vi "ControlProgram5.8.vi"() -> ()   [LabVIEW 2016]
uses:
  <vilib>/Utility/miscctls.llb/LVPoint32TypeDef.ctl
  <vilib>/Platform/TimedLoop/XDataNode/timing_clust.ctl
  <vilib>/Platform/TimedLoop/XDataNode/nitl_modes.ctl
  <vilib>/Platform/TimedLoop/XDataNode/wakeup.ctl
  <vilib>/vision/Avi1.llb/AviRefnum.ctl
  <vilib>/Utility/error.llb/DialogType.ctl
  <vilib>/DAQmx/write.llb/DAQmx Write (Analog 1D DBL NChan 1Samp).vi
  <vilib>/DAQmx/read.llb/DAQmx Read (Analog 2D DBL NChan NSamp).vi
  <vilib>/Analysis/baseanly.llb/Mean (DBL).vi
  <vilib>/DAQmx/write.llb/DAQmx Write (Digital Bool 1Line 1Point).vi
  <vilib>/DAQmx/create/channels.llb/DAQmx Create Channel (DO-Digital Output).vi
  <vilib>/Instr/_visa.llb/VISA Configure Serial Port (Instr).vi
  <vilib>/DAQmx/create/channels.llb/DAQmx Create Channel (AI-Voltage-Basic).vi
  <vilib>/DAQmx/create/channels.llb/DAQmx Create Channel (AO-Voltage-Basic).vi
  <vilib>/DAQmx/configure/timing.llb/DAQmx Timing (Sample Clock).vi
  <vilib>/DAQmx/miscellaneous.llb/DAQmx Fill In Error Info.vi
  <vilib>/Utility/inputDevices.llb/mouseAcquire.vi
  <vilib>/Utility/inputDevices.llb/closeMouse.vi
  <vilib>/platform/TimedLoop/XDataNode/XDataNode.xnode
  <vilib>/Platform/TimedLoop/XDataNode/XDNodeRunTimeDep.lvlib
  <resource>/objmgr/daqmx.rc
  <vilib>/Analysis/NI_AALBase.lvlib
panel:
  out "Primary Video Display":T1(plugin-control)
  in  "Save file index":i32
  out "Flush Sample Start Time":u32=2111292881
  out "Sample flush time (s)":dbl=48.0
  in  "Inject Sample":bool
  out "Chart Freq (Hz)":dbl=500.0
  out "Cal values":T2={"AX alpha"=612.9626061060078, "BX alpha"=549.6584469744151, "AX kappa"=0.3485731373010688, "BX kappa"=0.3853424216291352, "AX offset"=-0.03900484438240665, "BX offset"=-0.11295550662085417, "AY alpha"=582.7562541114835, "BY alpha"=571.1587543790358, "AY kappa"=0.37498408087930674, "BY kappa"=0.36252029651198364, "AY offset"=-0.21125584642206058, "BY offset"=-0.12469077200400738}
  in  "Inject Pump 1":bool
  in  "Inject Pump 2":bool
  in  "Tab Control 2":T3(tab)
  in  "Force FB script":bool
  in  "Got ADig bead":bool
  in  "Move Cap. 2 (ADig Top)":bool
  in  "Dump beads":bool
  in  "Got DNA bead":bool
  in  "Flow on\ncap 2?":bool=TRUE
  in  "Flow on\ncap 1?":bool=TRUE
  in  "Flow on\ndump?":bool=TRUE
  in  "Raster set":i32=1
  in  "Fish After TA?":bool=TRUE
  in  "Delta after tether":dbl=1700.0
  in  "TA Cancel Save?":bool=TRUE
  in  "Min fish\ndelta (nm)":dbl=1425.0 min=0.0 max=5000.0 step=50.0
  in  "Max fish\ndelta (nm)":dbl=1900.0 min=0.0 max=5000.0 step=25.0
  in  "Fish Speed (ms)":i32=5000
  in  "Wait (ms)":i32=1500
  in  "# attempts":dbl=10.0
  in  "Cutoff force (pN)":dbl=4.5
  in  "Raster after\n tether?":bool=TRUE
  out "Tether":bool
  out "Attempt #":i32
  in  "Flow on\nwhile fish?":bool=TRUE
  in  "Flow on\nafter raster?":bool=TRUE
  in  "Offset raster set":i32
  in  "Offset @ Delta (nm)":dbl=1700.0
  in  "Cal @ Delta (nm)":dbl=2500.0
  in  "Cal stage position":i32=3
  out "Cal Final Sampling Rate":dbl=125000.0
  in  "Cal Averaging":i32=1
  in  "Wait before dip (s)":dbl=3.0
  in  "Start dipping after?":bool
  in  "Start trap delta (nm)":dbl=1700.0
  in  "Cancel dwell":bool=TRUE
  in  "Pause dwell":bool
  in  "Return position":dbl=3.0
  in  "Dip duration":dbl=15.0
  in  "Dip position":dbl=4.0
  in  "Dip":bool
  out "Dip time":i32
  in  "Stop":bool=TRUE
  in  "?":T4(tab)
  in  "Cal time (s)":dbl=5.0
  in  "Save N sets":bool
  in  "N sets":i32=200
  out "Cal sets to save":i32=500
  in  "Reset data stream":bool
  out "Buffer Overflow":bool
  out "Stage moving":bool
  in  "Comment":string
  in  "Raster scan":bool
  out "Saving":bool
  in  "Save cal":bool
  in  "Save Data":bool
  in  "Stop saving":bool
  out "Calibrating":bool
  out "Progress":dbl(slide) scale=0.0..100.0
  in  "Read Cal":bool
  in  "Fish":bool
  in  "Averaging Number":i32=1250
  out "Final Sampling Rate":dbl=100.0
  in  "Trap position (V)":cluster{"X":dbl, "Y":dbl}={"X"=3.9042624789680316, "Y"=0.2}
  in  "Trap delta (nm)":dbl=2500.0 min=0.0 max=5000.0 step=50.0
  in  "Fixed X":dbl=1.3
  in  "Fixed Y":dbl=1.8
  in  "Shutter 1 (B)":bool
  in  "Shutter 2 (A)":bool
  in  "Pulling direction":bool
  out "Raster scanning...":bool
  out "Current file name":path=path "D:/data/160111/160111_006.dat"
  in  "AX alpha":dbl=612.9626061060078 format="%#_3p"
  in  "BX alpha":dbl=549.6584469744151 format="%#_3g"
  in  "AX kappa":dbl=0.3485731373010688 format="%#_3g"
  in  "BX kappa":dbl=0.3853424216291352 format="%#_3g"
  in  "AX offset":dbl=-0.03900484438240665 format="%#_3g"
  in  "BX offset":dbl=-0.11295550662085417 format="%#_3g"
  in  "AY alpha":dbl=582.7562541114835 format="%#_3g"
  in  "BY alpha":dbl=571.1587543790358 format="%#_3g"
  in  "AY kappa":dbl=0.37498408087930674 format="%#_3g"
  in  "BY kappa":dbl=0.36252029651198364 format="%#_3g"
  in  "AY offset":dbl=-0.21125584642206058 format="%#_3g"
  in  "BY offset":dbl=-0.12469077200400738 format="%#_3g"
  out "Buffer status":u8(slide) scale=0.0..100.0
  in  "Target":bool
  in  "Set Current\nPos to (0,0,0)":bool
  in  "dump spot":string="Dump beads spot"
  in  "up flow spot":string="Upper flow spot"
  in  "low flow spot":string="Lower flow spot"
  in  "up cap":string="Upper capillary (ADig beads)"
  in  "bottom cap":string="Lower capillary (DNA beads)"
  in  "Move to Position 5":bool
  in  "Set Position 5":bool
  in  "Saved stage positions":dbl[][](array[numeric])=[[1.0, 0.0, 0.0, 0.0], [2.0, -0.13716, -3.21132, 0.01436], [3.0, 0.45, -0.73974, 0.005], [4.0, 0.45, -2.1978, 0.005], [5.0, 0.45, -2.63158, -0.02256]]
  in  "Set Position 2":bool
  in  "Move to Position 2":bool
  in  "Set Position 1":bool
  in  "Move to Position 1":bool
  in  "Set Position 4":bool
  in  "Move to Position 4":bool
  in  "Set Position 3":bool
  in  "Move to Position 3":bool
  out "Stage error":errorcluster
  in  "Clear Volume":bool
  out "Sample Flush Meter":u8(slide) scale=0.0..100.0
  out "Flushing Sample":bool
  in  "Flush Sample":bool
  in  "Normal \nRate (ul/hr)  3":dbl=100.0
  in  "Normal \nVolume (ul) 3":dbl=250.0
  in  "Normal \nVolume (ul) 2":dbl
  in  "Normal \nRate (ul/hr)":dbl
  in  "Normal \nVolume (ul)":dbl
  in  "Flush\nRate (ul/min)":dbl
  in  "Flush\nVolume (ul)":dbl
  in  "Flush \nRate (ul/min)  2":dbl
  in  "Flush Pump 2":bool
  in  "Flush\nVolume (ul)  2":dbl
  in  "Flush Pump 1":bool
  in  "Normal \nRate (ul/hr)  2":dbl
  in  "Write Wait":i32=1000
  in  "Flush \nRate (ul/min)  3":dbl=100.0
  in  "Flush\nVolume (ul)  3":dbl=80.0
  out "error out":errorcluster
  in  "Use Mouse to Move Trap?":bool
  in  "Pause Mouse/Mirror Connection":bool
  out "Reference Voltage":cluster{dbl, dbl}={0.0, -0.0}
  out "Saved voltage":cluster{dbl, dbl}={5.766666666666665, 1.45}
  out "Real Coordinates":cluster{"Horizontal":i32, "Vertical":i32}={"Horizontal"=897, "Vertical"=-1271}
  out "CoordinatesMousePressed":T5
  out "Sum error":dbl(knob) scale=-0.2..0.2
  out "Trap sep":waveform(dbl)[](graph)=[{"t0"=timestamp(4.489999999999949 s since 1904-01-01), "dt"=0.002, "Y"=[-1157.7639781743756, -1157.678951177374, -1157.7582331070425, -1157.7490409992681, -1157.8995617642552], "attributes"=variant("NI_ChannelName"=variant(string "T2 X"))}, {"t0"=timestamp(4.489999999999949 s since 1904-01-01), "dt"=0.002, "Y"=[-909.0775466981794, -909.1316439023619, -909.1322956759037, -909.1570630705896, -909.1264297140281], "attributes"=variant("NI_ChannelName"=variant(string "T2 Y"))}]
  in  "Set reading to\nsetpoint":bool
  in  "Offset Y (nm)":dbl format="%0.2f"
  in  "Offset X (nm)":dbl format="%0.2f"
  in  "Remove offsets":bool
  in  "Force Feedback":bool
  out "Feedback Output Voltage 2":cluster{dbl, dbl} {"?" format="%#_4g"; "?" format="%#_4g"}
  in  "Offset":cluster{"Off Y":dbl, "Off X":dbl}={"Off Y"=1.5, "Off X"=0.17}
  in  "Setpoint voltage":cluster{"SP Y":dbl, "SP X":dbl}={"SP Y"=0.6, "SP X"=0.0}
  in  "Feedback const":T6={"Ki_B_Y"=0.5, "Ki_B_X"=0.0, "Kp Y"=1.0, "Kp X"=0.0}
  out "Mean Trap Pos X 2 (nm)":dbl=-1157.769953044463 format="%0.2f"
  out "Mean Trp Pos Y 2 (nm)":dbl=-909.1249958122125 format="%0.2f"
  out "T2 X RMS (A)":dbl=0.7168002469275427 format="%0.2f"
  out "T2 Y RMS (A)":dbl=0.25997187037503383 format="%0.2f"
  in  "Scan range (nm)":dbl=425.0
  in  "Scan speed (nm/s)":dbl=100.0 min=0.0 max=100.0
  in  "Step size (nm)":dbl=1.0
  in  "Save scans":bool=TRUE
  in  "# scans":i32=1
  in  "Load param":bool
  in  "Scan Parameters":T7(array[cluster])=[{"Label"="Offset", "Scan range 1"=600.0, "Step size 1"=1.0, "Scan speed 1"=100, "# scans 2"=1}, {"Label"="Hairpin", "Scan range 1"=450.0, "Step size 1"=1.0, "Scan speed 1"=100, "# scans 2"=1}]
  in  "Trap delta\nafter (nm)":dbl=1550.0
  in  "Stop raster":bool
  out "Scan range (V)":dbl=0.47672462142456534
  out "Scan steps (mirror)":u64=425
  out "Scan increment (V)":dbl=0.0011217049915872126
  out "Time per step (ms)":dbl=10.0
  out "Total raster time (s)":dbl=8.5
  out "N sets to be saved":dbl=850.0
  in  "Zoom Factor":sgl=7.0
  in  "Center Point":cluster{"X":i32, "Y":i32}={"X"=335, "Y"=271}
  in  "Intensity Upper":dbl=88.0
  in  "Intensity Lower":dbl=66.0
  out "Window Size":cluster{"Height":i32, "Width":i32}
  in  "Image Index":dbl=1.0 min=1.0
  in  "Save Image":bool
  in  "Averaging":bool
  in  "Reset Averaging":bool
  in  "Save Video":bool
  in  "New Video File":bool
  in  "Video Index":dbl=1.0 min=1.0 step=1.0
  in  "Video Capture Rate (Hz)":dbl=30.0
  in  "Initial Window Size":cluster{"Width":i32, "Height":i32}={"Width"=884, "Height"=619}
  in  "Initial Window Position":cluster{"X Position":i32, "Y Position":i32}={"X Position"=796, "Y Position"=4}
  out "Window Position":cluster{"X Position":i32, "Y Position":i32}={"X Position"=40, "Y Position"=40}
  out "Path Out":path
  in  "Target coordinates":cluster{"X1":dbl, "Y1":dbl, "X2":dbl, "Y2":dbl}={"X1"=328.0, "Y1"=274.0, "X2"=368.0, "Y2"=314.0}
  in  "# Samples/channel (in)":i32=40000 format="%.2f"
  out "Buffer size\n(Samples/channel)":u32=511
  out "DAQ rate\n(Samples/s)":dbl=125000.0 format="%#_6p"
  out "# Samples/channel":i32=1250
  out "# Samples/channel/s":dbl=100.0
  out "AvailSampPerChan":u32=9
  out "Data update period (s/set)":dbl=0.01 format="%#_6p"
  out "AvailSampPerChan 2":u32=110
  in  "PC samp per channel":i32=1000
  in  "Sampling Rate":dbl=125000.0 format="%0.0p"
  in  "DAQ Rate2":dbl=1000000.0 format="%#_6p"
  out "Data period (s)":dbl=8e-06 format="%#_6p"
  in  "Save user params":bool
  in  "User":string(combo)
  in  "Load user params":bool
  in  "Tether break\nforce (pN)":dbl=1.0
  in  "Path":path=path "E:/Data"
  out "Mirror task":refnum<k21>
  in  "Conv X (nm/V)":dbl=891.5
  in  "Conv Y (nm/V)":dbl=505.7
  in  "Min value Y":dbl format="%.1g"
  in  "Max value Y":dbl=10.0 format="%.1f"
  in  "Min value X":dbl format="%0.1f"
  in  "Max value X":dbl=10.0 format="%.1f"
  in  "HWP1":string="Half waveplate 1: differential trap power"
  in  "HWP0":string="Half waveplate 0: total trap power"
  in  "Move 1":bool
  in  "\"Degrees\" 1":dbl
  in  "Move 0":bool
  in  "\"Degrees\" 0":dbl
  out "Deflection":T5
  in  "Sampling Rate":dbl=125000.0 format="%0.2f"
  in  "Averaging Number":i32=12500
  in  "DAQ Rate":dbl=1000000.0
  out "Final Sampling Rate":dbl
  in  "Tab Control":T8(tab)
  in  "Downsamp\nfact":dbl=250.0
  out "Bead sep":waveform(dbl)[](graph)=[{"t0"=timestamp(4.489999999999949 s since 1904-01-01), "dt"=0.002, "Y"=[8093.963535945606, 8103.1617772716045, 8385.72390184118, 8245.733099167523, 8154.925676756515], "attributes"=variant("NI_ChannelName"=variant(string "T2"))}, {"t0"=timestamp(4.489999999999949 s since 1904-01-01), "dt"=0.002, "Y"=[1717.924930434114, 1628.723007842151, 1787.6888378897193, 1598.475730715916, 1776.2517588078954], "attributes"=variant("NI_ChannelName"=variant(string "T1"))}]
  out "Force (pN)":waveform(dbl)[](graph)=[{"t0"=timestamp(4.489999999999949 s since 1904-01-01), "dt"=0.002, "Y"=[2821.5994183803123, 2824.8226375853515, 2923.3663028678166, 2874.5254578927593, 2842.869034836209], "attributes"=variant("NI_ChannelName"=variant(string "T2"))}, {"t0"=timestamp(4.489999999999949 s since 1904-01-01), "dt"=0.002, "Y"=[623.5850847499229, 591.0680427774053, 648.761979867749, 579.944408346982, 644.7436619059413], "attributes"=variant("NI_ChannelName"=variant(string "T1"))}]
  out "Mean force (pN)":dbl=1737.5286029210451 format="%0.2f"
  out "Force noise (pN)":dbl=26.83032703631318 format="%0.2f"
  out "Mean Bead Sep\n(nm)":dbl=4949.257225667222 format="%0.2f"
  out "Bead Sep Noise\n(A)":dbl=757.8078481959694 format="%0.2f"
  out "PSD 2":cluster{dbl[], dbl[]}(graph)
  out "PSD 1":cluster{dbl[], dbl[]}(graph)
  out "PSD 1 Sum":dbl(slide) scale=0.0..10.0
  out "PSD 2 Sum":dbl(slide) scale=0.0..10.0
  in  "Start":bool
  out "All signals":waveform(dbl)[](graph)=[{"t0"=timestamp(4.489999999999949 s since 1904-01-01), "dt"=0.002, "Y"=[0.0010396217068286443, 0.0010666908927528754, 0.001103298744846499, 0.0010651440823993424, 0.0010656596859401936], "attributes"=variant("NI_ChannelName"=variant(string "A y"))}, {"t0"=timestamp(4.489999999999949 s since 1904-01-01), "dt"=0.002, "Y"=[0.02000680227246931, 0.020097032918054827, 0.02003412926844257, 0.020136734401221615, 0.020087494249822452], "attributes"=variant("NI_ChannelName"=variant(string "A x"))}, {"t0"=timestamp(4.489999999999949 s since 1904-01-01), "dt"=0.002, "Y"=[-0.0014958587831537804, -0.0015046240440107857, -0.0014930229638311983, -0.001533240041751485, -0.0015262793936602433], "attributes"=variant("NI_ChannelName"=variant(string "B y"))}, {"t0"=timestamp(4.489999999999949 s since 1904-01-01), "dt"=0.002, "Y"=[0.0002901198559372817, 0.0002731049385577592, 0.00026511308349727467, 0.0002517073909711183, 0.0002916666665966012], "attributes"=variant("NI_ChannelName"=variant(string "B x"))}, {"t0"=timestamp(4.489999999999949 s since 1904-01-01), "dt"=0.002, "Y"=[-0.001511556786147372, -0.0015167122027053212, -0.0014612914746018214, -0.0014935128282145193, -0.0015064013696263116], "attributes"=variant("NI_ChannelName"=variant(string "A sum"))}, {"t0"=timestamp(4.489999999999949 s since 1904-01-01), "dt"=0.002, "Y"=[-0.0005242945138364382, -0.0005565158674093218, -0.000501095139248956, -0.0005771375336978897, -0.0005165613890095197], "attributes"=variant("NI_ChannelName"=variant(string "B sum"))}, {"t0"=timestamp(4.489999999999949 s since 1904-01-01), "dt"=0.002, "Y"=[0.0013303666019343777, 0.0014257418088905328, 0.0013368108726387405, 0.0013471217058124534, 0.0011782818123890176], "attributes"=variant("NI_ChannelName"=variant(string "Trap x"))}, {"t0"=timestamp(4.489999999999949 s since 1904-01-01), "dt"=0.002, "Y"=[0.0023382505474007294, 0.002231275652833831, 0.002229986798687363, 0.0021810103409340116, 0.002241586486003531], "attributes"=variant("NI_ChannelName"=variant(string "Trap y"))}]
  # "Bead Calibration"
  # "Y"
  # "X"
  # "Pump #1 Controls"
  # "Pump #2 Controls"
  # "Sample Pump Controls"
  # "Retract the pumps manually. Change it back to INFUSE when you're done. Suck it up, don't whine."
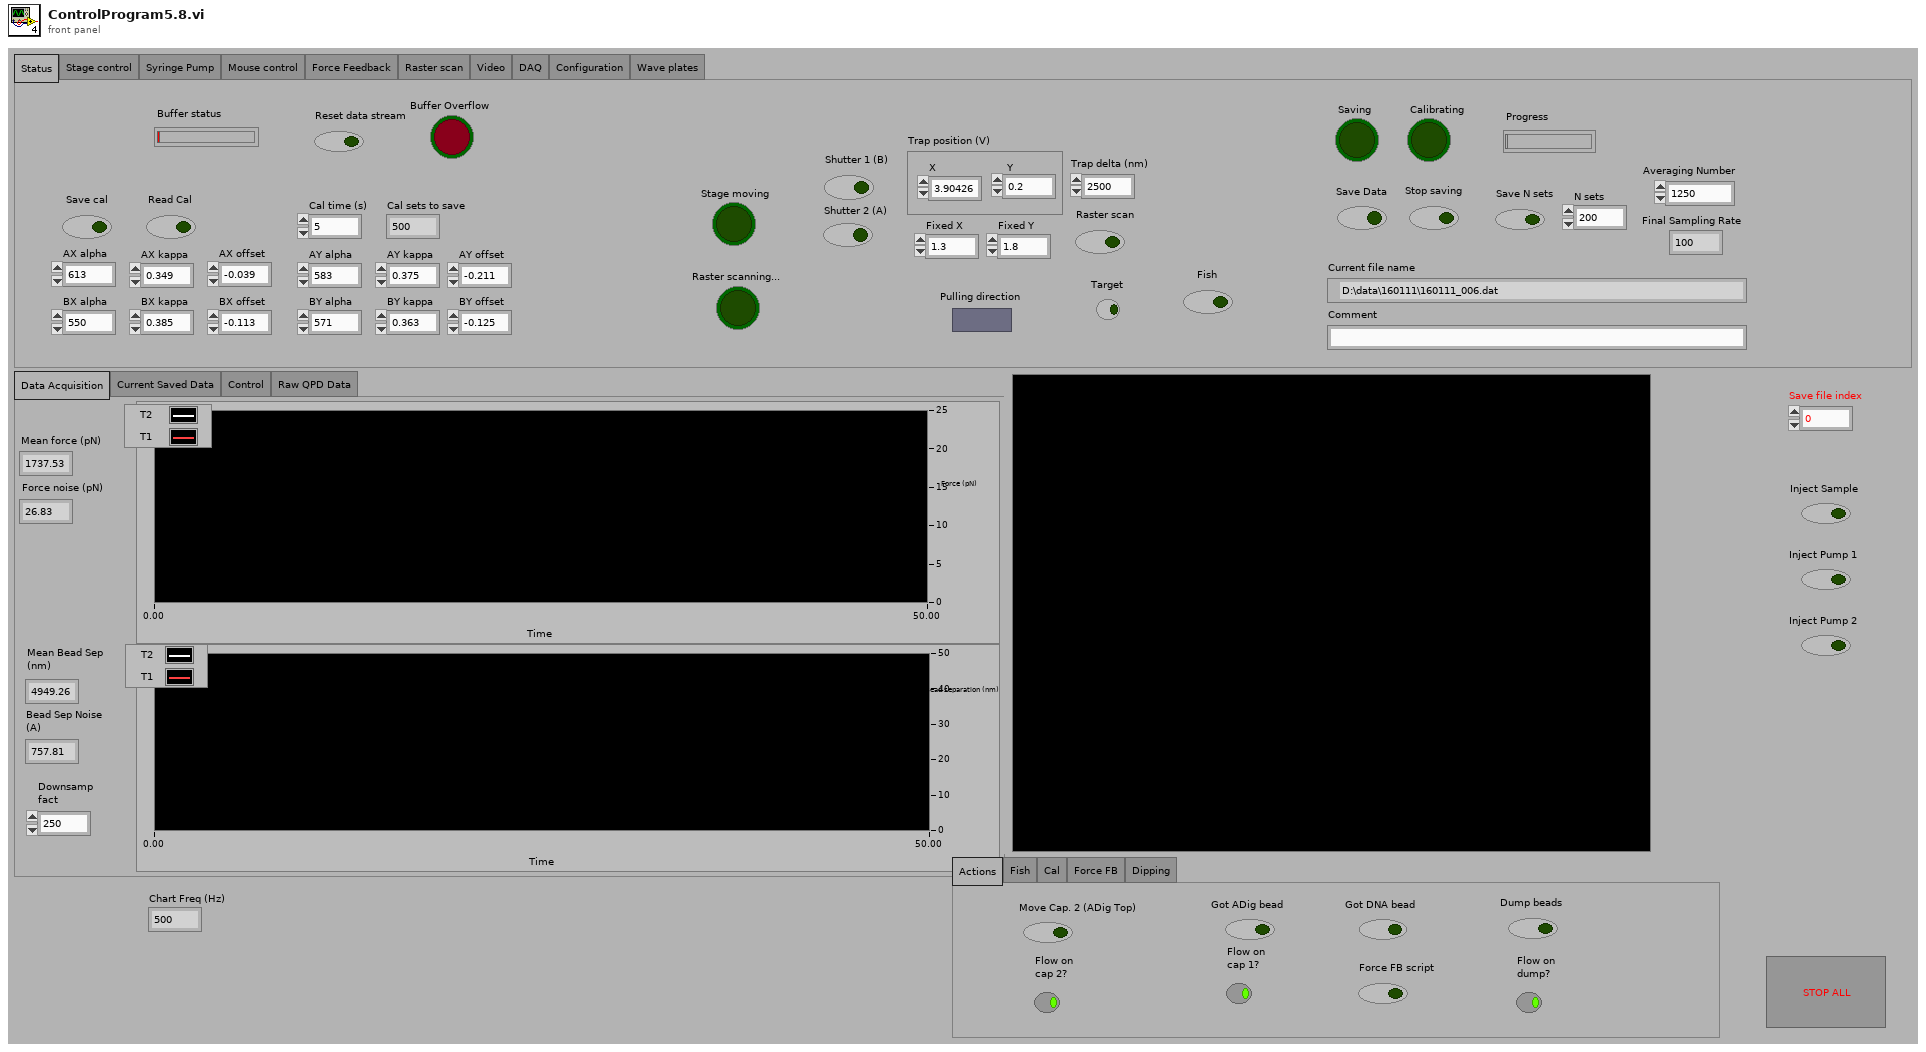
[diagram p1: front panel]
types:
  T1 = typedef "IMAQ Image.ctl" = refnum<image>
  T2 = cluster{"AX alpha":dbl, "BX alpha":dbl, "AX kappa":dbl, "BX kappa":dbl, "AX offset":dbl, "BX offset":dbl, "AY alpha":dbl, "BY alpha":dbl, "AY kappa":dbl, "BY kappa":dbl, "AY offset":dbl, "BY offset":dbl}
  T3 = enum32{"Actions", "Fish", "Cal", "Force FB", "Dipping"}
  T4 = enum32{"Status", "Stage control", "Syringe Pump", "Mouse control", "Force Feedback", "Raster scan", "Video", "DAQ", "Configuration", "Wave plates"}
  T5 = typedef "LVPoint32TypeDef.ctl" = cluster{"Horizontal":i32, "Vertical":i32}
  T6 = cluster{"Ki_B_Y":dbl, "Ki_B_X":dbl, "Kp Y":dbl, "Kp X":dbl}
  T7 = cluster{"Label":string, "Scan range 1":dbl, "Step size 1":dbl, "Scan speed 1":i32, "# scans 2":i32}[]
  T8 = enum32{"Data Acquisition", "Current Saved Data", "Control", "Raw QPD Data"}
  T9 = enum32{"setting", "request", "request control", "info", "statistics", "system settings", "I/O sub system", "HRT control", "camera descriptions", "device specific data", "event sub system settings", "event sub system results", "image memory manager"}
  T10 = typedef "AviRefnum.ctl" = refnum<k1>
  T11 = typedef "XDNodeRunTimeDep.lvlib/timing_clust.ctl" = cluster{"Expected End [f-1]":u64, "Actual End [f-1]":u64, "Finished Late? [f-1]":bool, "Expected End [i-1]":u64, "Actual End [i-1]":u64, "Finished Late? [i-1]":bool, "Expected Start [i]":u64, "Actual Start [i]":u64, "Expected Start [f]":u64, "Actual Start [f]":u64, "Source Name":string, "Structure Name":string, "Period":i64, "Deadline":i64, "Offset":i64, "Start":i64, "Priority":i32, "Timeout":i32, "Mode":T12, "Wakeup Reason":T13, "Error":errorcluster, "Source Type":string, "Secondary Source Type":string, "Global End Time":u64, "Global Start Time":u64, "Frame Duration":u64, "Iteration Duration":u64, "Assigned CPU":i32, "I/O Scan Engine Mode":u32}
  T12 = typedef "XDNodeRunTimeDep.lvlib/nitl_modes.ctl" = enum32{"No Change", "Process missed periods, maintain original phase", "Discard missed periods, maintain original phase", "Process missed periods, ignore original phase", "Discard missed periods, ignore original phase"}
  T13 = typedef "XDNodeRunTimeDep.lvlib/wakeup.ctl" = enum32{"Normal", "Aborted", "Asynchronous wakeup", "Timing source error", "Timed loop error", "Timeout"}
  T14 = typedef "Image Type" = u32
  T15 = typedef "imagedata.ctl" = cluster{"image type":i32, "image depth":i32, "image":u8[], "mask":u8[], "colors":u32[], "Rectangle":cluster{"left":i16, "top":i16, "right":i16, "bottom":i16}}
  T16 = enum16{"open", "replace", "create", "open or create", "replace or create", "replace or create with confirmation"}
  T17 = enum16{"big-endian, network order", "native, host order", "little-endian"}
  T18 = cluster{string, string, string, string, string, string, string, string}
  T19 = typedef "DialogType.ctl" = u16
  T20 = cluster{"button 1":bool, "button 2":bool, "button 3":bool, "button 4":bool}
  T21 = cluster{"[0]":dbl, "[1]":dbl, "[2]":dbl, "[3]":dbl, "[4]":dbl, "[5]":dbl, "[6]":dbl, "[7]":dbl, "[8]":dbl, "[9]":dbl, "[10]":dbl, "[11]":dbl}
  T22 = cluster{"Label":string, "Scan range 1":dbl, "Step size 1":dbl, "Scan speed 1":i32, "# scans 2":i32}
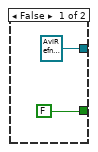
[diagram p2: hidden frame]
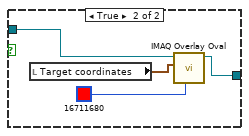
[diagram p5: hidden frame]
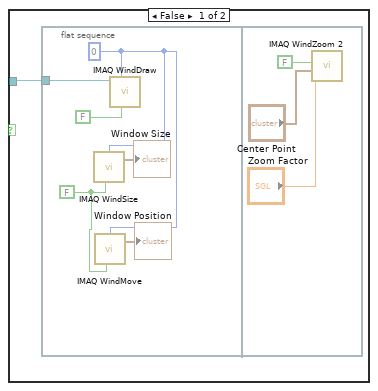
[diagram p6: hidden frame]
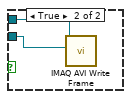
[diagram p8: hidden frame]
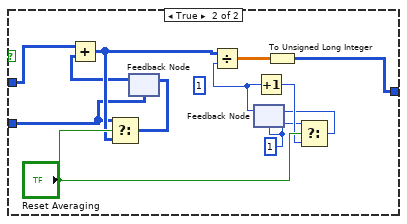
[diagram p9: hidden frame]
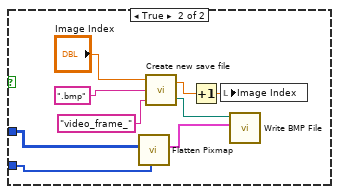
[diagram p10: hidden frame]
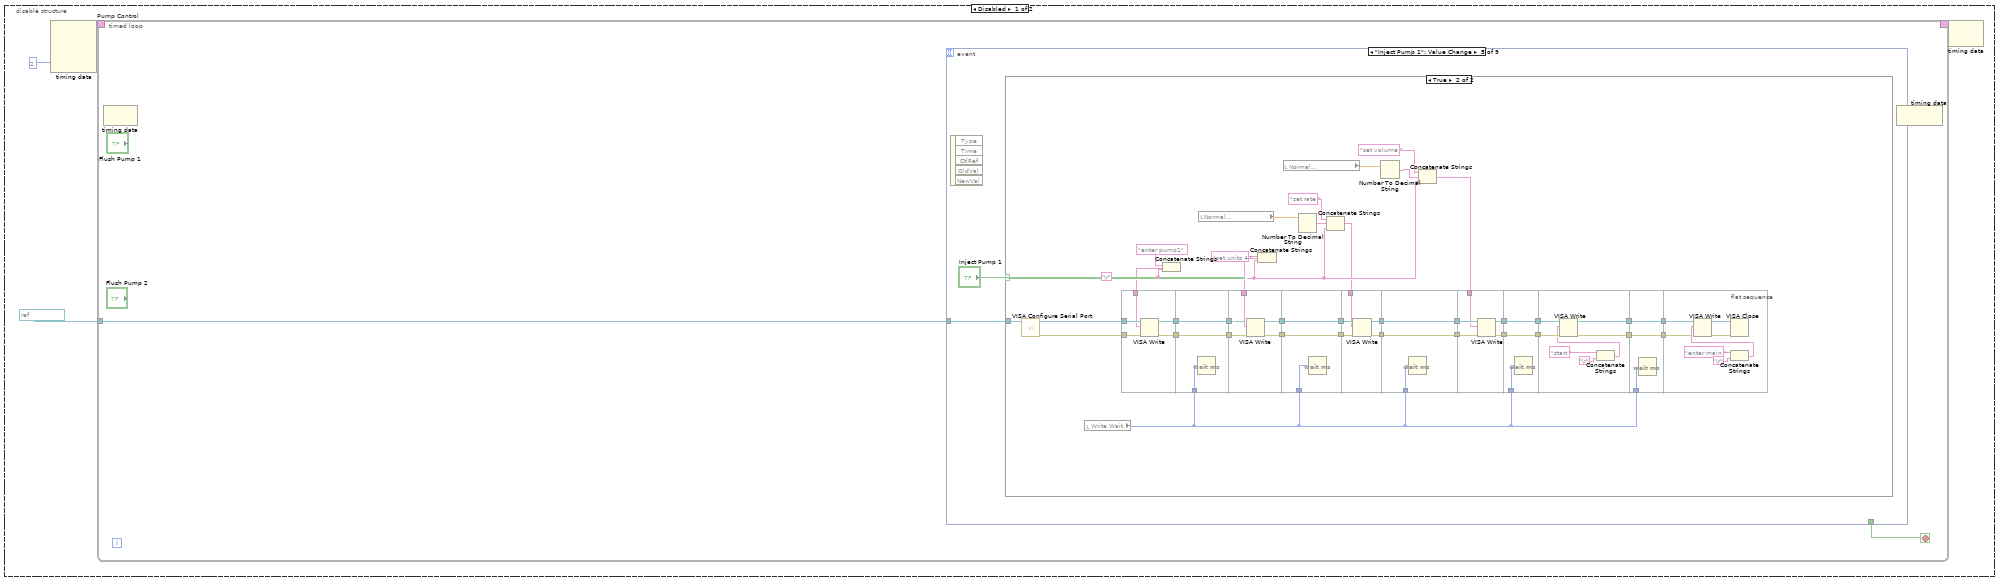
[diagram p11: hidden frame]
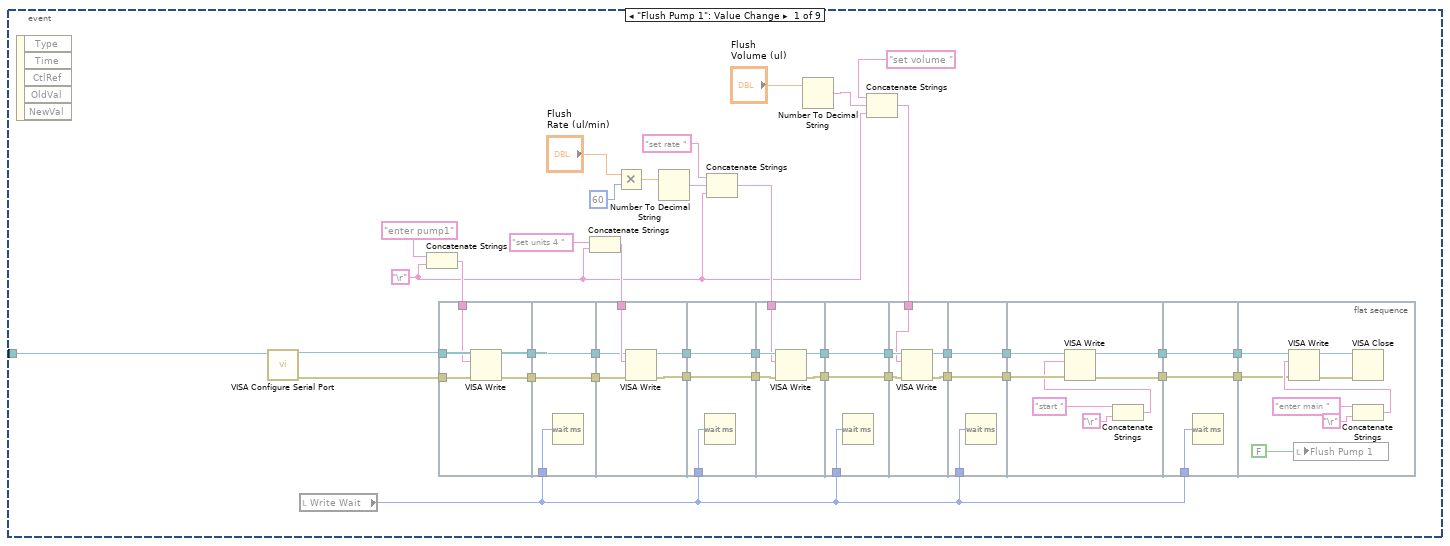
[diagram p12: hidden frame]
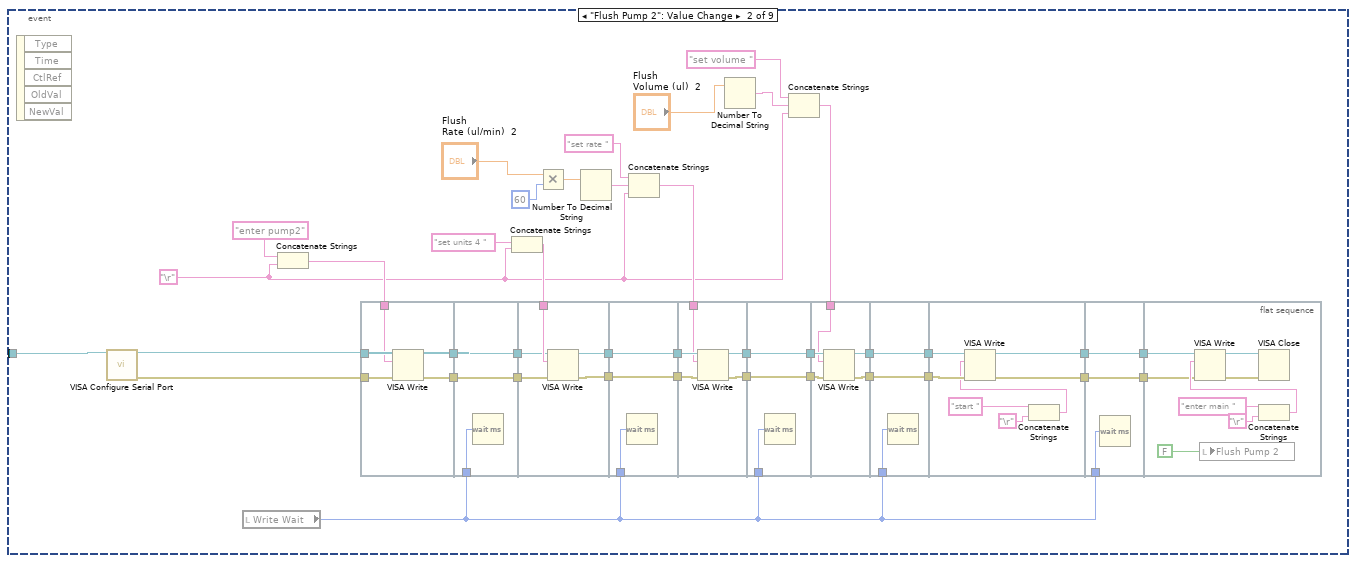
[diagram p13: hidden frame]
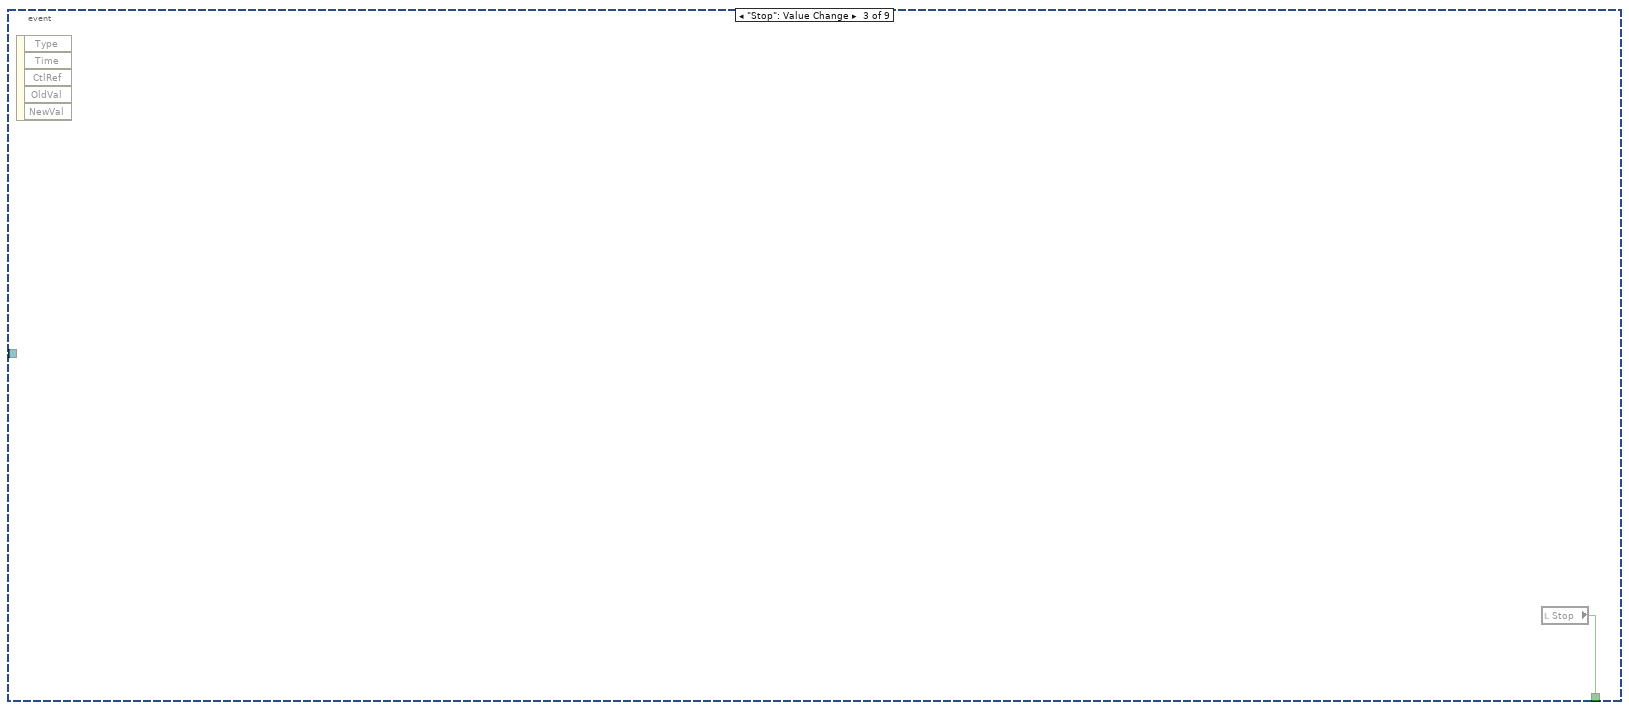
[diagram p14: hidden frame]
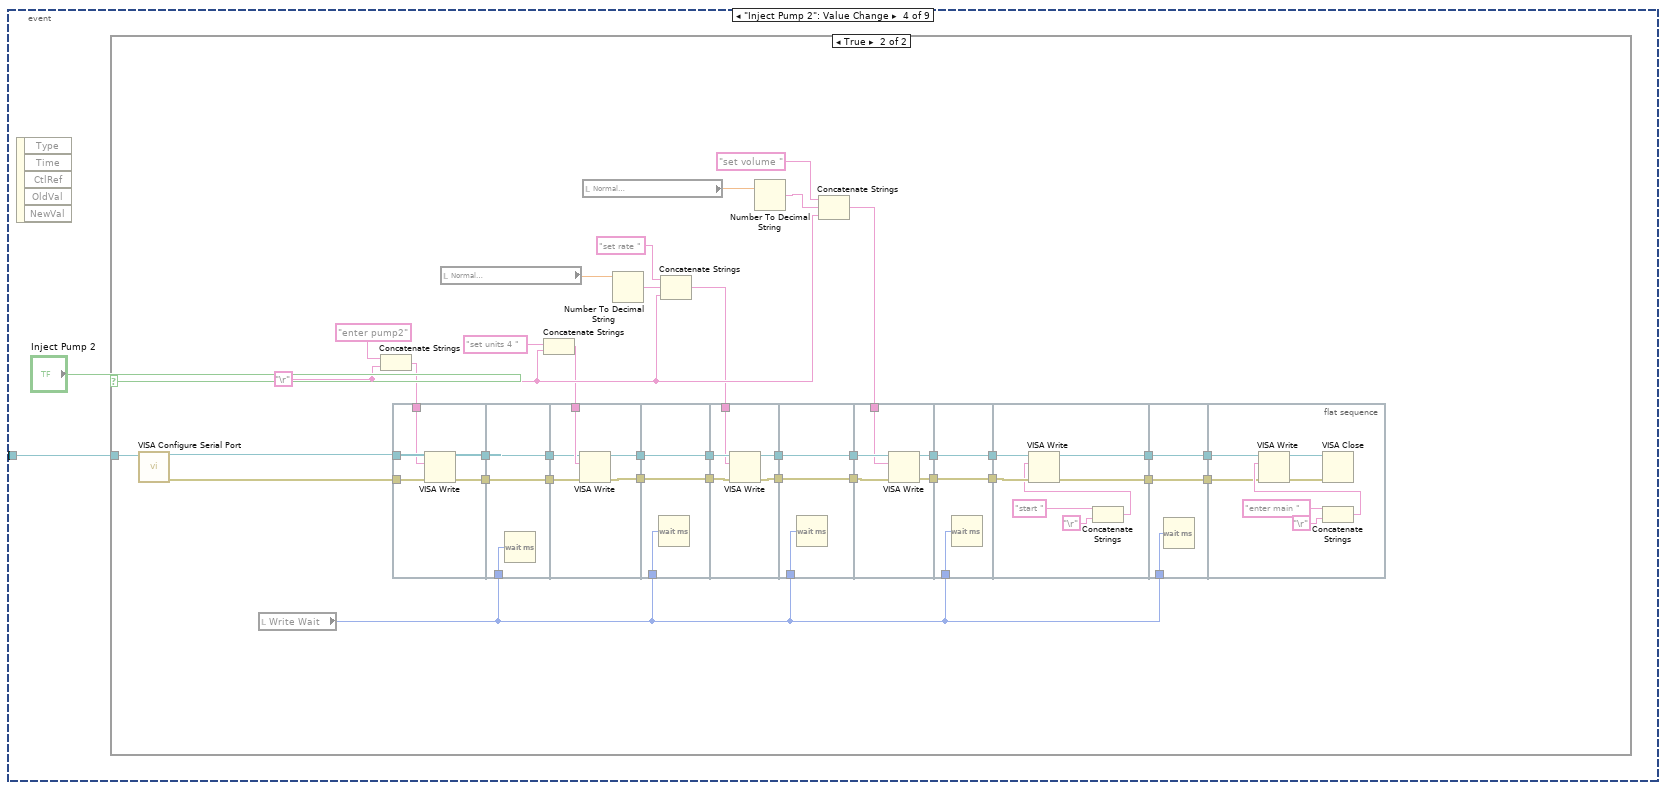
[diagram p15: hidden frame]
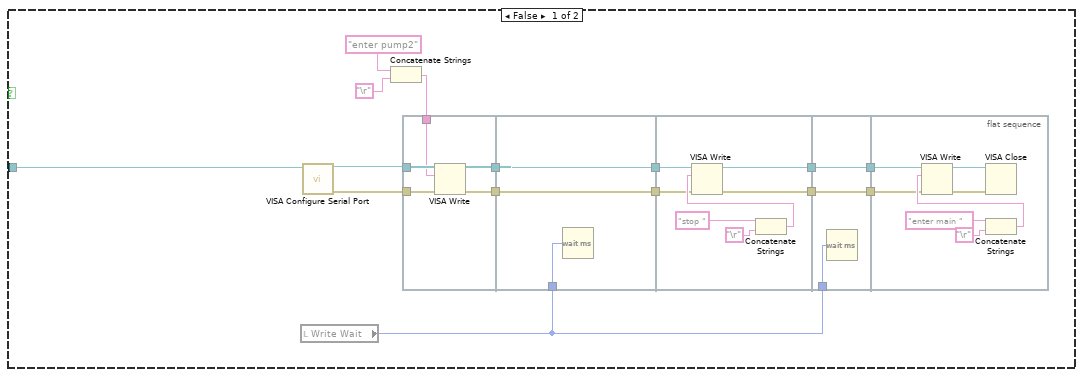
[diagram p16: hidden frame]
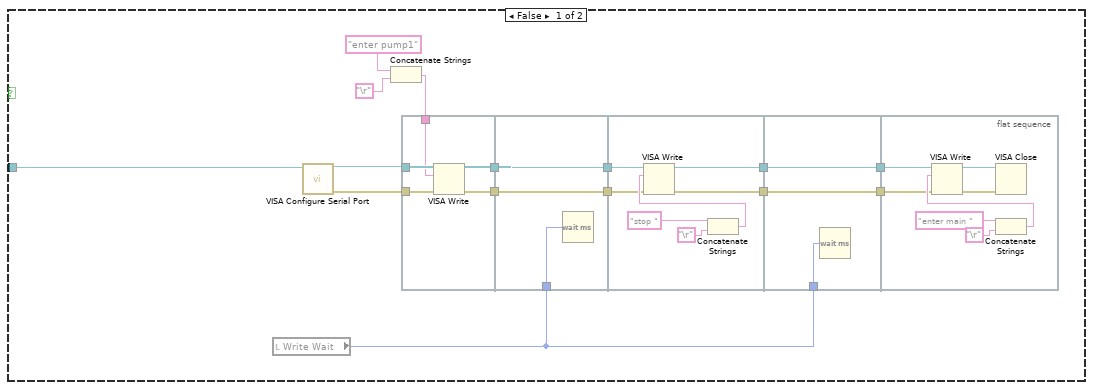
[diagram p17: hidden frame]
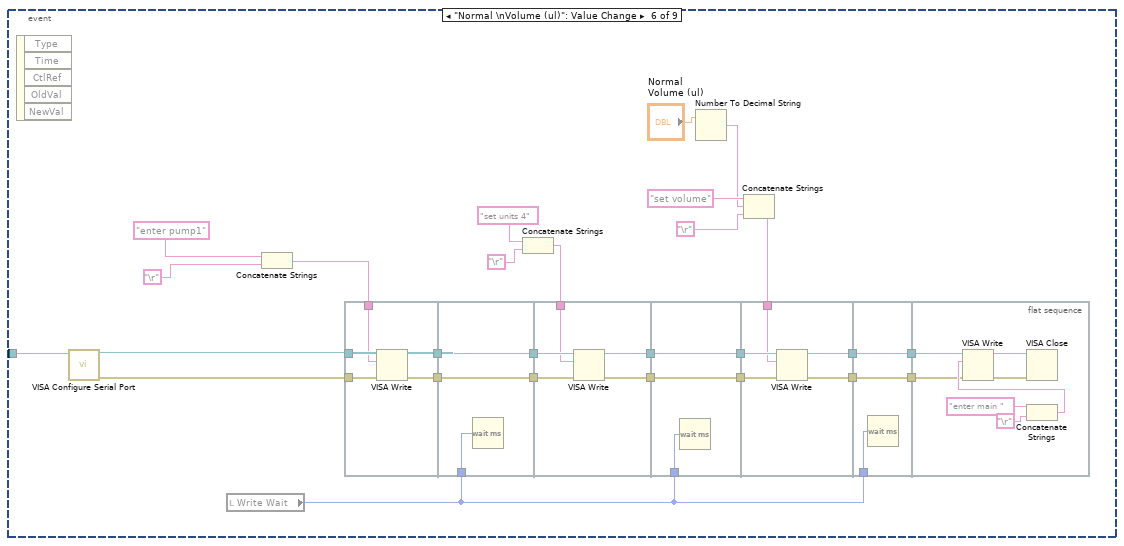
[diagram p18: hidden frame]
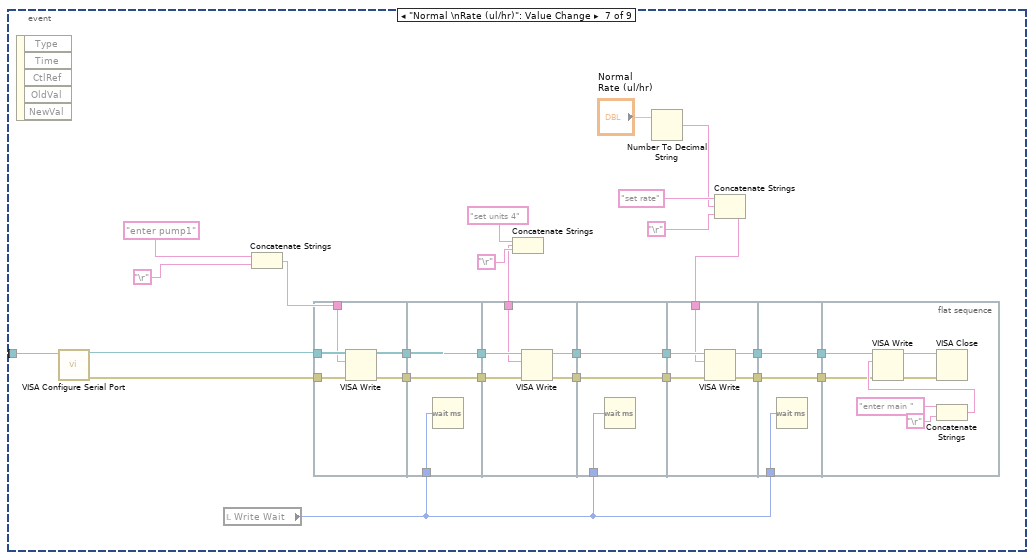
[diagram p19: hidden frame]
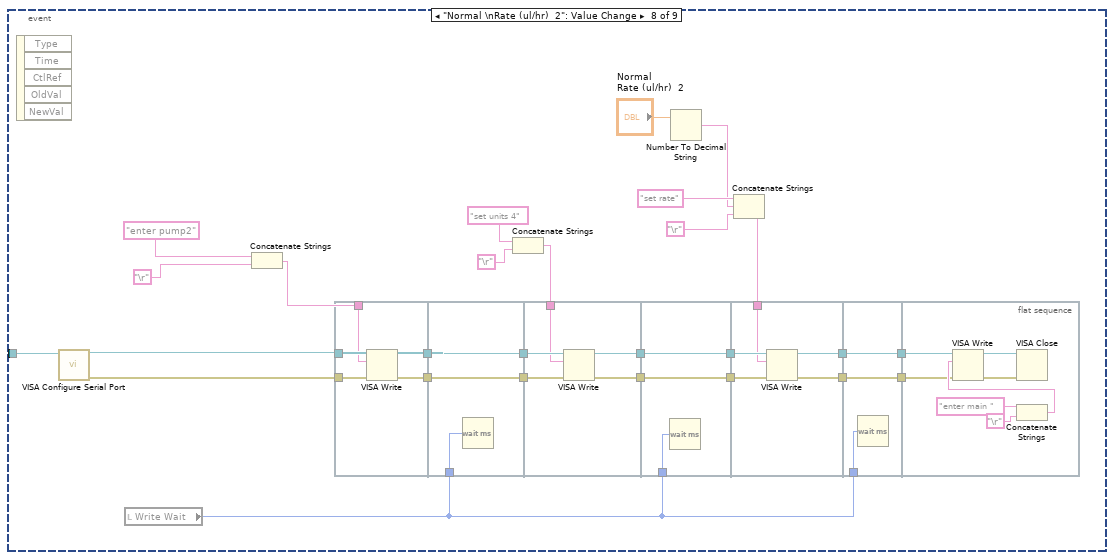
[diagram p20: hidden frame]
diagram:
  w38 = 10.0 ("Minimum Value")
  w39 = -10.0 ("Minimum Value")
  w41 = -2.0 ("Minimum Value")
  w42 = 2.0 ("Maximum Value")
  w67 = 10123 items=["Finite Samples"=10178, "Continuous Samples"=10123] ("sample mode")
  w88 = tag "Dev1/port2/line1"  # Shutter 2
  w91 = tag "Dev1/port1/line4"  # Shutter 1
  # "Create channels for movable mirror"
  # "Create channels for detectors"
  n1 = call-poly <vilib>:"DAQmx Create Virtual Channel.vi"("maximum value"=w42, "minimum value"=w41, "physical channels"=tag "Dev1/ai0" ("Physical Channel")) -> ("task out"=w43:refnum<k21>, "error out"=w66:errorcluster)  [unwired: 11 in]
  n2 = call-poly <vilib>:"DAQmx Create Virtual Channel.vi"("task in"=w43, "maximum value"=w42, "minimum value"=w41, "physical channels"=tag "Dev1/ai1", "error in"=w66) -> ("task out"=w64:refnum<k21>, "error out"=w63:errorcluster)  [unwired: 9 in]
  n3 = call-poly <vilib>:"DAQmx Create Virtual Channel.vi"("task in"=w64, "maximum value"=w42, "minimum value"=w41, "physical channels"=tag "Dev1/ai2", "error in"=w63) -> ("task out"=w55:refnum<k21>, "error out"=w54:errorcluster)  [unwired: 9 in]
  n4 = call-poly <vilib>:"DAQmx Create Virtual Channel.vi"("task in"=w55, "maximum value"=w42, "minimum value"=w41, "physical channels"=tag "Dev1/ai3" ("Physical Channel"), "error in"=w54) -> ("task out"=w40:refnum<k21>, "error out"=w60:errorcluster)  [unwired: 9 in]
  n5 = call-poly <vilib>:"DAQmx Create Virtual Channel.vi"("task in"=w40, "maximum value"=w38, "minimum value"=w39, "physical channels"=tag "Dev1/ai4", "error in"=w60) -> ("task out"=w58:refnum<k21>, "error out"=w57:errorcluster)  [unwired: 9 in]
  n6 = call-poly <vilib>:"DAQmx Create Virtual Channel.vi"("task in"=w58, "maximum value"=w38, "minimum value"=w39, "physical channels"=tag "Dev1/ai5", "error in"=w57) -> ("task out"=w53:refnum<k21>, "error out"=w52:errorcluster)  [unwired: 9 in]
  n7 = call-poly <vilib>:"DAQmx Create Virtual Channel.vi"("task in"=w53, "maximum value"=w38, "minimum value"=w39, "physical channels"=tag "Dev1/ai6", "error in"=w52) -> ("task out"=w47:refnum<k21>, "error out"=w45:errorcluster)  [unwired: 9 in]
  n8 = call-poly <vilib>:"DAQmx Create Virtual Channel.vi"("task in"=w47, "maximum value"=w38, "minimum value"=w39, "physical channels"=tag "Dev1/ai7", "error in"=w45) -> ("task out"=w46:refnum<k21>, "error out"=w44:errorcluster)  [unwired: 9 in]
  n9 = call-poly <vilib>:"DAQmx Timing.vi"("task/channels in"=w46, "sample mode"=w67, "samples per channel"="PC samp per channel", "rate"="Sampling Rate", "error in"=w44) -> ("task out"=w50:refnum<k21>, "error out"=w49:errorcluster)  [unwired: 9 in]
  n10 = call-poly <vilib>:"DAQmx Create Virtual Channel.vi"("maximum value"="Max value Y", "minimum value"="Min value Y", "physical channels"=tag "Dev1/ao1" ("Trap X Axis")) -> ("task out"=w35:refnum<k21>, "error out"=w37:errorcluster)  [unwired: 11 in]
  n11 = property class="DAQmx Timing"(reference=w50, error in=w49, "More:AI Convert:Rate"="DAQ Rate2") -> (reference out=w7:refnum<k21>, error out=w6:errorcluster, "SampClk.Rate"=→"DAQ rate\n(Samples/s)":dbl)
  n12 = call-poly <vilib>:"DAQmx Create Virtual Channel.vi"("task in"=w35, "maximum value"="Max value X", "minimum value"="Min value X", "physical channels"=tag "Dev1/ao0" ("Trap Y Axis"), "error in"=w37) -> ("task out"=w26:refnum<k21>, "error out"=w25:errorcluster)  [unwired: 9 in]
  "Mirror task" <- w26
  n13 = property class="DAQmx Buffer"(reference=w7, error in=w6) -> (reference out=w4:refnum<k21>, error out=w3:errorcluster, "Input.OnbrdBufSize"=→"Buffer size\n(Samples/channel)":u32)
  n14 = call <vilib>:"DAQmx Start Task.vi"("task/channels in"=w4, "error in"=w3) -> ("task out"=w27:refnum<k21>)  [unwired: 12 in, 1 out]
  n15 = flat-sequence "Video" {
    tunnel: [w104] -> w1
    tunnel: w1 -> [w145]
    frame #0 {
      n16 = while {
        stop <- w97 continue-if-true
        n17 = call "Close Video Capture.vi"() -> ("error code OUT"=w99:i32)
        n18 = Equal?(x=w99, y=0) -> (x = y?=w97:bool)
      }
      n19 = local write "Stop"(FALSE ("Stop All")) -> ()
    }
    frame #1 {
      n20 = call "DMR_Init.vi"() -> ()  [unwired: 3 out]
    }
    frame #2 {
      # "Setting the destination format to Mono8 makes sure that the image can be displayed in the intensity plot."
      n21 = call "DMR_GetDevice.vi"("search string IN"="DE514724602") -> ("device handle OUT"=w122:i32)  [unwired: 4 in, 2 out]
      n22 = call "DMR_OpenDevice.vi"("device handle IN"=w122) -> ("driver handle OUT"=w105:i32)  [unwired: 4 out]
      n23 = call "DMR_FindList.vi"("flags IN"=u32 0 ("flags"), "list name IN"="" ("String"), "list type IN"=T9."camera descriptions", "driver handle IN"=w105) -> ("list handle OUT"=w108:i32)  [unwired: 2 out]
      n24 = call "DMR_FindList.vi"("flags IN"=u32 0 ("flags"), "list name IN"="Base", "list type IN"=T9."setting", "driver handle IN"=w105) -> ("list handle OUT"=w106:i32)  [unwired: 2 out]
      n25 = call "OBJ_GetHandle.vi"("object name IN"="VideoStandard", "list handle IN"=w108) -> ("object handle OUT"=w102:i32)  [unwired: 3 out]
      n26 = call "OBJ_GetHandle.vi"("object name IN"="PixelFormat", "list handle IN"=w106) -> ("object handle OUT"=w116:i32)  [unwired: 3 out]
      n27 = call "OBJ_SetS.vi"("value index IN"=0, "value IN"="NTSC M", "object handle IN"=w102) -> ()  [unwired: 2 out]
      n28 = call "OBJ_SetS.vi"("value index IN"=0, "value IN"="Mono8" ("value"), "object handle IN"=w116) -> ()  [unwired: 2 out]
      n29 = call "OBJ_GetHandle.vi"("object name IN"="VideoChannel", "list handle IN"=w106) -> ("object handle OUT"=w112:i32)  [unwired: 3 out]
      n30 = while {
        tunnel: [w127] -> w104
        tunnel: w105 -> [w124]
        stop <- w125 continue-if-true
        n31 = call "DMR_ImageRequestSingle.vi"("request control IN"=0, "driver handle IN"=w124) -> ("error code OUT"=w126:i32, "driver handle OUT"=w127:i32)  [unwired: 2 out]
        n32 = Equal To 0?(x=w126) -> (x = 0?=w125:bool)
      }
      n33 = call "OBJ_SetI.vi"("value index IN"=0, "value IN"=0 ("Video channel"), "object handle IN"=w112) -> ()  [unwired: 2 out]
    }
    frame #3 {
      w133 = T14 0 items=["Grayscale (U8)", "Grayscale (I16)", "Grayscale (SGL)", "Complex (CSG)", "RGB (U32)", "HSL (U32)", "RGB (U64)"] ("Image Type")
      w141 = T14 0 items=["Grayscale (U8)", "Grayscale (I16)", "Grayscale (SGL)", "Complex (CSG)", "RGB (U32)", "HSL (U32)", "RGB (U64)"] ("Image Type")
      n34 = for "Create Greyscale map" {
        N: 256 -> [_]
        tunnel: [w147] -> w130 mode=indexing
        workers-P: _ -> [_]
        i -> [w150]
        n35 = To Unsigned Byte Integer(number=w150) -> (unsigned 8bit integer=w146:u8)
        n36 = Join Numbers(hi=w146, lo=w146) -> ((hi.lo)=w149:u16)
        n37 = Join Numbers(hi=w146, lo=w146) -> ((hi.lo)=w148:u16)
        n38 = Join Numbers(hi=w149, lo=w148) -> ((hi.lo)=w147:u32)
      }
      n39 = call "IMAQ Create"("Image Name"="Scaled video", "Image Type"=w133) -> ("New Image"=w132:T1)  [unwired: 2 in, 2 out]
      n40 = call "IMAQ Create"("Image Name"="Main video", "Image Type"=w141) -> ("New Image"=w142:T1)  [unwired: 2 in, 2 out]
      n41 = node-c288(0 ("Processor")) -> (w140:T11)  [unwired: 3 out]
      n42 = Initialize Array(u32 0 ("Window Number (0...15)"), 480 ("dimension size"), 640 ("dimension size")) -> (w135:u32[][])
      n43 = timed-loop {
        tunnel: w145 -> [w167]
        tunnel: [w166] -> w144
        tunnel: w142 -> [w165]
        timing: w140 -> [_]
        timing-out: [_] -> w139
        tunnel: w135 -> [w154]
        tunnel: w132 -> [w152]
        tunnel: w130 -> [w151]
        stop <- w153 stop-if-true
        # "This block performs the \nactual image capture."
        n44 = node-c288() -> ()  [unwired: 2 out]
        n45 = local read "Stop"() -> (w153:bool)
        n46 = Reciprocal(x="Video Capture Rate (Hz)") -> (1/x=w157:dbl)
        n47 = Multiply(x=w157, y=1000.0) -> (x*y=w155:dbl)
        n48 = call "DMR_ImageRequestWaitFor.vi"("queue number IN"=0, "timeout(ms) IN"=500, "driver handle IN"=w167) -> ("error code OUT"=w171:i32, "request number OUT"=w168:i32, "driver handle OUT"=w169:i32)
        n49 = feedback #1(T10 refnum ("Avi Refnum")) -> (w159:T10)
        n50 = case shown="True" "New Video File" {
          tunnel: [T10 refnum ("Avi Refnum") w188] -> w161
          tunnel: [FALSE TRUE] -> w162
          tunnel: w159 -> [_ w184]
          frame False {
          }
          frame True {
            n51 = call "Create new save file.vi"("Ext"=".avi" ("string"), "Index In"="Video Index") -> ("Path Out"=w180:path, "Index Out"=w181:dbl)  [unwired: 1 in]
            "Path Out" <- w180
            n52 = Not Equal?(x=w184, y=T10 refnum ("Avi Refnum")) -> (x != y?=w185:bool)
            n53 = Increment(x=w181) -> (x+1=w190:dbl)
            n54 = case shown="True" w185 {
              tunnel: w184 -> [_ w191]
              frame False {
              }
              frame True {
                n55 = call "IMAQ AVI Close"("Avi Refnum"=w191) -> ()  [unwired: 1 in, 10 out]
              }
            }
            n56 = local write "Video Index"(w190) -> ()
            n57 = call "IMAQ AVI Create"("Frames Per Second"=u32 30, "AVI Path"=w180) -> ("Avi Refnum"=w188:T10)  [unwired: 5 in, 4 out]
          }
        }
        n58 = Equal To 0?(x=w171) -> (x = 0?=w170:bool)
        n59 = Select(t=w161, s=w162, f=w159) -> (s? t:f=w160:T10)
        n60 = feedback-in #1(w160) -> ()
        n61 = case shown="True" w170 {
          tunnel: w169 -> [w192 w219]
          tunnel: w168 -> [_ w218]
          tunnel: [w192 w215] -> w166
          tunnel: w165 -> [_ w196]
          tunnel: w154 -> [_ w203]
          tunnel: w160 -> [_ w201]
          tunnel: w152 -> [_ w197]
          tunnel: w151 -> [_ w198]
          frame False {
          }
          frame True {
            w209 = u32 0 ("X-offset IN")
            n62 = call "DMR_GetImageRequestBufferData.vi"("driver handle IN"=w219, "request number IN"=w218) -> ("width OUT"=w208:i32, "height OUT"=w207:i32, "driver handle OUT"=w214:i32, "request number OUT"=w213:i32, "bytes per pixel OUT"=w210:i32)  [unwired: 13 out]
            n63 = call "DMR_GetImageRequestBufferImageData.vi"("driver handle IN"=w214, "request number IN"=w213, "bytes per pixel IN"=w210, "X-offset IN"=w209, "Y-offset IN"=w209, "height IN"=w207, "width IN"=w208) -> ("driver handle OUT"=w212:u32, "request number OUT"=w211:u32, "image OUT"=w204:u32[][])  [unwired: 10 out]
            n64 = call "DMR_ImageRequestUnlock.vi"("request number IN"=w211, "driver handle IN"=w212) -> ("driver handle OUT"=w217:i32)  [unwired: 1 in, 2 out]
            n65 = case shown="False" "Averaging" {
              tunnel: w204 -> [w260 w265]
              tunnel: [w260 w264] -> w200
              tunnel: w203 -> [_ w262]
              frame False {
              }
              frame True {
                (unwired) 1
                w270 = 1
                n66 = feedback #2(w262) -> (w261:u32[][])
                n67 = Add(x=w265, y=w261) -> (x+y=w266:u32[][])
                n68 = Select(t=w262, s="Reset Averaging", f=w266) -> (s? t:f=w268:u32[][])
                n69 = feedback-in #2(w268) -> ()
                n70 = feedback #3(w270) -> (w263:i32)
                n71 = Divide(x=w266, y=w263) -> (x/y=w267:dbl[][])
                n72 = Increment(x=w263) -> (x+1=w271:i32)
                n73 = To Unsigned Long Integer(number=w267) -> (unsigned 32bit integer=w264:u32[][])
                n74 = Select(t=w270, s="Reset Averaging", f=w271) -> (s? t:f=w269:i32)
                n75 = feedback-in #3(w269) -> ()
              }
            }
            n76 = call "DMR_ImageRequestSingle.vi"("request control IN"=0, "driver handle IN"=w217) -> ("driver handle OUT"=w215:i32)  [unwired: 3 out]
            n77 = disable-structure shown="Disabled" {
              disable-tunnel: w200 -> [w237 _]
              disable-tunnel: w197 -> [w236 _]
              frame Disabled {
                n78 = To Double Precision Float(number=w237) -> (double precision float=w235:dbl[][])
                n79 = In Range and Coerce(upper limit="Intensity Upper", x=w235, lower limit="Intensity Lower") -> (coerced(x)=w234:dbl[][])  [unwired: 1 out]
                n80 = Subtract(x="Intensity Upper", y="Intensity Lower") -> (x-y=w231:dbl)
                n81 = Subtract(x=w234, y="Intensity Lower") -> (x-y=w232:dbl[][])
                n82 = Divide(x=w232, y=w231) -> (x/y=w233:dbl[][])
                n83 = Multiply(x=255.0, y=w233) -> (x*y=w229:dbl[][])
                n84 = To Unsigned Byte Integer(number=w229) -> (unsigned 8bit integer=w238:u8[][])
                n85 = call "IMAQ ArrayToImage"("Image Pixels (U8)"=w238, "Image"=w236) -> ("Image Out"=w225:T1)  [unwired: 4 in, 5 out]
                n86 = First Call?() -> (First Call?: T/F=w226:bool)
                n87 = case shown="True" w226 {
                  tunnel: w225 -> [w239 w250]
                  frame False {
                    n88 = flat-sequence {
                      tunnel: w239 -> [w245]
                      frame #0 {
                        w242 = FALSE ("Get/Set Status? (Set)")
                        w241 = 0 ("Window Number (0...15)")
                        n89 = call "IMAQ WindSize"("Get/Set Status? (Set)"=w242, "Window Number"=w241) -> ("Width & Height out"=→"Window Size":cluster{"Width":i32, "Height":i32})  [unwired: 4 in, 2 out]
                        n90 = call "IMAQ WindMove"("Window Number (0...15)"=w241, "Get/Set Status? (Set)"=w242) -> ("Coordinates (screen)"=→"Window Position":cluster{"X Position":i32, "Y Position":i32})  [unwired: 3 in, 1 out]
                        n91 = call "IMAQ WindDraw"("Resize to Image Size? (Y)"=FALSE, "Window Number (0...15)"=w241, "Image"=w245) -> ()  [unwired: 7 in, 2 out]
                      }
                      frame #1 {
                        n92 = call "IMAQ WindZoom 2"("Center Point"="Center Point", "Zoom to Fit? (False)"=FALSE, "Zoom Factor"="Zoom Factor") -> ()  [unwired: 5 in, 4 out]
                      }
                    }
                  }
                  frame True {
                    n93 = flat-sequence {
                      tunnel: w250 -> [w253]
                      tunnel: [w251] -> w249
                      tunnel: w249 -> [w255]
                      frame #0 {
                        w252 = TRUE ("Resize to Image Size? (Y)")
                        w251 = 0 ("Window Number (0...15)")
                        n94 = call "IMAQ WindNonTearing"("Window Number"=w251, "NonTearing? (True)"=w252) -> ()  [unwired: 8 in, 2 out]
                        n95 = call "IMAQ WindDraw"("Resize to Image Size? (Y)"=w252, "Window Number (0...15)"=w251, "Image"=w253) -> ()  [unwired: 7 in, 2 out]
                      }
                      frame #1 {
                        n96 = call "IMAQ WindSize"("Scrollbars? (N)"=FALSE, "Width & Height"="Initial Window Size", "Window Number"=w255) -> ()  [unwired: 3 in, 3 out]
                        n97 = call "IMAQ WindMove"("Window Number (0...15)"=w255, "Coordinates (screen)"="Initial Window Position") -> ()  [unwired: 3 in, 2 out]
                      }
                    }
                  }
                }
              }
              frame Enabled {
              }
            }
            n98 = To Unsigned Byte Integer(number=w200) -> (unsigned 8bit integer=w199:u8[][])
            n99 = call "IMAQ ArrayToImage"("Image Pixels (U8)"=w199, "Image"=w196) -> ("Image Out"=w194:T1)  [unwired: 4 in, 5 out]
            n100 = case shown="False" "Save Video" {
              tunnel: w201 -> [_ w259]
              tunnel: w194 -> [_ w258]
              frame False {
              }
              frame True {
                n101 = call "IMAQ AVI Write Frame"("Image"=w258, "Avi Refnum"=w259) -> ()  [unwired: 2 in, 8 out]
              }
            }
            n102 = case shown="False" "Save Image" {
              tunnel: w199 -> [_ w274]
              tunnel: w198 -> [_ w273]
              frame False {
              }
              frame True {
                n103 = call <vilib>:"Flatten Pixmap.vi"("colors"=w273, "8-bit pixmap"=w274) -> ("image data"=w280:T15)  [unwired: 4 in, 5 out]
                n104 = call "Create new save file.vi"("Insert"="video_frame_" ("string"), "Ext"=".bmp" ("string"), "Index In"="Image Index") -> ("Path Out"=w276:path, "Index Out"=w281:dbl)
                n105 = Increment(x=w281) -> (x+1=w275:dbl)
                n106 = local write "Image Index"(w275) -> ()
                n107 = call <vilib>:"Write BMP File.vi"("image data"=w280, "path to BMP file"=w276) -> ()  [unwired: 1 in, 9 out]
              }
            }
            n108 = case shown="False" "Target" {
              tunnel: w194 -> [w220 w224]
              tunnel: [w220 w222] -> w193
              frame False {
              }
              frame True {
                n109 = local read "Target coordinates"() -> (w221:cluster{"X1":dbl, "Y1":dbl, "X2":dbl, "Y2":dbl})
                n110 = call "IMAQ Overlay Oval"("Color"=u32 16711680, "Bounding Rectangle"=w221, "Image"=w224) -> ("Image Out"=w222:T1)  [unwired: 7 in, 1 out]
              }
            }
            "Primary Video Display" <- w193
          }
        }
        n111 = node-c288(w155) -> ()  [unwired: 1 out]
      }
      n112 = node-c288(w139) -> ()  [unwired: 1 out]
      n113 = call "DMR_CloseDevice2.vi"("driver handle IN"=w144) -> ()  [unwired: 3 in, 2 out]
    }
    frame #4 {
      n114 = call "DMR_Close.vi"() -> ()  [unwired: 1 out]
    }
  }
  n115 = while {
    tunnel: [w311] -> w73
    tunnel: [w502] -> w74
    tunnel: [w309] -> w72
    tunnel: [w614] -> w69
    tunnel: w27 -> [w296]
    tunnel: w26 -> [w610]
    tunnel: w25 -> [w615]
    stop <- w614 stop-if-true
    w351 = "NI_ChannelName" ("name")
    w427 = -1
    # "Scan # counter"
    # "DAQ loop iteration\ncounter (for timing)"
    # "Step counter"
    # "Force feedback"
    # "Raster scan"
    # "Rewire everything"
    # "Invert these because changed\nfrom PSD to QPD"
    # "Trap Y"
    # "Trap X"
    # "Convert to\npN"
    # "Convert to\nnm"
    # "Subtract\noffset"
    # "Normalize by\nsum"
    # "B sum"
    # "BX"
    # "BY"
    # "AX"
    # "AY"
    # "A sum"
    # "Close files when done saving"
    n116 = disable-structure shown="Disabled" {
      frame Disabled {
        n117 = property class="DAQmx Read"() -> ("AvailSampPerChan"=→"AvailSampPerChan 2":u32)  [unwired: 2 in, 2 out]
      }
      frame Enabled {
      }
    }
    n118 = local read "Averaging Number"() -> (w319:i32)
    n119 = local read "Averaging Number"() -> (w322:i32)
    "# Samples/channel" <- w322
    n120 = local read "Sampling Rate"() -> (w613:dbl)
    n121 = call-poly <vilib>:"DAQmx Read.vi"("task/channels in"=w296, "number of samples per channel"=w319, "timeout"=10.0) -> ("task out"=w295:refnum<k21>, "data"=w320:dbl[][], "error out"=w430:errorcluster)  [unwired: 10 in]
    n122 = Unbundle By Name(w430) -> ("status"=w550:bool)
    n123 = Divide(x=w613, y="Cal Averaging") -> (x/y=→"Cal Final Sampling Rate":dbl)
    n124 = Divide(x=w613, y=w322) -> (x/y=→"Final Sampling Rate" →"# Samples/channel/s":dbl)
    n125 = disable-structure shown="Disabled" {
      frame Disabled {
        n126 = local read "Buffer size\n(Samples/channel)"() -> (w617:u32)
        n127 = property class="DAQmx Read"() -> ("AvailSampPerChan"=w618:u32)  [unwired: 2 in, 2 out]
        "AvailSampPerChan" <- w618
        n128 = Divide(x=w618, y=w617) -> (x/y=→"Buffer status":dbl)
      }
      frame Enabled {
      }
    }
    n129 = case shown="True" w550 {
      frame False {
      }
      frame True {
        n130 = call <vilib>:"Beep.vi"() -> ()  [unwired: 12 in]
        "Buffer Overflow" <- TRUE
      }
    }
    n131 = local read "Cal values"() -> (w542:T2)
    n132 = Index Array(array=w320, index (row)=4) -> (element=w419:dbl[])  [unwired: 1 in]
    n133 = Index Array(array=w320, index (row)=0) -> (element=w429:dbl[])  [unwired: 1 in]
    n134 = Index Array(array=w320, index (row)=2) -> (element=w424:dbl[])  [unwired: 1 in]
    n135 = Index Array(array=w320, index (row)=1) -> (element=w428:dbl[])  [unwired: 1 in]
    n136 = Index Array(array=w320, index (row)=3) -> (element=w422:dbl[])  [unwired: 1 in]
    n137 = Index Array(array=w320, index (row)=6) -> (element=w421:dbl[])  [unwired: 1 in]
    n138 = Index Array(array=w320, index (row)=7) -> (element=w420:dbl[])  [unwired: 1 in]
    n139 = Index Array(array=w320, index (row)=5) -> (element=w418:dbl[])  [unwired: 1 in]
    n140 = Unbundle(w542) -> ("AX alpha"=w530:dbl, "BX alpha"=w526:dbl, "AX kappa"=w522:dbl, "BX kappa"=w518:dbl, "AX offset"=w536:dbl, "BX offset"=w534:dbl, "AY alpha"=w533:dbl, "BY alpha"=w528:dbl, "AY kappa"=w524:dbl, "BY kappa"=w520:dbl, "AY offset"=w540:dbl, "BY offset"=w538:dbl)
    n141 = Multiply(x=w428, y=w427) -> (x*y=w423:dbl[])
    n142 = Multiply(x=w429, y=w427) -> (x*y=w425:dbl[])
    n143 = local write "AX alpha"(w530) -> ()
    n144 = local write "BY offset"(w538) -> ()
    n145 = Build Array(w425, w424, w423, w422, w421, w420, w419, w418) -> (w348:dbl[][])
    n146 = local write "BX alpha"(w526) -> ()
    n147 = case shown="True" "Reset data stream" {
      selector: "Reset data stream" -> [_ w765]
      tunnel: w295 -> [w757 w763]
      tunnel: [w757 w761] -> w502
      tunnel: w430 -> [w756 w760]
      tunnel: [w756 w758] -> _
      frame False {
      }
      frame True {
        n148 = Not(x=w765) -> (.not. x?=w764:bool)
        n149 = call <vilib>:"DAQmx Stop Task.vi"("task/channels in"=w763, "error in"=w760) -> ("task out"=w762:refnum<k21>, "error out"=w759:errorcluster)  [unwired: 12 in]
        n150 = local write "Reset data stream"(w764) -> ()
        n151 = local write "Buffer Overflow"(w764) -> ()
        n152 = call <vilib>:"DAQmx Start Task.vi"("task/channels in"=w762, "error in"=w759) -> ("task out"=w761:refnum<k21>, "error out"=w758:errorcluster)  [unwired: 12 in]
      }
    }
    n153 = call-poly <vilib>:"Mean.vi"("X"=w418) -> ("mean"=w556:dbl)  [unwired: 1 out]
    n154 = local write "AY offset"(w540) -> ()
    n155 = call-poly <vilib>:"Mean.vi"("X"=w419) -> ("mean"=w557:dbl)  [unwired: 1 out]
    n156 = call-poly <vilib>:"Mean.vi"("X"=w424) -> ("mean"=w563:dbl)  [unwired: 1 out]
    n157 = call-poly <vilib>:"Mean.vi"("X"=w422) -> ("mean"=w561:dbl)  [unwired: 1 out]
    n158 = call-poly <vilib>:"Mean.vi"("X"=w421) -> ("mean"=w560:dbl)  [unwired: 1 out]
    n159 = call-poly <vilib>:"Mean.vi"("X"=w420) -> ("mean"=w559:dbl)  [unwired: 1 out]
    n160 = local read "Averaging Number"() -> (w318:i32)
    n161 = local write "BY kappa"(w520) -> ()
    n162 = local write "AX kappa"(w522) -> ()
    n163 = call-poly <vilib>:"Mean.vi"("X"=w423) -> ("mean"=w562:dbl)  [unwired: 1 out]
    n164 = local write "AY kappa"(w524) -> ()
    n165 = call-poly <vilib>:"Mean.vi"("X"=w425) -> ("mean"=w564:dbl)  [unwired: 1 out]
    n166 = local read "DAQ rate\n(Samples/s)"() -> (w326:dbl)
    n167 = Build Array(w557, w556) -> (w555:dbl[])
    n168 = local write "BX kappa"(w518) -> ()
    n169 = local write "BY alpha"(w528) -> ()
    n170 = local write "AX offset"(w536) -> ()
    n171 = local write "BX offset"(w534) -> ()
    n172 = local write "AY alpha"(w533) -> ()
    n173 = Build Array(w564, w563, w562, w561, w560, w559) -> (w553:dbl[])
    n174 = local read "Total raster time (s)"() -> (w292:dbl)
    n175 = Divide(x=w318, y=w326) -> (x/y=w288:dbl)
    "Data update period (s/set)" <- w288
    n176 = Reciprocal(x=w326) -> (1/x=w327:dbl)
    "Data period (s)" <- w327
    n177 = Divide(x=w292, y=w288) -> (x/y=w291:dbl)
    n178 = Divide(x="Cal time (s)", y=w288) -> (x/y=w287:dbl)
    n179 = Divide(x=w564, y=w560) -> (x/y=w594:dbl)
    n180 = Divide(x=w563, y=w560) -> (x/y=w595:dbl)
    n181 = Round Toward -Infinity(1:w291) -> (0:w290:dbl)
    n182 = Divide(x=w562, y=w559) -> (x/y=w602:dbl)
    n183 = Divide(x=w561, y=w559) -> (x/y=w603:dbl)
    n184 = Round Toward -Infinity(1:w287) -> (0:→"Cal sets to save":dbl)
    n185 = local write "N sets to be saved"(w290) -> ()
    n186 = Subtract(x=w594, y="AY offset") -> (x-y=w576:dbl)
    n187 = Subtract(x=w595, y="AX offset") -> (x-y=w577:dbl)
    n188 = Subtract(x=w602, y="BY offset") -> (x-y=w575:dbl)
    n189 = Subtract(x=w603, y="BX offset") -> (x-y=w578:dbl)
    n190 = Subtract(x=w602, y=w594) -> (x-y=w592:dbl)
    n191 = Subtract(x=w603, y=w595) -> (x-y=w593:dbl)
    n192 = feedback #4(0.0) -> (w501:dbl)
    n193 = Multiply(x="Downsamp\nfact", y=w327) -> (x*y=w328:dbl)
    n194 = Multiply(x=w576, y="AY alpha") -> (x*y=w510:dbl)
    n195 = Multiply(x=w577, y="AX alpha") -> (x*y=w508:dbl)
    n196 = Multiply(x=w578, y="BX alpha") -> (x*y=w509:dbl)
    n197 = Multiply(x=w575, y="BY alpha") -> (x*y=w511:dbl)
    n198 = Add(x=w288, y=w501) -> (x+y=w499:dbl)
    n199 = feedback-in #4(w499) -> ()
    n200 = Square(x=w510) -> (x^2=w586:dbl)
    n201 = Square(x=w508) -> (x^2=w587:dbl)
    n202 = Square(x=w511) -> (x^2=w588:dbl)
    n203 = Square(x=w509) -> (x^2=w589:dbl)
    n204 = Bundle(w592, w593) -> (w321:cluster{dbl, dbl})  [unwired: 1 in]
    n205 = case shown="True" "Set reading to\nsetpoint" {
      tunnel: w321 -> [_ w754]
      frame False {
      }
      frame True {
        n206 = local write "Set reading to\nsetpoint"(FALSE ("Set reading to\nsetpoint")) -> ()
        n207 = local read "Trap position (V)"() -> (w753:cluster{"X":dbl, "Y":dbl})
        n208 = property on="Setpoint voltage" class="Clust (strict)"("Val(Sgnl)"=w754) -> ()  [unwired: 2 in, 2 out]
        n209 = Unbundle(w753) -> ("X"=w752:dbl, "Y"=w751:dbl)
        n210 = Bundle("Y"=w751, "X"=w752) -> (w750:cluster{"Y":dbl, "X":dbl})  [unwired: 1 in]
        n211 = property on="Offset" class="Clust (strict)"("Val(Sgnl)"=w750) -> ()  [unwired: 2 in, 2 out]
      }
    }
    n212 = Reciprocal(x=w328) -> (1/x=→"Chart Freq (Hz)":dbl)
    n213 = To Time Stamp(1:w499) -> (0:w498:timestamp)
    n214 = Add(x=w586, y=w587) -> (x+y=w590:dbl)
    n215 = Add(x=w588, y=w589) -> (x+y=w601:dbl)
    n216 = Multiply(x=w508, y="AX kappa") -> (x*y=w504:dbl)
    n217 = Bundle("A y", "A x", "B y", "B x", "A sum", "B sum", "Trap x", "Trap y") -> (w489:T18)  [unwired: 1 in]
    n218 = Multiply(x=w509, y="BX kappa") -> (x*y=w505:dbl)
    n219 = Square Root(x=w590) -> (sqrt(x)=w606:dbl)
    n220 = Square Root(x=w601) -> (sqrt(x)=w605:dbl)
    n221 = Multiply(x=w510, y="AY kappa") -> (x*y=w506:dbl)
    n222 = Multiply(x=w511, y="BY kappa") -> (x*y=w507:dbl)
    n223 = Subtract(x=w556, y="Fixed Y") -> (x-y=w591:dbl)
    n224 = Subtract(x=w557, y="Fixed X") -> (x-y=w596:dbl)
    n225 = Cluster To Array(cluster=w489) -> (array=w488:string[])
    n226 = for {
      tunnel: w348 -> [w742] mode=indexing
      tunnel: w328 -> [w741]
      tunnel: "Downsamp\nfact" -> [w747]
      tunnel: [w745] -> w404 mode=indexing
      tunnel: w498 -> [w749]
      tunnel: w488 -> [w744] mode=indexing
      tunnel: "NI_ChannelName" ("name") -> [w743]
      n227 = call "Downsample 1D array.vi"("Ave N"=w747, "Arrray In"=w742) -> ("Array Out"=w748:dbl[])  [unwired: 9 in]
      n228 = Bundle By Name("Y"=w748, "dt"=w741, "t0"=w749) -> (w746:waveform(dbl))  [unwired: 1 in]
      n229 = Set Waveform Attribute(5:w744, 6:w743, 7:w746) -> (3:w745:waveform(dbl))  [unwired: 1 in, 2 out]
    }
    "All signals" <- w404
    n230 = Square(x=w506) -> (x^2=w579:dbl)
    n231 = Square(x=w504) -> (x^2=w580:dbl)
    n232 = Square(x=w507) -> (x^2=w581:dbl)
    n233 = Square(x=w505) -> (x^2=w582:dbl)
    n234 = Add(x=w579, y=w580) -> (x+y=w583:dbl)
    n235 = Add(x=w581, y=w582) -> (x+y=w584:dbl)
    n236 = Multiply(x=w591, y="Conv Y (nm/V)") -> (x*y=w513:dbl)
    n237 = Multiply(x=w596, y="Conv X (nm/V)") -> (x*y=w514:dbl)
    n238 = feedback #5() -> (w551:cluster{"B_Y":dbl, "B_X":dbl})  [unwired: 1 in]
    n239 = case shown="True" "Force Feedback" {
      tunnel: [w1039 w1055] -> w312
      tunnel: [w1038 w1054] -> w310
      tunnel: w321 -> [_ w1053]
      tunnel: [cluster{"B_Y":dbl, "B_X":dbl} {"B_Y"=0.0, "B_X"=0.0} ("Sum error past") w1045] -> w552
      tunnel: w551 -> [_ w1052]
      tunnel: w610 -> [w1039 w1048]
      tunnel: w615 -> [w1038 w1047]
      frame False {
        # "Force feedback"
      }
      frame True {
        n240 = call "ForceFeedback2.vi"("PSD/Mirror Voltages"=w1053, "Sum error"=w1052, "task/channels in"=w1048, "error in"=w1047, "Desired voltage"="Setpoint voltage", "Feedback const"="Feedback const", "offset"="Offset") -> ("task out"=w1055:refnum<k21>, "Sum error past"=w1045:cluster{"B_Y":dbl, "B_X":dbl}, "Output Voltage"=→"Feedback Output Voltage 2":cluster{dbl, dbl}, "error out"=w1054:errorcluster)  [unwired: 8 in, 1 out]
        n241 = local read "Pulling direction"() -> (w1044:bool)
        n242 = Unbundle(w1045) -> ("B_Y"=w1042:dbl, "B_X"=w1041:dbl)
        n243 = Select(t=w1042, s=w1044, f=w1041) -> (s? t:f=→"Sum error":dbl)
      }
    }
    n244 = feedback-in #5(w552) -> ()
    n245 = Square Root(x=w583) -> (sqrt(x)=w512:dbl)
    n246 = Square Root(x=w584) -> (sqrt(x)=w607:dbl)
    n247 = Add(x=w512, y=w607) -> (x+y=w585:dbl)
    n248 = Build Array(w594, w595, w602, w603, w560, w559, w512, w607, w606, w605, w514, w513) -> ()  [unwired: 1 out]
    n249 = Divide(x=w585, y=2.0) -> (x/y=w549:dbl)
    n250 = Index Array(array=w404, index=6) -> (element=w353:waveform(dbl))
    n251 = Index Array(array=w404, index=7) -> (element=w355:waveform(dbl))
    n252 = local read "Fixed X"() -> (w408:dbl)
    n253 = local read "Fixed Y"() -> (w410:dbl)
    n254 = Unbundle By Name(w353) -> ("Y"=w412:dbl[])
    n255 = Unbundle By Name(w355) -> ("Y"=w411:dbl[])
    n256 = Index Array(array=w404, index=0) -> (element=w361:waveform(dbl))
    n257 = Index Array(array=w404, index=1) -> (element=w485:waveform(dbl))
    n258 = Index Array(array=w404, index=4) -> (element=w479:waveform(dbl))
    n259 = Subtract(x=w412, y=w408) -> (x-y=w409:dbl[])
    n260 = Subtract(x=w411, y=w410) -> (x-y=w406:dbl[])
    n261 = Unbundle By Name(w361) -> ("Y"=w477:dbl[])
    n262 = Unbundle By Name(w485) -> ("Y"=w476:dbl[])
    n263 = Unbundle By Name(w479) -> ("Y"=w475:dbl[])
    n264 = Index Array(array=w404, index=5) -> (element=w478:waveform(dbl))
    n265 = local read "Conv X (nm/V)"() -> (w407:dbl)
    n266 = local read "Conv Y (nm/V)"() -> (w405:dbl)
    n267 = Index Array(array=w404, index=2) -> (element=w358:waveform(dbl))
    n268 = Index Array(array=w404, index=3) -> (element=w482:waveform(dbl))
    n269 = Set Waveform Attribute(5:"T2 X", 6:w351, 7:w353) -> (3:w352:waveform(dbl))  [unwired: 1 in, 2 out]
    n270 = Set Waveform Attribute(5:"T2 Y", 6:w351, 7:w355) -> (3:w354:waveform(dbl))  [unwired: 1 in, 2 out]
    n271 = Unbundle By Name(w478) -> ("Y"=w472:dbl[])
    n272 = Unbundle By Name(w358) -> ("Y"=w474:dbl[])
    n273 = Unbundle By Name(w482) -> ("Y"=w473:dbl[])
    n274 = Divide(x=w477, y=w475) -> (x/y=w376:dbl[])
    n275 = Divide(x=w476, y=w475) -> (x/y=w374:dbl[])
    n276 = local read "AY offset"() -> (w463:dbl)
    n277 = local read "AX offset"() -> (w461:dbl)
    n278 = Multiply(x=w409, y=w407) -> (x*y=w345:dbl[])
    n279 = Multiply(x=w406, y=w405) -> (x*y=w347:dbl[])
    n280 = Divide(x=w473, y=w472) -> (x/y=w375:dbl[])
    n281 = Subtract(x=w374, y=w461) -> (x-y=w464:dbl[])
    n282 = local read "BY offset"() -> (w468:dbl)
    n283 = local read "BX offset"() -> (w471:dbl)
    n284 = Subtract(x=w376, y=w463) -> (x-y=w465:dbl[])
    n285 = Divide(x=w474, y=w472) -> (x/y=w377:dbl[])
    n286 = local read "AY alpha"() -> (w462:dbl)
    n287 = local read "AX alpha"() -> (w460:dbl)
    n288 = call-poly <vilib>:"Mean.vi"("X"=w347) -> ("mean"=w387:dbl)  [unwired: 1 out]
    "Mean Trp Pos Y 2 (nm)" <- w387
    n289 = Subtract(x=w377, y=w376) -> (x-y=w373:dbl[])
    n290 = Subtract(x=w375, y=w374) -> (x-y=w372:dbl[])
    n291 = Subtract(x=w345, y="Offset X (nm)") -> (x-y=w344:dbl[])
    n292 = Subtract(x=w347, y="Offset Y (nm)") -> (x-y=w346:dbl[])
    n293 = Subtract(x=w377, y=w468) -> (x-y=w470:dbl[])
    n294 = Subtract(x=w375, y=w471) -> (x-y=w469:dbl[])
    n295 = Subtract(x=w387, y=w347) -> (x-y=w386:dbl[])
    n296 = call-poly <vilib>:"Mean.vi"("X"=w345) -> ("mean"=w391:dbl)  [unwired: 1 out]
    "Mean Trap Pos X 2 (nm)" <- w391
    n297 = Build Array(w373, w372) -> (w370:dbl[][])
    n298 = Index Array(array=w370, index (row)=0) -> (element=w368:dbl[])  [unwired: 1 in]
    n299 = Index Array(array=w370, index (row)=1) -> (element=w367:dbl[])  [unwired: 1 in]
    n300 = call-poly <vilib>:"Mean.vi"("X"=w368) -> ("mean"=w366:dbl)  [unwired: 1 out]
    n301 = call-poly <vilib>:"Mean.vi"("X"=w367) -> ("mean"=w365:dbl)  [unwired: 1 out]
    n302 = Bundle("mean"=w366, "mean"=w365) -> ()  [unwired: 1 in, 1 out]
    n303 = local read "BY alpha"() -> (w467:dbl)
    n304 = local read "BX alpha"() -> (w466:dbl)
    n305 = Multiply(x=w465, y=w462) -> (x*y=w453:dbl[])
    n306 = Multiply(x=w464, y=w460) -> (x*y=w452:dbl[])
    n307 = Square(x=w386) -> (x^2=w385:dbl[])
    n308 = Subtract(x=w391, y=w345) -> (x-y=w390:dbl[])
    n309 = Bundle By Name(cluster=w354, "Y"=w346) -> (w402:waveform(dbl))
    n310 = Bundle By Name(cluster=w352, "Y"=w344) -> (w403:waveform(dbl))
    n311 = local read "Raster scanning..."() -> (w294:bool)
    n312 = local read "Saving"() -> (w515:bool)
    n313 = local read "Tether"() -> (w516:bool)
    n314 = Square(x=w390) -> (x^2=w389:dbl[])
    n315 = call-poly <vilib>:"Mean.vi"("X"=w385) -> ("mean"=w384:dbl)  [unwired: 1 out]
    n316 = Square(x=w453) -> (x^2=w459:dbl[])
    n317 = Multiply(x=w470, y=w467) -> (x*y=w451:dbl[])
    n318 = Square(x=w452) -> (x^2=w458:dbl[])
    n319 = Multiply(x=w469, y=w466) -> (x*y=w450:dbl[])
    n320 = Less?(x=w549, y="Tether break\nforce (pN)") -> (x < y?=w547:bool)
    n321 = call-poly <vilib>:"Mean.vi"("X"=w389) -> ("mean"=w388:dbl)  [unwired: 1 out]
    n322 = Build Array(w403, w402) -> (w313:waveform(dbl)[])
    "Trap sep" <- w313
    n323 = Square Root(x=w384) -> (sqrt(x)=w383:dbl)
    n324 = Square(x=w451) -> (x^2=w457:dbl[])
    n325 = Square(x=w450) -> (x^2=w456:dbl[])
    n326 = Add(x=w459, y=w458) -> (x+y=w455:dbl[])
    n327 = Square Root(x=w388) -> (sqrt(x)=w381:dbl)
    n328 = Compound Arithmetic op=AND(w515, w516, w547) -> (w546:bool)
    n329 = Multiply(x=w383, y=10) -> (x*y=→"T2 Y RMS (A)":dbl)
    n330 = Square Root(x=w455) -> (sqrt(x)=w340:dbl[])
    n331 = Add(x=w457, y=w456) -> (x+y=w454:dbl[])
    n332 = Set Waveform Attribute(5:"T2", 6:"NI_ChannelName" ("name"), 7:w361) -> (3:w360:waveform(dbl))  [unwired: 1 in, 2 out]
    n333 = Set Waveform Attribute(5:"T1", 6:"NI_ChannelName" ("name"), 7:w358) -> (3:w357:waveform(dbl))  [unwired: 1 in, 2 out]
    n334 = case shown="True" w546 {
      selector: w546 -> [_ w772]
      tunnel: w294 -> [w766 w767]
      tunnel: [w766 w767] -> w293
      frame False {
      }
      frame True {
        n335 = call <vilib>:"Beep.vi"() -> ()  [unwired: 12 in]
        n336 = Not(x=w772) -> (.not. x?=w770:bool)
        n337 = And(x=w767, y="Fish After TA?") -> (x .and. y?=w769:bool)
        n338 = local write "Tether"(w770) -> ()
        n339 = local write "Force Feedback"(w770) -> ()
        n340 = case shown="True" w769 {
          selector: w769 -> [_ w773]
          frame False {
          }
          frame True {
            n341 = property on="Fish" class="Bool (strict)"("Val(Sgnl)"=w773) -> ()  [unwired: 2 in, 2 out]
          }
        }
        n342 = property on="Stop saving" class="Bool (strict)"("Val(Sgnl)"="TA Cancel Save?") -> ()  [unwired: 2 in, 2 out]
      }
    }
    n343 = Square Root(x=w454) -> (sqrt(x)=w339:dbl[])
    n344 = Multiply(x=w381, y=10) -> (x*y=→"T2 X RMS (A)":dbl)
    n345 = Bundle By Name(cluster=w360, "Y"=w340) -> (w364:waveform(dbl))
    n346 = Bundle By Name(cluster=w357, "Y"=w339) -> (w432:waveform(dbl))
    n347 = Add(x=w340, y=w339) -> (x+y=w338:dbl[])
    n348 = case shown="True" "Remove offsets" {
      selector: "Remove offsets" -> [_ w739]
      frame False {
      }
      frame True {
        n349 = local read "Mean Trp Pos Y 2 (nm)"() -> (w737:dbl)
        n350 = Not(x=w739) -> (.not. x?=w740:bool)
        n351 = local read "Mean Trap Pos X 2 (nm)"() -> (w738:dbl)
        n352 = local write "Remove offsets"(w740) -> ()
        n353 = local write "Offset Y (nm)"(w737) -> ()
        n354 = local write "Offset X (nm)"(w738) -> ()
      }
    }
    n355 = Build Array(w364, w432) -> (→"Bead sep":waveform(dbl)[])
    n356 = local read "AY kappa"() -> (w449:dbl)
    n357 = local read "AX kappa"() -> (w448:dbl)
    n358 = Divide(x=w338, y=2) -> (x/y=w336:dbl[])
    n359 = local read "BX kappa"() -> (w446:dbl)
    n360 = local read "BY kappa"() -> (w447:dbl)
    n361 = call-poly <vilib>:"Mean.vi"("X"=w336) -> ("mean"=w335:dbl)  [unwired: 1 out]
    "Mean Bead Sep\n(nm)" <- w335
    n362 = local read "Calibrating"() -> (w608:bool)
    n363 = Multiply(x=w453, y=w449) -> (x*y=w442:dbl[])
    n364 = Multiply(x=w452, y=w448) -> (x*y=w443:dbl[])
    n365 = Square(x=w442) -> (x^2=w441:dbl[])
    n366 = Square(x=w443) -> (x^2=w440:dbl[])
    n367 = Subtract(x=w336, y=w335) -> (x-y=w334:dbl[])
    n368 = Multiply(x=w451, y=w447) -> (x*y=w444:dbl[])
    n369 = Multiply(x=w450, y=w446) -> (x*y=w445:dbl[])
    n370 = Or(x=w293, y="Raster scan") -> (x .or. y?=w308:bool)
    n371 = Add(x=w441, y=w440) -> (x+y=w437:dbl[])
    n372 = Square(x=w334) -> (x^2=w333:dbl[])
    n373 = Square Root(x=w437) -> (sqrt(x)=w401:dbl[])
    n374 = Square(x=w444) -> (x^2=w439:dbl[])
    n375 = Square(x=w445) -> (x^2=w438:dbl[])
    n376 = call-poly <vilib>:"Mean.vi"("X"=w333) -> ("mean"=w332:dbl)  [unwired: 1 out]
    n377 = Add(x=w439, y=w438) -> (x+y=w436:dbl[])
    n378 = Bundle By Name(cluster=w360, "Y"=w401) -> (w435:waveform(dbl))
    n379 = local read "Saving"() -> (w545:bool)
    n380 = Or(x=w608, y=w545) -> ()  [unwired: 1 out]
    n381 = Square Root(x=w332) -> (sqrt(x)=w331:dbl)
    n382 = Square Root(x=w436) -> (sqrt(x)=w400:dbl[])
    n383 = Multiply(x=10, y=w331) -> (x*y=→"Bead Sep Noise\n(A)":dbl)
    n384 = Bundle By Name(cluster=w357, "Y"=w400) -> (w434:waveform(dbl))
    n385 = Add(x=w401, y=w400) -> (x+y=w399:dbl[])
    n386 = Build Array(w435, w434) -> (→"Force (pN)":waveform(dbl)[])
    n387 = Divide(x=w399, y=2) -> (x/y=w396:dbl[])
    n388 = call-poly <vilib>:"Mean.vi"("X"=w396) -> ("mean"=w397:dbl)  [unwired: 1 out]
    "Mean force (pN)" <- w397
    n389 = Subtract(x=w397, y=w396) -> (x-y=w395:dbl[])
    n390 = Square(x=w395) -> (x^2=w394:dbl[])
    n391 = call-poly <vilib>:"Mean.vi"("X"=w394) -> ("mean"=w393:dbl)  [unwired: 1 out]
    n392 = Square Root(x=w393) -> (sqrt(x)=→"Force noise (pN)":dbl)
    n393 = flat-sequence {
      tunnel: w608 -> [w813]
      tunnel: w545 -> [_]
      tunnel: w608 -> [_]
      tunnel: w545 -> [_]
      tunnel: w348 -> [w800]
      tunnel: [w800] -> w566
      tunnel: w430 -> [w799]
      tunnel: [w799] -> w565
      tunnel: w553 -> [w798]
      tunnel: [w798] -> w558
      tunnel: w555 -> [w797]
      tunnel: [w797] -> w554
      tunnel: [w794] -> w544
      tunnel: [w791] -> w543
      tunnel: [w788] -> w417
      tunnel: [w787] -> w416
      tunnel: [w784] -> w415
      tunnel: w315 -> [w781]
      tunnel: ["Save Data"] -> w314
      tunnel: w566 -> [w961]
      tunnel: w565 -> [w960]
      tunnel: w558 -> [_]
      tunnel: w554 -> [_]
      tunnel: w544 -> [w959]
      tunnel: w543 -> [w958]
      tunnel: w417 -> [w957]
      tunnel: w416 -> [w956]
      tunnel: w415 -> [w955]
      tunnel: w314 -> [w953]
      tunnel: w313 -> [w952]
      frame #0 {
        w779 = 0.0
        # "1: old trap\n0: fleezers"
        # "Create files if saving data"
        n394 = local read "Save N sets"() -> (w783:bool)
        n395 = local read "Sampling Rate"() -> (w811:dbl)
        n396 = Or(x=w783, y="Save Data") -> (x .or. y?=w782:bool)
        n397 = Build Array(w782, "Save cal", w781) -> (w802:bool[])
        n398 = Compound Arithmetic op=OR("Save Data", "Save cal", w781) -> (w804:bool)
        n399 = Boolean Array To Number(Boolean array=w802) -> (number=w801:u32)
        n400 = local read "Trap position (V)"() -> (w808:cluster{"X":dbl, "Y":dbl})
        n401 = local read "Fixed X"() -> (w778:dbl)
        n402 = local read "Fixed Y"() -> (w777:dbl)
        n403 = Unbundle(w808) -> ("X"=w776:dbl, "Y"=w775:dbl)
        n404 = Build Array(w776, w775, w778, w777, w779, w779) -> (w807:dbl[])
        n405 = feedback #6(refnum<k0> refnum) -> (w792:refnum<file>)
        n406 = feedback #7() -> (w789:dbl)  [unwired: 1 in]
        n407 = feedback #8(FALSE) -> (w785:bool)
        n408 = feedback #9(0) -> (w805:i32)
        n409 = feedback #10(refnum<k0> refnum) -> (w795:refnum<file>)
        n410 = case shown="True" w804 {
          tunnel: w813 -> [_ _]
          tunnel: 9 -> [_ w856]
          tunnel: w811 -> [_ w855]
          tunnel: 6 -> [_ w854]
          tunnel: 5 -> [_ w853]
          tunnel: w807 -> [_ w852]
          tunnel: [w818 1] -> w788
          tunnel: w805 -> [w819 _]
          tunnel: w801 -> [_ w827]
          tunnel: [w817 w826] -> w794
          tunnel: w795 -> [w817 _]
          tunnel: [w816 w825] -> w791
          tunnel: w792 -> [w816 _]
          tunnel: 1.0 -> [_ w824]
          tunnel: [w815 w823] -> w787
          tunnel: w789 -> [w815 _]
          tunnel: [w814 w822] -> w784
          tunnel: w785 -> [w814 _]
          frame False {
            n411 = Increment(x=w819) -> (x+1=w818:i32)
          }
          frame True {
            w828 = FALSE ("Save Data")
            w834 = FALSE
            w835 = T17."big-endian, network order" ("byte order (0:big-endian, network order)")
            n412 = local write "Save cal"(w828) -> ()
            n413 = local write "Save Data"(w828) -> ()
            n414 = case shown="4" w827 {
              tunnel: w856 -> [w903 w921 w951]
              tunnel: w855 -> [w881 w920 w926]
              tunnel: w854 -> [w902 w918 w947]
              tunnel: w853 -> [w901 w917 w946]
              tunnel: w852 -> [w899 w914 w943]
              tunnel: [w898 w913 w932] -> w849
              tunnel: [w900 w910 w931] -> w822
              tunnel: ["Averaging Number" 200 w929] -> _
              tunnel: w824 -> [w886 w905 w928]
              tunnel: [w882 w904 w922] -> w823
              frame 1, Default {
                w900 = TRUE
                w887 = 0.0
                # "Time trace"
                n415 = local read "Averaging Number"() -> (w897:i32)
                n416 = Boolean To (0,1)(Boolean=w900) -> (0, 1=w892:i16)
                n417 = Increment(x=w892) -> (x+1=w891:i16)
                n418 = Divide(x=w881, y=w897) -> (x/y=w896:dbl)
                n419 = To Double Precision Float(number=w891) -> (double precision float=w890:dbl)
                n420 = Reciprocal(x=w896) -> (1/x=w895:dbl)
                n421 = Reciprocal(x=w881) -> (1/x=w880:dbl)
                n422 = Build Array(w903, w880, w895, w902, w901, 0 ("f")) -> (w894:dbl[])
                n423 = Build Array(w890, w886, w887, w887, w887) -> (w893:dbl[])
                n424 = Build Array (concatenate)(w894, w899, w893) -> (w898:dbl[])
                n425 = Select(t="N sets", s="Save N sets", f=2147483647) -> (s? t:f=w882:i32)
              }
              frame 2 {
                w910 = FALSE
                w908 = 0.0
                # "Calibration file"
                n426 = Reciprocal(x=w920) -> (1/x=w919:dbl)
                n427 = Boolean To (0,1)(Boolean=w910) -> (0, 1=w912:i16)
                n428 = To Double Precision Float(number=w912) -> (double precision float=w911:dbl)
                n429 = Build Array(w921, w919, w919, w918, w917, 1) -> (w915:dbl[])
                n430 = Build Array(w911, w905, w908, w908, w908) -> (w909:dbl[])
                n431 = Build Array (concatenate)(w915, w914, w909) -> (w913:dbl[])
                n432 = local read "Cal sets to save"() -> (w904:i32)
                "Calibrating" <- TRUE ("Calibrating")
              }
              frame 4 {
                w939 = 0.0
                w931 = TRUE
                # "Not using ncycles"
                # "FX curve"
                n433 = local read "Averaging Number"() -> (w950:i32)
                n434 = Boolean To (0,1)(Boolean=w931) -> (0, 1=w942:i16)
                n435 = Increment(x=w942) -> (x+1=w941:i16)
                n436 = local write "Raster scan"(FALSE ("Raster scan")) -> ()
                n437 = To Double Precision Float(number=w941) -> (double precision float=w940:dbl)
                n438 = Divide(x=w926, y=w950) -> (x/y=w949:dbl)
                n439 = Reciprocal(x=w949) -> (1/x=w948:dbl)
                n440 = Build Array(w940, w928, w939, w939, w939) -> (w938:dbl[])
                n441 = Reciprocal(x=w926) -> (1/x=w925:dbl)
                n442 = Build Array(w951, w925, w948, w947, w946, 2) -> (w944:dbl[])
                n443 = local read "Pulling direction"() -> (w936:bool)
                n444 = local read "Scan range (V)"() -> (w923:dbl)
                n445 = local read "N sets to be saved"() -> (w922:dbl)
                n446 = local read "Scan steps (mirror)"() -> (w924:u64)
                n447 = local read "# scans"() -> (w934:i32)
                n448 = Not(x=w936) -> (.not. x?=w935:bool)
                n449 = local read "Averaging Number"() -> (w929:i32)
                n450 = Boolean To (0,1)(Boolean=w935) -> (0, 1=w937:i16)
                n451 = Build Array(w937, w923, w924, 0, w934) -> (w933:dbl[])
                n452 = Build Array (concatenate)(w944, w943, w938, w933) -> (w932:dbl[])
              }
            }
            n453 = call "CreateSaveFile.vi"("Index In"="Save file index", "Ext"=".dat", "Insert"="", "Directory"="Path") -> ("Index Out"=w821:i32, "Path Out"=w833:path)  [unwired: 6 in]
            "Current file name" <- w833
            n454 = Open/Create/Replace File(file path (use dialog)=w833, operation (0:open)=T16."create", access (0:read/write)=enum16{"read/write", "read-only", "write-only"}."write-only") -> (refnum out=w842:refnum<file>, error out=w843:errorcluster)  [unwired: 3 in, 1 out]
            n455 = local write "Save file index"(w821) -> ()
            n456 = Array Size(array=w849) -> (size(s)=w851:i32)
            n457 = case shown="True" w822 {
              tunnel: w833 -> [_ w879]
              tunnel: [refnum<k0> refnum w858] -> w825
              frame False {
              }
              frame True {
                w865 = 0.0
                n458 = Path To String(path=w879) -> (string=w875:string)
                n459 = Build Array(w865, w865, w865, w865, w865, w865, w865, w865) -> (w862:dbl[])
                n460 = String Length(string=w875) -> (length=w878:i32)
                n461 = Array Size(array=w862) -> (size(s)=w864:i32)
                n462 = Subtract(x=w878, y=4) -> (x-y=w876:i32)
                n463 = To Double Precision Float(number=w864) -> (double precision float=w863:dbl)
                n464 = String Subset(string=w875, length (rest)=w876) -> (substring=w874:string)  [unwired: 1 in]
                n465 = Build Array (concatenate)(w863, w862) -> (w861:dbl[])
                n466 = Concatenate Strings(w874, "_pos.dat" ("string")) -> (w872:string)
                n467 = String To Path(string=w872) -> (path=w871:path)
                n468 = Open/Create/Replace File(file path (use dialog)=w871, operation (0:open)=T16."create", access (0:read/write)=enum16{"read/write", "read-only", "write-only"}."write-only") -> (refnum out=w867:refnum<file>, error out=w868:errorcluster)  [unwired: 3 in, 1 out]
                n469 = Deny Access(4:w868, 7:w867) -> (3:w866:refnum<file>)  [unwired: 1 in, 1 out]
                n470 = Write to Binary File(file (use dialog)=w866, data=w861, 5:FALSE ("prepend array or string size? (T)"), 9:T17."big-endian, network order" ("byte order (0:big-endian, network order)")) -> (refnum out=w858:refnum<file>)  [unwired: 2 in, 2 out]
              }
            }
            n471 = Deny Access(4:w843, 7:w842) -> (0:w832:errorcluster, 3:w841:refnum<file>)  [unwired: 1 in]
            n472 = String Length(string="Comment") -> (length=w848:i32)
            n473 = To Double Precision Float(number=w851) -> (double precision float=w850:dbl)
            n474 = To Double Precision Float(number=w848) -> (double precision float=w847:dbl)
            n475 = Build Array (concatenate)(w850, w849, w847) -> (w838:dbl[])
            n476 = Write to Binary File(file (use dialog)=w841, data=w838, error in=w832, 5:w834, 9:w835) -> (refnum out=w837:refnum<file>, error out=w831:errorcluster)  [unwired: 1 in, 1 out]
            n477 = Write to Binary File(file (use dialog)=w837, data="Comment", error in=w831, 5:w834, 9:w835) -> (refnum out=w826:refnum<file>)  [unwired: 1 in, 2 out]
            "Saving" <- TRUE
          }
        }
        n478 = feedback-in #6(w791) -> ()
        n479 = feedback-in #7(w787) -> ()
        n480 = feedback-in #8(w784) -> ()
        n481 = feedback-in #9(w788) -> ()
        n482 = feedback-in #10(w794) -> ()
      }
      frame #1 {
        n483 = local read "Saving"() -> (w954:bool)
        n484 = case shown="True" w954 {
          tunnel: w961 -> [_ w980]
          tunnel: w960 -> [_ w979]
          tunnel: w959 -> [_ w978]
          tunnel: w958 -> [_ w977]
          tunnel: w957 -> [_ w967]
          tunnel: w956 -> [_ w968]
          tunnel: w955 -> [_ w971]
          tunnel: w953 -> [_ w963]
          tunnel: w952 -> [_ w962]
          frame False {
            (unwired) FALSE ("Calibrating")
          }
          frame True {
            n485 = local read "Stop"() -> (w975:bool)
            n486 = Less Or Equal?(x=w967, y=w968) -> (x <= y?=w976:bool)
            n487 = Divide(x=w967, y=w968) -> (x/y=w966:dbl)
            n488 = Or(x=w975, y="Stop saving") -> (x .or. y?=w974:bool)
            n489 = Not(x=w974) -> (.not. x?=w973:bool)
            n490 = Multiply(x=100.0, y=w966) -> (x*y=w965:dbl)
            n491 = And(x=w976, y=w973) -> (x .and. y?=w972:bool)
            n492 = case shown="True" w972 {
              tunnel: w978 -> [w985 w994]
              tunnel: w979 -> [_ w993]
              tunnel: w980 -> [_ w992]
              tunnel: w977 -> [w984 w991]
              tunnel: w971 -> [w982 _]
              tunnel: [0.0 ("Progress") w990] -> w970
              tunnel: w965 -> [_ w990]
              tunnel: w963 -> [_ w987]
              tunnel: w962 -> [_ w988]
              frame False {
                w983 = FALSE
                n493 = Close File(refnum=w985) -> ()  [unwired: 1 in, 2 out]
                n494 = case shown="True" w982 {
                  tunnel: w984 -> [_ w986]
                  frame False {
                  }
                  frame True {
                    n495 = Close File(refnum=w986) -> ()  [unwired: 1 in, 2 out]
                  }
                }
                n496 = call <vilib>:"Beep.vi"() -> ()  [unwired: 12 in]
                n497 = local write "Saving"(w983) -> ()
                n498 = local write "Stop saving"(w983) -> ()
                n499 = local write "Calibrating"(w983) -> ()
              }
              frame True {
                n500 = local read "Calibrating"() -> (w989:bool)
                n501 = case shown="False" w989 {
                  tunnel: w994 -> [w1021 w1037]
                  tunnel: w993 -> [_ w1036]
                  tunnel: w992 -> [w1008 w1030]
                  tunnel: w991 -> [w1007 _]
                  tunnel: w988 -> [w999 _]
                  tunnel: w987 -> [_ _]
                  frame False {
                    n502 = local read "Averaging Number"() -> (w1015:i32)
                    n503 = Array Subset(array=w1008, index (row)=0 ("index"), length (row)=6 ("length")) -> (w1004:dbl[][])  [unwired: 2 in]
                    n504 = Array Subset(array=w1008, index (row)=6 ("index"), length (row)=2 ("length")) -> (w1003:dbl[][])  [unwired: 2 in]
                    n505 = Array Size(array=w1003) -> (size(s)=w1014:i32[])
                    n506 = Array Size(array=w1004) -> (size(s)=w1011:i32[])
                    n507 = Index Array(array=w999, index=0) -> (element=w996:waveform(dbl))
                    n508 = Index Array(array=w999, index=1) -> (element=w995:waveform(dbl))
                    n509 = for {
                      tunnel: w1004 -> [w1025] mode=indexing
                      tunnel: w1015 -> [w1027]
                      tunnel: [w1026] -> w1002 mode=indexing
                      n510 = call "Downsample 1D array.vi"("Ave N"=w1027, "Arrray In"=w1025) -> ("Array Out"=w1026:dbl[])  [unwired: 9 in]
                    }
                    n511 = Unbundle By Name(w996) -> ()  [unwired: 1 out]
                    n512 = Unbundle By Name(w995) -> ()  [unwired: 1 out]
                    n513 = Multiply Array Elements(1:w1011) -> (0:w1010:i32)
                    n514 = for {
                      tunnel: w1003 -> [w1024] mode=indexing
                      tunnel: w1015 -> [w1023]
                      tunnel: [w1022] -> w1006 mode=indexing
                      n515 = call "Downsample 1D array.vi"("Ave N"=w1023, "Arrray In"=w1024) -> ("Array Out"=w1022:dbl[])  [unwired: 9 in]
                    }
                    n516 = Multiply Array Elements(1:w1014) -> (0:w1013:i32)
                    n517 = Divide(x=w1010, y=w1015) -> (x/y=w1016:dbl)
                    n518 = Divide(x=w1013, y=w1015) -> (x/y=w1012:dbl)
                    n519 = Transpose 2D Array(2D array=w1002) -> (transposed array=w1001:dbl[][])
                    n520 = Transpose 2D Array(2D array=w1006) -> (transposed array=w1000:dbl[][])
                    n521 = Reshape Array(w1001, w1016) -> (w1005:dbl[])
                    n522 = Reshape Array(w1000, w1012) -> (w1009:dbl[])
                    n523 = call <vilib>:"Write File+ [SGL].vi"("1D array"=w1009, "refnum"=w1007) -> ()  [unwired: 7 in, 3 out]
                    n524 = call <vilib>:"Write File+ [SGL].vi"("1D array"=w1005, "refnum"=w1021) -> ()  [unwired: 7 in, 3 out]
                  }
                  frame True {
                    n525 = Array Subset(array=w1030, index (row)=0 ("index"), length (row)=6 ("length")) -> (w1028:dbl[][])  [unwired: 2 in]
                    n526 = Transpose 2D Array(2D array=w1028) -> (transposed array=w1034:dbl[][])
                    n527 = Array Size(array=w1028) -> (size(s)=w1029:i32[])
                    n528 = Multiply Array Elements(1:w1029) -> (0:w1035:i32)
                    n529 = Reshape Array(w1034, w1035) -> (w1033:dbl[])
                    n530 = call <vilib>:"Write File+ [SGL].vi"("1D array"=w1033, "error in (no error)"=w1036, "refnum"=w1037) -> ()  [unwired: 6 in, 3 out]
                  }
                }
              }
            }
            "Progress" <- w970
          }
        }
      }
    }
    n531 = local read "Flushing Sample"() -> (w317:bool)
    n532 = case shown="True" w317 {
      frame False {
      }
      frame True {
        n533 = local read "Flush Sample Start Time"() -> (w733:u32)
        n534 = local read "Sample flush time (s)"() -> (w726:dbl)
        n535 = Tick Count (ms)() -> (millisecond timer value=w734:u32)
        n536 = Subtract(x=w734, y=w733) -> (x-y=w724:u32)
        n537 = Multiply(x=u32 1000, y=w726) -> (x*y=w725:dbl)
        n538 = Divide(x=w724, y=w725) -> (x/y=w729:dbl)
        n539 = Greater?(x=w724, y=w725) -> (0:w732:bool)
        n540 = Not(x=w732) -> (.not. x?=w731:bool)
        n541 = Boolean To (0,1)(Boolean=w731) -> (0, 1=w730:i16)
        n542 = Compound Arithmetic op=MULTIPLY(w730, w729, 100.0 ("value")) -> (→"Sample Flush Meter":dbl)
        n543 = case shown="True" w732 {
          frame False {
          }
          frame True {
            w736 = FALSE ("Inject Sample")
            n544 = property on="Clear Volume" class="Bool (strict)"("Val(Sgnl)"=TRUE ("Value (Signaling)")) -> ()  [unwired: 2 in, 2 out]
            n545 = local write "Inject Sample"(w736) -> ()
            n546 = local write "Flushing Sample"(w736) -> ()
          }
        }
      }
    }
    n547 = feedback #11(0) -> (w301:i32)
    n548 = feedback #12(0) -> (w298:i32)
    n549 = feedback #13(0) -> (w303:i32)
    n550 = case shown="True" w308 {
      tunnel: w312 -> [w626 w683]
      tunnel: [w626 w667] -> w311
      tunnel: w310 -> [w625 w682]
      tunnel: [w625 w666] -> w309
      tunnel: "Raster scan" -> [w624 w660]
      tunnel: [w624 w659] -> w306
      tunnel: [0 w658] -> w304
      tunnel: w303 -> [_ w652]
      tunnel: w301 -> [_ w640]
      tunnel: [0 w643] -> w300
      tunnel: w298 -> [_ w649]
      tunnel: [0 w648] -> w297
      frame False {
      }
      frame True {
        # "Reset step counter"
        # "Current position"
        # "Initial values"
        n551 = local read "Conv Y (nm/V)"() -> (w635:dbl)
        n552 = local read "Conv X (nm/V)"() -> (w636:dbl)
        n553 = local read "Trap delta (nm)"() -> (w634:dbl)
        n554 = disable-structure shown="Disabled" {
          frame Disabled {
            n555 = local write "Raster scan"(FALSE ("Raster scan")) -> ()
            n556 = property on="Reset data stream" class="Bool (strict)"("Val(Sgnl)"=TRUE) -> ()  [unwired: 2 in, 2 out]
          }
          frame Enabled {
          }
        }
        n557 = local read "Data update period (s/set)"() -> (w657:dbl)
        n558 = local read "Time per step (ms)"() -> (w654:dbl)
        n559 = Select(t=w635, s="Pulling direction", f=w636) -> (s? t:f=w633:dbl)
        n560 = Divide(x=w634, y=w633) -> (x/y=w632:dbl)
        n561 = local read "Fixed X"() -> (w676:dbl)
        n562 = local read "Fixed Y"() -> (w677:dbl)
        n563 = local read "Fixed X"() -> (w638:dbl)
        n564 = local read "Fixed Y"() -> (w637:dbl)
        n565 = local read "Trap position (V)"() -> (w639:cluster{"X":dbl, "Y":dbl})
        n566 = Select(t=w637, s="Pulling direction", f=w638) -> (s? t:f=w631:dbl)
        n567 = local read "Scan steps (mirror)"() -> (w665:u64)
        n568 = Unbundle(w639) -> ("X"=w629:dbl, "Y"=w630:dbl)
        n569 = Multiply(x=w657, y=1000.0) -> (x*y=w655:dbl)
        n570 = local read "Stop raster"() -> (w672:bool)
        n571 = local read "Stop saving"() -> (w673:bool)
        n572 = Select(t=w676, s="Pulling direction", f=w677) -> (s? t:f=w684:dbl)
        n573 = Add(x=w632, y=w631) -> ()  [unwired: 1 out]
        n574 = Divide(x=w654, y=w655) -> (x/y=w653:dbl)
        n575 = Quotient & Remainder(x=w652, y=w653) -> (x-y*floor(x/y)=w651:dbl)  [unwired: 1 out]
        n576 = Not(x=w672) -> (.not. x?=w671:bool)
        n577 = Select(t=w630, s="Pulling direction", f=w629) -> (s? t:f=w627:dbl)
        n578 = Not(x=w673) -> (.not. x?=w670:bool)
        n579 = Multiply(x=u64 2, y=w665) -> (x*y=w661:u64)
        n580 = Equal To 0?(x=w651) -> (x = 0?=w650:bool)
        n581 = Less?(x=w640, y=w661) -> (x < y?=w662:bool)
        n582 = Compound Arithmetic op=AND(w662, w671, w670, w650) -> (w663:bool)
        n583 = Not(x=w662) -> (.not. x?=w646:bool)
        n584 = feedback #14() -> (w668:dbl)  [unwired: 1 in]
        n585 = case shown="True" w663 {
          tunnel: w684 -> [_ w719]
          tunnel: w627 -> [_ w701]
          tunnel: w683 -> [w696 w718]
          tunnel: w682 -> [w695 w717]
          tunnel: [w696 w716] -> w667
          tunnel: [w695 w715] -> w666
          tunnel: [w692 w704] -> w669
          tunnel: w640 -> [w693 w699]
          tunnel: w668 -> [w692 w698]
          tunnel: w660 -> [w694 w703]
          tunnel: [w694 w703] -> w659
          tunnel: [w693 w702] -> w644
          frame False {
          }
          frame True {
            # "Go forward or backward?"
            n586 = local read "Scan increment (V)"() -> (w697:dbl)
            n587 = local read "Scan steps (mirror)"() -> (w708:u64)
            n588 = Multiply(x=w697, y=w699) -> (x*y=w700:dbl)
            n589 = Less?(x=w699, y=w708) -> (x < y?=w707:bool)
            n590 = Add(x=w701, y=w700) -> (x+y=w710:dbl)
            n591 = Subtract(x=w698, y=w697) -> (x-y=w709:dbl)
            n592 = Select(t=w710, s=w707, f=w709) -> (s? t:f=w704:dbl)
            n593 = local read "Pulling direction"() -> (w706:bool)
            n594 = Build Array(w704, w719) -> (w713:dbl[])
            n595 = Build Array(w719, w704) -> (w712:dbl[])
            n596 = Select(t=w713, s=w706, f=w712) -> (s? t:f=w711:dbl[])
            n597 = call-poly <vilib>:"DAQmx Write.vi"("task/channels in"=w718, "auto start"=TRUE, "data"=w711, "error in"=w717) -> ("task out"=w716:refnum<k21>, "error out"=w715:errorcluster)  [unwired: 9 in, 1 out]
            n598 = Increment(x=w699) -> (x+1=w702:i32)
            "Raster scanning..." <- TRUE ("Raster scanning...")
          }
        }
        n599 = feedback-in #14(w669) -> ()
        n600 = case shown="True" w646 {
          tunnel: w649 -> [w689 w691]
          tunnel: [w689 w690] -> w648
          frame False {
          }
          frame True {
            n601 = Increment(x=w691) -> (x+1=w690:i32)
          }
        }
        n602 = local read "# scans"() -> (w647:i32)
        n603 = local read "Stop saving"() -> (w675:bool)
        n604 = Greater Or Equal?(x=w648, y=w647) -> (x >= y?=w641:bool)
        n605 = Not(x=w641) -> (.not. x?=w642:bool)
        n606 = And(x=w646, y=w642) -> (x .and. y?=w645:bool)
        n607 = Compound Arithmetic op=OR(w641, "Stop raster", w675) -> (w678:bool)
        n608 = case shown="True" w678 {
          frame False {
          }
          frame True {
            n609 = flat-sequence {
              frame #0 {
                n610 = Wait (ms)(milliseconds to wait=u32 300) -> ()  [unwired: 1 out]
              }
              frame #1 {
                n611 = property on="Trap delta (nm)" class="DigNum (strict)"("Val(Sgnl)"="Trap delta\nafter (nm)") -> ()  [unwired: 2 in, 2 out]
              }
            }
          }
        }
        n612 = And(x="Flow on\nafter raster?", y=w678) -> (x .and. y?=w679:bool)
        n613 = case shown="True" w679 {
          frame False {
          }
          frame True {
            n614 = property on="Inject Sample" class="Bool (strict)"("Val(Sgnl)"=TRUE ("Value (Signaling)")) -> ()  [unwired: 2 in, 2 out]
          }
        }
        n615 = case shown="True" w645 {
          tunnel: w644 -> [w687 _]
          tunnel: [w687 0] -> w643
          frame False {
          }
          frame True {
          }
        }
        n616 = Not(x=w678) -> (.not. x?=w681:bool)
        n617 = local write "Raster scanning..."(w681) -> ()
        n618 = Increment(x=w652) -> (x+1=w658:i32)
      }
    }
    n619 = And(x="Save scans", y=w306) -> (x .and. y?=w315:bool)
    n620 = feedback-in #11(w300) -> ()
    n621 = feedback-in #12(w297) -> ()
    n622 = feedback-in #13(w304) -> ()
    n623 = local read "Stop"() -> (w614:bool)
  }
  n624 = local write "Progress"(u8 0 ("Progress")) -> ()
  n625 = local write "Calibrating"(FALSE ("Calibrating")) -> ()
  n626 = call-poly "VISA Configure Serial Port"("VISA resource name"=refnum<visa-resource-name> "COM5") -> ("VISA resource name out"=w17:refnum<visa-resource-name>, "error out"=w16:errorcluster)  [unwired: 13 in]
  n627 = node-c288(i64 100 ("Period"), 2 ("Processor")) -> (w19:T11)  [unwired: 2 in]
  n628 = timed-loop {
    timing: w19 -> [_]
    timing-out: [_] -> w18
    tunnel: w17 -> [w1056]
    tunnel: w16 -> [w1058]
    tunnel: [w1056] -> w15
    stop <- w1057 stop-if-true
    n629 = node-c288() -> ()  [unwired: 1 in, 1 out]
    n630 = event shown="[5] \"Move to Position 2\", \"Move to Position 4\", \"Move to Position 3\", \"Move to Position 5\", \"Move to Position 1\": Value Change" {
      selector: _ -> [_ _ _ _ _ _ _ _ _ _ _ _ _ _]
      dyn-events: _ -> [_ _ _ _ _ _ _ _ _ _ _ _ _ _]
      timeout: _ -> [_ _ _ _ _ _ _ _ _ _ _ _ _ _]
      tunnel: w1056 -> [w1064 w1115 w1135 w1152 w1169 w1188 w1211 w1221 _ _ _ _ _ _]
      tunnel: w1058 -> [w1063 w1114 w1134 w1151 w1168 w1187 w1210 w1220 _ _ _ _ _ _]
      tunnel: [_ _ _ _ _ _ _ _ _ _ _ _ _ w1313] -> w1057
      event "Got DNA bead": Value Change {
        n631 = event-data() -> ()  [unwired: 1 in, 5 out]
        n632 = flat-sequence {
          tunnel: w1064 -> [w1069]
          tunnel: w1063 -> [w1067]
          tunnel: ["Cal @ Delta (nm)"] -> w1059
          tunnel: [w1083] -> w1062
          tunnel: w1059 -> [w1082]
          tunnel: w1062 -> [w1104]
          tunnel: [w1104] -> w1061
          tunnel: w1061 -> [w1106]
          tunnel: [w1106] -> w1060
          tunnel: w1060 -> [w1108]
          frame #0 {
            n633 = local read "Saved stage positions"() -> (w1070:dbl[][])
            n634 = disable-structure shown="Disabled" {
              frame Disabled {
                n635 = property on="Inject Pump 2" class="Bool (strict)"("Val(Sgnl)"=FALSE ("Inject Pump 2")) -> ()  [unwired: 2 in, 2 out]
              }
              frame Enabled {
              }
            }
            n636 = property on="Inject Sample" class="Bool (strict)"("Val(Sgnl)"=TRUE ("Value (Signaling)")) -> ()  [unwired: 2 in, 2 out]
            n637 = local write "Stage moving"(TRUE ("Stage moving")) -> ()
            n638 = property on="Trap delta (nm)" class="DigNum (strict)"("Val(Sgnl)"="Cal @ Delta (nm)") -> ()  [unwired: 2 in, 2 out]
            n639 = call "move to saved stage position.vi"("error in"=w1067, "Stage VISA resource name in"=w1069, "Position"="Cal stage position", "Saved Stage Positions"=w1070) -> ()  [unwired: 2 out]
          }
          frame #1 {
            n640 = local write "Stage moving"(FALSE ("Stage moving")) -> ()
            n641 = property on="Inject Sample" class="Bool (strict)"("Val(Sgnl)"=FALSE ("Value (Signaling)")) -> ()  [unwired: 2 in, 2 out]
            n642 = call <vilib>:"Beep.vi"() -> ()  [unwired: 12 in]
          }
          frame #2 {
            n643 = Wait (ms)(milliseconds to wait=u32 1000) -> ()  [unwired: 1 out]
          }
          frame #3 {
            n644 = property on="Save cal" class="Bool (strict)"("Val(Sgnl)"=TRUE ("Value (Signaling)")) -> ()  [unwired: 2 in, 2 out]
          }
          frame #4 {
            n645 = Wait (ms)(milliseconds to wait=u32 2000) -> ()  [unwired: 1 out]
          }
          frame #5 {
            n646 = while {
              stop <- w1079 stop-if-true
              n647 = local read "Saving"() -> (w1080:bool)
              n648 = Not(x=w1080) -> (.not. x?=w1079:bool)
              n649 = Wait (ms)(milliseconds to wait=u32 100) -> ()  [unwired: 1 out]
            }
          }
          frame #6 {
            n650 = Wait (ms)(milliseconds to wait=u32 2000) -> ()  [unwired: 1 out]
          }
          frame #7 {
            n651 = stacked-sequence {
              tunnel: [_ _ _ _ _ _ w1098 _] -> w1083
              tunnel: w1082 -> [_ _ _ _ _ _ _ w1103]
              frame #0 {
                n652 = property on="Trap delta (nm)" class="DigNum (strict)"("Val(Sgnl)"="Offset @ Delta (nm)") -> ()  [unwired: 2 in, 2 out]
                n653 = Replace Array Subset(array=i32[] [0], new element="Offset raster set", index=0) -> (w1087:i32[])
                n654 = property on="Scan Parameters" class="Arr (strict)"("Index Values"=w1087) -> ()  [unwired: 2 in, 2 out]
              }
              frame #1 {
                n655 = Wait (ms)(milliseconds to wait=u32 200) -> ()  [unwired: 1 out]
              }
              frame #2 {
                n656 = property on="Load param" class="Bool (strict)"("Val(Sgnl)"=TRUE ("Load param")) -> ()  [unwired: 2 in, 2 out]
              }
              frame #3 {
                n657 = Wait (ms)(milliseconds to wait=u32 200) -> ()  [unwired: 1 out]
              }
              frame #4 {
                # "Only continue if there is no buffer\noverflow error"
                n658 = local read "Buffer Overflow"() -> (w1093:bool)
                n659 = Not(x=w1093) -> (.not. x?=w1092:bool)
                n660 = case shown="True" w1092 {
                  frame False {
                  }
                  frame True {
                    n661 = property on="Raster scan" class="Bool (strict)"("Val(Sgnl)"=TRUE ("Value (Signaling)")) -> ()  [unwired: 2 in, 2 out]
                  }
                }
              }
              frame #5 {
                n662 = local read "Buffer Overflow"() -> (w1096:bool)
                n663 = Not(x=w1096) -> (.not. x?=w1095:bool)
                n664 = case shown="True" w1095 {
                  frame False {
                  }
                  frame True {
                    n665 = Wait (ms)(milliseconds to wait=u32 2000) -> ()  [unwired: 1 out]
                  }
                }
              }
              frame #6 {
                n666 = local read "Buffer Overflow"() -> (w1099:bool)
                n667 = Not(x=w1099) -> (.not. x?=w1098:bool)
                n668 = case shown="True" w1098 {
                  frame False {
                  }
                  frame True {
                    n669 = while {
                      stop <- w1101 stop-if-true
                      n670 = local read "Saving"() -> (w1102:bool)
                      n671 = Not(x=w1102) -> (.not. x?=w1101:bool)
                      n672 = Wait (ms)(milliseconds to wait=u32 100) -> ()  [unwired: 1 out]
                    }
                  }
                }
              }
              frame #7 {
                n673 = property on="Trap delta (nm)" class="DigNum (strict)"("Val(Sgnl)"=w1103) -> ()  [unwired: 2 in, 2 out]
              }
            }
          }
          frame #8 {
            n674 = case shown="True" w1104 {
              frame False {
              }
              frame True {
                n675 = property on="Read Cal" class="Bool (strict)"("Val(Sgnl)"=TRUE ("Value (Signaling)")) -> ()  [unwired: 2 in, 2 out]
              }
            }
          }
          frame #9 {
            n676 = case shown="True" w1106 {
              frame False {
              }
              frame True {
                n677 = Wait (ms)(milliseconds to wait=u32 1000) -> ()  [unwired: 1 out]
              }
            }
          }
          frame #10 {
            n678 = case shown="True" w1108 {
              frame False {
              }
              frame True {
                n679 = property on="Fish" class="Bool (strict)"("Val(Sgnl)"=TRUE ("Value (Signaling)")) -> ()  [unwired: 2 in, 2 out]
                n680 = case shown="True" "Flow on\nwhile fish?" {
                  frame False {
                  }
                  frame True {
                    n681 = property on="Inject Sample" class="Bool (strict)"("Val(Sgnl)"=TRUE ("Value (Signaling)")) -> ()  [unwired: 2 in, 2 out]
                  }
                }
              }
            }
          }
        }
      }
      event "Dump beads": Value Change {
        n682 = event-data() -> ()  [unwired: 1 in, 5 out]
        n683 = flat-sequence {
          tunnel: w1114 -> [w1118]
          tunnel: w1115 -> [w1119]
          tunnel: [w1119] -> w1113
          tunnel: [w1118] -> w1112
          tunnel: w1113 -> [w1122]
          tunnel: w1112 -> [w1121]
          frame #0 {
            w1116 = FALSE ("Fish")
            n684 = local read "Saving"() -> (w1117:bool)
            n685 = local write "Pause dwell"(w1116) -> ()
            n686 = local write "Force Feedback"(w1116) -> ()
            n687 = local write "Dump beads"(w1116) -> ()
            n688 = property on="Stop saving" class="Bool (strict)"("Val(Sgnl)"=w1117) -> ()  [unwired: 2 in, 2 out]
            n689 = local write "Fish"(w1116) -> ()
          }
          frame #1 {
            n690 = local read "Saved stage positions"() -> (w1124:dbl[][])
            n691 = case shown="True" "Flow on\ndump?" {
              frame False {
              }
              frame True {
                n692 = property on="Inject Sample" class="Bool (strict)"("Val(Sgnl)"=TRUE ("Value (Signaling)")) -> ()  [unwired: 2 in, 2 out]
              }
            }
            n693 = local write "Stage moving"(TRUE ("Stage moving")) -> ()
            n694 = call "move to saved stage position.vi"("error in"=w1121, "Stage VISA resource name in"=w1122, "Position"=5, "Saved Stage Positions"=w1124) -> ()  [unwired: 2 out]
          }
          frame #2 {
            n695 = local read "Shutter 1 (B)"() -> (w1129:bool)
            n696 = local read "Shutter 2 (A)"() -> (w1128:bool)
            n697 = call <vilib>:"Beep.vi"() -> ()  [unwired: 12 in]
            n698 = case shown="True" w1129 {
              frame False {
              }
              frame True {
                n699 = property on="Shutter 1 (B)" class="Bool (strict)"("Val(Sgnl)"=FALSE ("Value (Signaling)")) -> ()  [unwired: 2 in, 2 out]
              }
            }
            n700 = case shown="True" w1128 {
              frame False {
              }
              frame True {
                n701 = property on="Shutter 2 (A)" class="Bool (strict)"("Val(Sgnl)"=FALSE) -> ()  [unwired: 2 in, 2 out]
              }
            }
            n702 = local write "Stage moving"(FALSE ("Stage moving")) -> ()
            n703 = local write "Tether"(FALSE ("Tether")) -> ()
          }
          frame #3 {
            n704 = property on="Move Cap. 2 (ADig Top)" class="Bool (strict)"("Val(Sgnl)"=TRUE ("Value (Signaling)")) -> ()  [unwired: 2 in, 2 out]
          }
        }
      }
      event "Move Cap. 2 (ADig Top)": Value Change {
        n705 = event-data() -> ()  [unwired: 1 in, 5 out]
        n706 = flat-sequence {
          tunnel: w1135 -> [w1139]
          tunnel: w1134 -> [w1138]
          frame #0 {
            n707 = local read "Saved stage positions"() -> (w1137:dbl[][])
            n708 = case shown="True" "Flow on\ncap 2?" {
              frame False {
              }
              frame True {
                n709 = property on="Inject Sample" class="Bool (strict)"("Val(Sgnl)"=TRUE ("Value (Signaling)")) -> ()  [unwired: 2 in, 2 out]
              }
            }
            n710 = local write "Move Cap. 2 (ADig Top)"(FALSE ("Move Cap. 2 (ADig Top)")) -> ()
            n711 = local write "Stage moving"(TRUE ("Stage moving")) -> ()
            n712 = call "move to saved stage position.vi"("error in"=w1138, "Stage VISA resource name in"=w1139, "Position"=2, "Saved Stage Positions"=w1137) -> ()  [unwired: 2 out]
          }
          frame #1 {
            # "Make sure you don't reverse\nwhich is ON and OFF"
            n713 = local read "Cal @ Delta (nm)"() -> (w1146:dbl)
            n714 = local write "Stage moving"(FALSE ("Stage moving")) -> ()
            n715 = call <vilib>:"Beep.vi"() -> ()  [unwired: 12 in]
            n716 = property on="Trap delta (nm)" class="DigNum (strict)"("Val(Sgnl)"=w1146) -> ()  [unwired: 2 in, 2 out]
            n717 = disable-structure shown="Disabled" {
              frame Disabled {
                n718 = property on="Inject Pump 1" class="Bool (strict)"("Val(Sgnl)"=TRUE ("Inject Pump 2")) -> ()  [unwired: 2 in, 2 out]
              }
              frame Enabled {
              }
            }
            n719 = local read "Shutter 2 (A)"() -> (w1145:bool)
            n720 = case shown="False" w1145 {
              frame False {
                n721 = property on="Shutter 2 (A)" class="Bool (strict)"("Val(Sgnl)"=TRUE ("Value (Signaling)")) -> ()  [unwired: 2 in, 2 out]
              }
              frame True {
              }
            }
            n722 = property on="Inject Sample" class="Bool (strict)"("Val(Sgnl)"=FALSE ("Value (Signaling)")) -> ()  [unwired: 2 in, 2 out]
          }
        }
      }
      event "Got ADig bead": Value Change {
        n723 = event-data() -> ()  [unwired: 1 in, 5 out]
        n724 = flat-sequence {
          tunnel: w1152 -> [w1156]
          tunnel: w1151 -> [w1155]
          frame #0 {
            n725 = local read "Saved stage positions"() -> (w1158:dbl[][])
            n726 = property on="Inject Pump 1" class="Bool (strict)"("Val(Sgnl)"=FALSE ("Inject Pump 2")) -> ()  [unwired: 2 in, 2 out]
            n727 = case shown="True" "Flow on\ncap 1?" {
              frame False {
              }
              frame True {
                n728 = property on="Inject Sample" class="Bool (strict)"("Val(Sgnl)"=TRUE ("Value (Signaling)")) -> ()  [unwired: 2 in, 2 out]
              }
            }
            n729 = local write "Stage moving"(TRUE ("Stage moving")) -> ()
            n730 = call "move to saved stage position.vi"("error in"=w1155, "Stage VISA resource name in"=w1156, "Position"=1, "Saved Stage Positions"=w1158) -> ()  [unwired: 2 out]
          }
          frame #1 {
            n731 = local read "Shutter 1 (B)"() -> (w1162:bool)
            n732 = disable-structure shown="Disabled" {
              frame Disabled {
                n733 = property on="Inject Pump 2" class="Bool (strict)"("Val(Sgnl)"=TRUE ("Inject Pump 2")) -> ()  [unwired: 2 in, 2 out]
              }
              frame Enabled {
              }
            }
            n734 = local write "Stage moving"(FALSE ("Stage moving")) -> ()
            n735 = case shown="False" w1162 {
              frame False {
                n736 = property on="Shutter 1 (B)" class="Bool (strict)"("Val(Sgnl)"=TRUE ("Value (Signaling)")) -> ()  [unwired: 2 in, 2 out]
              }
              frame True {
              }
            }
            n737 = property on="Inject Sample" class="Bool (strict)"("Val(Sgnl)"=FALSE ("Value (Signaling)")) -> ()  [unwired: 2 in, 2 out]
            n738 = call <vilib>:"Beep.vi"() -> ()  [unwired: 12 in]
          }
        }
        n739 = local write "Got ADig bead"(FALSE ("Got ADig bead")) -> ()
      }
      event "Set Position 1", "Set Position 2", "Set Position 3", "Set Position 4", "Set Position 5": Value Change {
        n740 = event-data() -> ()  [unwired: 1 in, 5 out]
        n741 = Build Array("Set Position 1", "Set Position 2", "Set Position 3", "Set Position 4", "Set Position 5") -> (w1181:bool[])
        n742 = Boolean Array To Number(Boolean array=w1181) -> (number=w1180:u32)
        n743 = call "Read Stage Position.vi"("error in"=w1168, "VISA resource name in"=w1169) -> ("Current Position"=w1166:cluster{dbl, dbl, dbl}, "error out"=→"Stage error":errorcluster)  [unwired: 1 in, 1 out]
        n744 = Logarithm Base 2(1:w1180) -> (0:w1174:dbl)
        n745 = Cluster To Array(cluster=w1166) -> (array=w1176:dbl[])
        n746 = Increment(x=w1174) -> (x+1=w1177:dbl)
        n747 = Build Array (concatenate)(w1177, w1176) -> (w1175:dbl[])
        n748 = Replace Array Subset(array="Saved stage positions", new element=w1175, index (row)=w1174) -> (w1178:dbl[][])  [unwired: 1 in]
        n749 = local write "Saved stage positions"(w1178) -> ()
      }
      event "Move to Position 2", "Move to Position 4", "Move to Position 3", "Move to Position 5", "Move to Position 1": Value Change {
        n750 = event-data() -> ()  [unwired: 1 in, 5 out]
        n751 = Build Array("Move to Position 1", "Move to Position 2", "Move to Position 3", "Move to Position 4", "Move to Position 5") -> (w1191:bool[])
        n752 = Boolean Array To Number(Boolean array=w1191) -> (number=w1190:u32)
        n753 = Logarithm Base 2(1:w1190) -> (0:w1189:dbl)
        n754 = flat-sequence {
          tunnel: w1189 -> [w1196]
          tunnel: w1188 -> [w1195]
          tunnel: w1187 -> [w1194]
          frame #0 {
            n755 = local read "Saved stage positions"() -> (w1197:dbl[][])
            n756 = Increment(x=w1196) -> (x+1=w1193:dbl)
            n757 = call "move to saved stage position.vi"("error in"=w1194, "Stage VISA resource name in"=w1195, "Position"=w1193, "Saved Stage Positions"=w1197) -> ()  [unwired: 2 out]
            "Stage moving" <- TRUE ("Stage moving")
          }
          frame #1 {
            n758 = call <vilib>:"Beep.vi"() -> ()  [unwired: 12 in]
            n759 = local write "Stage moving"(FALSE ("Stage moving")) -> ()
          }
        }
      }
      event "Set Current\nPos to (0,0,0)": Value Change {
        w1201 = ";" ("string")
        # "DH is \"Define Home\" -KW"
        n760 = event-data() -> ()  [unwired: 1 in, 5 out]
        n761 = local write "Set Current\nPos to (0,0,0)"(FALSE ("Set Current\nPos to (0,0,0)")) -> ()
        n762 = call-poly "VISA Configure Serial Port"("VISA resource name"=w1211, "baud rate (9600)"=u32 19200, "error in (no error)"=w1210) -> ("VISA resource name out"=w1205:refnum<visa-resource-name>, "error out"=w1204:errorcluster)  [unwired: 11 in]
        n763 = Concatenate Strings("1DH" ("string"), w1201, "2DH" ("string"), w1201, "3DH" ("string"), "\r") -> (w1203:string)
        n764 = VISA Write(VISA resource name=w1205, write buffer=w1203, error in (no error)=w1204) -> (error out=w1202:errorcluster)  [unwired: 2 out]
        n765 = local write "Stage error"(w1202) -> ()
      }
      event "Dip": Value Change {
        n766 = event-data() -> ()  [unwired: 1 in, 5 out]
        n767 = local write "Dip"(FALSE ("Dip")) -> ()
        n768 = flat-sequence {
          tunnel: w1221 -> [w1223]
          tunnel: w1220 -> [w1222]
          tunnel: [w1224] -> w1218
          tunnel: [w1223] -> w1216
          tunnel: [w1222] -> w1214
          tunnel: [w1232] -> w1219
          tunnel: w1218 -> [w1232]
          tunnel: [w1231] -> w1217
          tunnel: w1216 -> [w1231]
          tunnel: [w1230] -> w1215
          tunnel: w1214 -> [w1230]
          tunnel: w1219 -> [w1251]
          tunnel: w1217 -> [w1250]
          tunnel: w1215 -> [w1249]
          frame #0 {
            n769 = local read "Saved stage positions"() -> (w1224:dbl[][])
            n770 = local write "Stage moving"(TRUE) -> ()
            n771 = call "move to saved stage position.vi"("error in"=w1222, "Stage VISA resource name in"=w1223, "Position"="Dip position", "Saved Stage Positions"=w1224) -> ()  [unwired: 2 out]
          }
          frame #1 {
            n772 = node-c288() -> (w1229:T11)  [unwired: 4 in]
            n773 = timed-loop {
              timing: w1229 -> [_]
              timing-out: [_] -> w1228
              i -> [w1242]
              stop <- w1233 stop-if-true
              n774 = node-c288() -> ()  [unwired: 1 in, 1 out]
              n775 = Greater Or Equal?(x=w1242, y="Dip duration") -> (x >= y?=w1238:bool)
              n776 = local read "Dump beads"() -> (w1235:bool)
              n777 = Or(x=w1238, y="Cancel dwell") -> (x .or. y?=w1236:bool)
              n778 = Not(x="Pause dwell") -> (.not. x?=w1239:bool)
              n779 = node-c288() -> ()  [unwired: 1 in, 1 out]
              n780 = And(x=w1239, y=w1236) -> (x .and. y?=w1234:bool)
              n781 = Or(x=w1234, y=w1235) -> (x .or. y?=w1233:bool)
              "Dip time" <- w1242
            }
            n782 = local write "Stage moving"(FALSE ("Stage moving")) -> ()
            n783 = node-c288(w1228) -> ()  [unwired: 1 out]
          }
          frame #2 {
            n784 = local write "Cancel dwell"(FALSE ("Cancel dwell")) -> ()
            n785 = call "move to saved stage position.vi"("error in"=w1249, "Stage VISA resource name in"=w1250, "Position"="Return position", "Saved Stage Positions"=w1251) -> ()  [unwired: 2 out]
          }
          frame #3 {
            n786 = local write "Stage moving"(FALSE ("Stage moving")) -> ()
          }
        }
      }
      event "Force FB script": Value Change {
        n787 = event-data() -> ()  [unwired: 1 in, 5 out]
        n788 = flat-sequence {
          frame #0 {
            n789 = disable-structure shown="Disabled" {
              frame Disabled {
                n790 = local read "# Samples/channel"() -> (w1255:i32)
                n791 = local write "# Samples/channel (in)"(w1255) -> ()
              }
              frame Enabled {
              }
            }
            n792 = local write "Force FB script"(FALSE ("Force FB script")) -> ()
            n793 = property on="Trap delta (nm)" class="DigNum (strict)"("Val(Sgnl)"="Start trap delta (nm)") -> ()  [unwired: 2 in, 2 out]
          }
          frame #1 {
            n794 = Wait (ms)(milliseconds to wait=u32 500) -> ()  [unwired: 1 out]
          }
          frame #2 {
            n795 = property on="Set reading to\nsetpoint" class="Bool (strict)"("Val(Sgnl)"=TRUE ("Value (Signaling)")) -> ()  [unwired: 2 in, 2 out]
          }
          frame #3 {
            n796 = Wait (ms)(milliseconds to wait=u32 300) -> ()  [unwired: 1 out]
          }
          frame #4 {
            n797 = local write "Force Feedback"(TRUE ("Force Feedback")) -> ()
            n798 = property on="Tabs" class="TabCtl (strict)"("Val(Sgnl)"=T4."Force Feedback" ("Value (Signaling)")) -> ()  [unwired: 2 in, 2 out]
          }
          frame #5 {
            n799 = property on="Save Data" class="Bool (strict)"("Val(Sgnl)"=TRUE ("Value (Signaling)")) -> ()  [unwired: 2 in, 2 out]
          }
          frame #6 {
            n800 = Multiply(x="Wait before dip (s)", y=1000) -> (x*y=w1262:dbl)
            n801 = Wait (ms)(milliseconds to wait=w1262) -> ()  [unwired: 1 out]
          }
          frame #7 {
            n802 = case shown="True" "Start dipping after?" {
              selector: "Start dipping after?" -> [_ w1267]
              frame False {
              }
              frame True {
                n803 = property on="Dip" class="Bool (strict)"("Val(Sgnl)"=w1267) -> ()  [unwired: 2 in, 2 out]
              }
            }
            n804 = property on="Remove offsets" class="Bool (strict)"("Val(Sgnl)"=TRUE ("Value (Signaling)")) -> ()  [unwired: 2 in, 2 out]
          }
        }
      }
      event "Move 0": Value Change {
        n805 = event-data() -> ()  [unwired: 1 in, 5 out]
        n806 = local write "Move 0"(FALSE) -> ()
        n807 = call "HalfWavePlate.vi"("Degrees"="\"Degrees\" 0", "Motor"=0) -> ()  [unwired: 1 in]
      }
      event "Move 1": Value Change {
        n808 = event-data() -> ()  [unwired: 1 in, 5 out]
        n809 = local write "Move 1"(FALSE) -> ()
        n810 = call "HalfWavePlate.vi"("Degrees"="\"Degrees\" 1", "Motor"=1) -> ()  [unwired: 1 in]
      }
      event "Save user params": Value Change {
        n811 = event-data() -> ()  [unwired: 1 in, 6 out]
        n812 = local write "Save user params"(FALSE) -> ()
        n813 = call "save control values.vi"("User"="User") -> ()  [unwired: 8 in, 1 out]
      }
      event "Load user params": Value Change {
        # "Exceptions. Don't load these parameters."
        n814 = event-data() -> ()  [unwired: 1 in, 6 out]
        n815 = local write "Load user params"(FALSE) -> ()
        n816 = flat-sequence {
          tunnel: [w1297] -> w1289
          tunnel: [w1296] -> w1287
          tunnel: [w1295] -> w1285
          tunnel: [w1294] -> w1283
          tunnel: [w1293] -> w1281
          tunnel: [w1292] -> w1279
          tunnel: [w1291] -> w1277
          tunnel: [w1304] -> w1290
          tunnel: w1289 -> [w1304]
          tunnel: [w1303] -> w1288
          tunnel: w1287 -> [w1303]
          tunnel: [w1302] -> w1286
          tunnel: w1285 -> [w1302]
          tunnel: [w1301] -> w1284
          tunnel: w1283 -> [w1301]
          tunnel: [w1300] -> w1282
          tunnel: w1281 -> [w1300]
          tunnel: [w1299] -> w1280
          tunnel: w1279 -> [w1299]
          tunnel: [w1298] -> w1278
          tunnel: w1277 -> [w1298]
          tunnel: w1290 -> [w1312]
          tunnel: w1288 -> [w1311]
          tunnel: w1286 -> [w1310]
          tunnel: w1284 -> [w1309]
          tunnel: w1282 -> [w1308]
          tunnel: w1280 -> [w1307]
          tunnel: w1278 -> [w1306]
          frame #0 {
            n817 = local read "Shutter 1 (B)"() -> (w1297:bool)
            n818 = local read "Shutter 2 (A)"() -> (w1296:bool)
            n819 = local read "Inject Sample"() -> (w1294:bool)
            n820 = local read "Trap delta (nm)"() -> (w1293:dbl)
            n821 = local read "Save file index"() -> (w1292:i32)
            n822 = local read "Force Feedback"() -> (w1291:bool)
            n823 = local read "Fish"() -> (w1295:bool)
          }
          frame #1 {
            n824 = local read "User"() -> (w1305:string)
            n825 = call "retrieve control values.vi"("User"=w1305) -> ()  [unwired: 10 in, 1 out]
          }
          frame #2 {
            n826 = local write "Trap delta (nm)"(w1308) -> ()
            n827 = local write "Save file index"(w1307) -> ()
            n828 = local write "Force Feedback"(w1306) -> ()
            n829 = local write "Inject Sample"(w1309) -> ()
            n830 = local write "Shutter 2 (A)"(w1311) -> ()
            n831 = local write "Shutter 1 (B)"(w1312) -> ()
            n832 = local write "Fish"(w1310) -> ()
          }
        }
      }
      event "Stop": Value Change {
        n833 = event-data() -> ()  [unwired: 1 in, 5 out]
        n834 = local read "Stop"() -> (w1313:bool)
      }
    }
    n835 = node-c288() -> ()  [unwired: 1 in, 1 out]
  }
  n836 = node-c288(2 ("Processor")) -> (w71:T11)  [unwired: 3 in]
  n837 = node-c288(2 ("Processor")) -> (w23:T11)  [unwired: 3 in]
  n838 = timed-loop {
    timing: w71 -> [_]
    timing-out: [_] -> w70
    stop <- w1316 stop-if-true
    n839 = node-c288() -> ()  [unwired: 1 in, 1 out]
    n840 = case shown="\"Current Saved Data\"" "Tab Control" {
      frame "Control" {
        n841 = case shown="True" "Start" {
          frame False {
          }
          frame True {
            w1329 = T19 3 items=["no dialog", "OK message", "continue or stop message", "OK message + warnings", "continue/stop + warnings"] ("type of dialog (OK msg:1)")
            n842 = call "InitializeAcquireFF.vi"("DAQ Rate"="DAQ Rate", "Averaging Number"="Averaging Number", "Sampling Rate"="Sampling Rate") -> ("error out"=w1323:errorcluster, "task out"=w1322:refnum<k21>, "Final Sampling Rate"=→"Final Sampling Rate":dbl)  [unwired: 4 in, 2 out]
            n843 = while {
              tunnel: [w1341] -> w1328
              tunnel: [w1340] -> w1321
              tunnel: "Averaging Number" -> [w1339]
              tunnel: w1323 -> [w1338]
              tunnel: w1322 -> [w1336]
              stop <- w1337 continue-if-true
              n844 = call "Acquire2_QPD.vi"("task/channels in"=w1336, "Save Data?"=FALSE ("Take Data?"), "Averaging Number"=w1339, "error in"=w1338) -> ("PSD 1"=→"PSD 1":cluster{dbl[], dbl[]}, "PSD 1 Sum"=→"PSD 1 Sum":dbl, "PSD 2"=→"PSD 2":cluster{dbl[], dbl[]}, "PSD 2 Sum"=→"PSD 2 Sum":dbl, "task out"=w1341:refnum<k21>, "error out"=w1340:errorcluster)  [unwired: 14 in, 4 out]
              n845 = local read "Start"() -> (w1337:bool)
            }
            n846 = call <vilib>:"DAQmx Clear Task.vi"("task in"=w1328, "error in"=w1321) -> ("error out"=w1330:errorcluster)  [unwired: 13 in]
            n847 = call <vilib>:"Simple Error Handler.vi"("type of dialog (OK msg:1)"=w1329, "error in (no error)"=w1330) -> ()  [unwired: 3 in, 5 out]
          }
        }
      }
      frame "Current Saved Data" {
      }
      frame "Data Acquisition" {
      }
      frame "Raw QPD Data" {
      }
    }
    n848 = local read "Stop"() -> (w1316:bool)
    n849 = node-c288() -> ()  [unwired: 1 in, 1 out]
  }
  n850 = call-poly <vilib>:"DAQmx Create Virtual Channel.vi"("lines"=w88) -> ("task out"=w87:refnum<k21>)  [unwired: 13 in, 1 out]
  n851 = call-poly <vilib>:"DAQmx Create Virtual Channel.vi"("lines"=w91) -> ("task out"=w90:refnum<k21>)  [unwired: 13 in, 1 out]
  n852 = timed-loop {
    timing: w23 -> [_]
    timing-out: [_] -> w22
    stop <- w1342 stop-if-true
    n853 = node-c288() -> ()  [unwired: 1 in, 1 out]
    n854 = event shown="[0] \"Pause Mouse/Mirror Connection\": Value Change" {
      selector: _ -> [_ _]
      dyn-events: _ -> [_ _]
      timeout: _ -> [_ _]
      tunnel: [w1435 _] -> w1343
      tunnel: [_ w1436] -> w1342
      event "Pause Mouse/Mirror Connection": Value Change {
        n855 = event-data() -> ("NewVal"=w1435:bool)  [unwired: 1 in]
      }
      event "Stop": Value Change {
        n856 = event-data() -> ("NewVal"=w1436:bool)  [unwired: 1 in]
      }
    }
    n857 = case shown="True" w1343 {
      frame False {
      }
      frame True {
        n858 = call "InitializeMouseControl.vi"() -> ("error out 2"=w1352:errorcluster, "task out"=w1353:refnum<k21>, "error out"=w1355:errorcluster, "device ID"=w1354:refnum<k1>)  [unwired: 8 in]
        n859 = while {
          tunnel: w1355 -> [w1367]
          tunnel: w1354 -> [w1366]
          tunnel: w1353 -> [w1365]
          tunnel: w1352 -> [w1364]
          tunnel: [w1363] -> w1350
          tunnel: [w1362] -> w1349
          tunnel: [w1361] -> w1346
          tunnel: [w1360] -> w1347
          stop <- w1359 stop-if-true
          n860 = case shown="True" "Use Mouse to Move Trap?" {
            tunnel: w1366 -> [w1374 w1397]
            tunnel: w1367 -> [w1373 w1396]
            tunnel: w1365 -> [w1372 w1395]
            tunnel: w1364 -> [w1371 w1394]
            tunnel: [w1374 w1393] -> w1361
            tunnel: [w1373 w1392] -> w1360
            tunnel: [w1372 w1391] -> w1363
            tunnel: [w1371 w1390] -> w1362
            frame False {
              (unwired) FALSE ("button 1")
            }
            frame True {
              w1385 = 0.0 ("y")
              w1387 = 10
              n861 = local read "Deflection"() -> (w1398:T5)
              n862 = call-poly <vilib>:"Acquire Input Data.vi"("device ID"=w1397, "error in (no error)"=w1396) -> ("device ID"=w1393:refnum<k1>, "button info"=w1411:T20, "error out"=w1392:errorcluster)  [unwired: 14 in, 1 out]
              n863 = Unbundle By Name(w1398) -> ("Horizontal"=w1400:i32, "Vertical"=w1399:i32)
              n864 = local read "Saved voltage"() -> (w1376:cluster{dbl, dbl})
              n865 = Divide(x=w1400, y=30) -> (x/y=w1403:dbl)
              n866 = Divide(x=w1399, y=-20) -> (x/y=w1404:dbl)
              n867 = Unbundle By Name(w1411) -> ("button 1"=w1389:bool, "button 2"=w1405:bool)
              n868 = Bundle(w1403, w1404) -> (w1381:cluster{dbl, dbl})  [unwired: 1 in]
              n869 = local write "Reference Voltage"(w1381) -> ()
              n870 = Add(x=w1381, y=w1376) -> (x+y=w1409:cluster{dbl, dbl})
              n871 = case shown="True" w1389 {
                frame False {
                  n872 = stacked-sequence {
                    frame #0 {
                      n873 = local write "CoordinatesMousePressed"(T5 {"Horizontal"=0, "Vertical"=0} ("Coords when pressed")) -> ()
                      n874 = local write "Deflection"(T5 {"Horizontal"=0, "Vertical"=0} ("deflaction")) -> ()
                    }
                  }
                }
                frame True {
                  n875 = local read "CoordinatesMousePressed"() -> (w1434:T5)
                  n876 = local read "Real Coordinates"() -> (w1433:cluster{"Horizontal":i32, "Vertical":i32})
                  n877 = Subtract(x=w1433, y=w1434) -> (x-y=w1432:T5)
                  n878 = local write "Deflection"(w1432) -> ()
                }
              }
              n879 = Unbundle(w1409) -> (w1386:dbl, w1377:dbl)
              n880 = case shown="True" w1405 {
                frame False {
                }
                frame True {
                  n881 = local read "Reference Voltage"() -> (w1415:cluster{dbl, dbl})
                  n882 = local read "Saved voltage"() -> (w1413:cluster{dbl, dbl})
                  n883 = Add(x=w1415, y=w1413) -> (x+y=→"Saved voltage":cluster{dbl, dbl})
                  n884 = local read "Real Coordinates"() -> (w1414:cluster{"Horizontal":i32, "Vertical":i32})
                  n885 = local write "CoordinatesMousePressed"(w1414) -> ()
                }
              }
              n886 = Less?(x=w1386, y=w1387) -> (x < y?=w1384:bool)
              n887 = Greater?(x=w1386, y=w1385) -> (0:w1383:bool)
              n888 = Greater?(x=w1377, y=w1385) -> (0:w1379:bool)
              n889 = Less?(x=w1377, y=w1387) -> (x < y?=w1380:bool)
              n890 = And(x=w1379, y=w1380) -> (x .and. y?=w1378:bool)
              n891 = And(x=w1384, y=w1383) -> (x .and. y?=w1382:bool)
              n892 = case shown="False" w1378 {
                tunnel: [w1425 w1429] -> w1388
                tunnel: w1377 -> [w1423 w1429]
                frame False {
                  n893 = Greater?(x=w1423, y=10.0) -> (0:w1426:bool)
                  n894 = case shown="True" w1426 {
                    tunnel: [0.0 10.0] -> w1425
                    frame False {
                    }
                    frame True {
                    }
                  }
                }
                frame True {
                }
              }
              n895 = case shown="False" w1382 {
                tunnel: w1386 -> [w1417 w1422]
                tunnel: [w1418 w1422] -> w1410
                frame False {
                  n896 = Greater?(x=w1417, y=10.0) -> (0:w1419:bool)
                  n897 = case shown="True" w1419 {
                    tunnel: [0.0 10.0] -> w1418
                    frame False {
                    }
                    frame True {
                    }
                  }
                }
                frame True {
                }
              }
              n898 = Bundle(w1410, w1388) -> (w1375:cluster{dbl, dbl})  [unwired: 1 in]
              n899 = Cluster To Array(cluster=w1375) -> (array=w1406:dbl[])
              n900 = call-poly <vilib>:"DAQmx Write.vi"("task/channels in"=w1395, "data"=w1406, "error in"=w1394) -> ("task out"=w1408:refnum<k21>, "error out"=w1407:errorcluster)  [unwired: 10 in, 1 out]
              n901 = call <vilib>:"DAQmx Is Task Done.vi"("task/channels in"=w1408, "error in"=w1407) -> ("task out"=w1391:refnum<k21>, "error out"=w1390:errorcluster)  [unwired: 11 in, 1 out]
            }
          }
          n902 = event shown="[0] \"Pane\": Mouse Move" {
            selector: _ -> [_ _ _]
            dyn-events: _ -> [_ _ _]
            timeout: _ -> [_ _ _]
            event Mouse Move {
              n903 = event-data() -> ("Coords"=w1369:T5)  [unwired: 1 in]
              n904 = local write "Real Coordinates"(w1369) -> ()
            }
            event Mouse Down {
              n905 = event-data() -> ("Coords"=w1370:T5)  [unwired: 1 in]
              n906 = local write "CoordinatesMousePressed"(w1370) -> ()
            }
            event "Pause Mouse/Mirror Connection": Value Change {
              n907 = event-data() -> ()  [unwired: 1 in, 3 out]
            }
          }
          n908 = local read "Stop"() -> (w1356:bool)
          n909 = Not(x="Pause Mouse/Mirror Connection") -> (.not. x?=w1357:bool)
          n910 = Or(x=w1357, y=w1356) -> (x .or. y?=w1359:bool)
        }
        n911 = call <vilib>:"DAQmx Clear Task.vi"("task in"=w1350, "error in"=w1349) -> ("error out"=w1351:errorcluster)  [unwired: 13 in]
        n912 = call <vilib>:"Simple Error Handler.vi"("error in (no error)"=w1351) -> ()  [unwired: 4 in, 5 out]
        n913 = call-poly <vilib>:"Close Input Device.vi"("error in (no error)"=w1347, "device ID"=w1346) -> ("error out"=w1348:errorcluster)  [unwired: 8 in]
        n914 = call <vilib>:"Simple Error Handler.vi"("error in (no error)"=w1348) -> ()  [unwired: 4 in, 5 out]
      }
    }
    n915 = node-c288() -> ()  [unwired: 1 in, 1 out]
  }
  n916 = node-c288(i64 100 ("Period")) -> (w85:T11)  [unwired: 3 in]
  n917 = timed-loop {
    tunnel: w87 -> [w1439]
    tunnel: [w1438] -> w86
    tunnel: w90 -> [w1441]
    tunnel: [w1440] -> w89
    timing: w85 -> [_]
    timing-out: [_] -> w84
    stop <- w1437 stop-if-true
    n918 = node-c288() -> ()  [unwired: 1 in, 1 out]
    n919 = event shown="[1] \"Shutter 2 (A)\": Value Change" {
      selector: _ -> [_ _ _]
      dyn-events: _ -> [_ _ _]
      timeout: _ -> [_ _ _]
      tunnel: w1441 -> [w1445 _ _]
      tunnel: [w1444 _ _] -> w1440
      tunnel: w1439 -> [_ w1465 _]
      tunnel: [_ w1463 _] -> w1438
      tunnel: [_ _ w1482] -> w1437
      event "Shutter 1 (B)": Value Change {
        n920 = event-data() -> ()  [unwired: 1 in, 1 out]
        n921 = flat-sequence {
          tunnel: [w1451] -> w1448
          tunnel: w1445 -> [w1450]
          tunnel: [w1455] -> w1447
          tunnel: [w1458] -> w1446
          tunnel: w1448 -> [w1453]
          tunnel: w1447 -> [w1462]
          tunnel: w1446 -> [w1460]
          tunnel: [w1459] -> w1444
          frame #0 {
            n922 = call-poly <vilib>:"DAQmx Write.vi"("task/channels in"=w1450, "data"=FALSE) -> ("task out"=w1451:refnum<k21>)  [unwired: 11 in, 2 out]
            n923 = Wait (ms)(milliseconds to wait=100) -> ()  [unwired: 1 out]
          }
          frame #1 {
            n924 = Or(x="Shutter 1 (B)", y=TRUE) -> (x .or. y?=w1455:bool)
            n925 = call-poly <vilib>:"DAQmx Write.vi"("task/channels in"=w1453, "data"=w1455) -> ("task out"=w1458:refnum<k21>)  [unwired: 11 in, 2 out]
            n926 = Wait (ms)(milliseconds to wait=100) -> ()  [unwired: 1 out]
          }
          frame #2 {
            n927 = Not(x=w1462) -> (.not. x?=w1461:bool)
            n928 = call-poly <vilib>:"DAQmx Write.vi"("task/channels in"=w1460, "data"=w1461) -> ("task out"=w1459:refnum<k21>)  [unwired: 11 in, 2 out]
          }
        }
      }
      event "Shutter 2 (A)": Value Change {
        n929 = event-data() -> ()  [unwired: 1 in, 1 out]
        n930 = flat-sequence {
          tunnel: w1465 -> [w1470]
          tunnel: [w1469] -> w1464
          tunnel: [w1474] -> w1467
          tunnel: [w1477] -> w1466
          tunnel: w1464 -> [w1472]
          tunnel: w1467 -> [w1481]
          tunnel: w1466 -> [w1479]
          tunnel: [w1478] -> w1463
          frame #0 {
            n931 = call-poly <vilib>:"DAQmx Write.vi"("task/channels in"=w1470, "data"=FALSE) -> ("task out"=w1469:refnum<k21>)  [unwired: 11 in, 2 out]
            n932 = Wait (ms)(milliseconds to wait=100) -> ()  [unwired: 1 out]
          }
          frame #1 {
            n933 = Or(x="Shutter 2 (A)", y=TRUE) -> (x .or. y?=w1474:bool)
            n934 = call-poly <vilib>:"DAQmx Write.vi"("task/channels in"=w1472, "data"=w1474) -> ("task out"=w1477:refnum<k21>)  [unwired: 11 in, 2 out]
            n935 = Wait (ms)(milliseconds to wait=100) -> ()  [unwired: 1 out]
          }
          frame #2 {
            n936 = Not(x=w1481) -> (.not. x?=w1480:bool)
            n937 = call-poly <vilib>:"DAQmx Write.vi"("task/channels in"=w1479, "data"=w1480) -> ("task out"=w1478:refnum<k21>)  [unwired: 11 in, 2 out]
          }
        }
      }
      event "Stop": Value Change {
        n938 = event-data() -> ("NewVal"=w1482:bool)  [unwired: 1 in, 5 out]
      }
    }
    n939 = node-c288() -> ()  [unwired: 1 in, 1 out]
  }
  n940 = node-c288(w84) -> ()  [unwired: 1 out]
  n941 = node-c288(w70) -> ()  [unwired: 1 out]
  n942 = call <vilib>:"DAQmx Clear Task.vi"("task in"=w86) -> ()  [unwired: 14 in, 1 out]
  n943 = call <vilib>:"DAQmx Clear Task.vi"("task in"=w89) -> ()  [unwired: 14 in, 1 out]
  n944 = node-c288(w22) -> ()  [unwired: 1 out]
  n945 = node-c288(w18) -> ()  [unwired: 1 out]
  n946 = local write "Tether"(FALSE ("Tether")) -> ()
  n947 = local read "Path"() -> (w77:path)
  n948 = node-c288(i64 1 ("Period"), 2 ("Processor")) -> (w83:T11)  [unwired: 2 in]
  n949 = VISA Close(VISA resource name=w15) -> (error out=w95:errorcluster)  [unwired: 1 in]
  n950 = timed-loop {
    timing: w83 -> [_]
    timing-out: [_] -> w82
    tunnel: w77 -> [w1484]
    stop <- w1483 stop-if-true
    n951 = node-c288() -> ()  [unwired: 1 in, 1 out]
    n952 = event shown="[5] \"Fish\": Value Change" {
      selector: _ -> [_ _ _ _ _ _ _ _ _ _]
      dyn-events: _ -> [_ _ _ _ _ _ _ _ _ _]
      timeout: _ -> [_ _ _ _ _ _ _ _ _ _]
      tunnel: w1484 -> [_ w1488 _ _ _ _ _ _ _ _]
      tunnel: [_ _ w1508 _ _ _ _ _ _ _] -> w1483
      event Timeout {
        n953 = event-data() -> ()  [unwired: 1 in, 2 out]
      }
      event "Read Cal": Value Change {
        n954 = event-data() -> ()  [unwired: 1 in, 6 out]
        n955 = Path To String(path=w1488) -> (string=w1487:string)
        n956 = Format Date/Time String(time format string (%c)="%y%m%d") -> (date/time string=w1489:string)  [unwired: 2 in]
        n957 = Concatenate Strings(w1487, "\\" ("string"), w1489, "\\" ("string"), "current.cal") -> (w1507:string)
        n958 = String To Path(string=w1507) -> (path=w1506:path)
        n959 = Open/Create/Replace File(file path (use dialog)=w1506, operation (0:open)=T16."open", access (0:read/write)=enum16{"read/write", "read-only", "write-only"}."read-only") -> (refnum out=w1502:refnum<file>, error out=w1503:errorcluster)  [unwired: 3 in, 1 out]
        n960 = Deny Access(4:w1503, 7:w1502) -> (0:w1501:errorcluster, 3:w1500:refnum<file>)  [unwired: 1 in]
        n961 = Read from Binary File(5:0.0, 8:w1501, 9:T17."big-endian, network order" ("byte order (0:big-endian, network order)"), 10:12 ("count"), 11:w1500) -> (0:w1496:errorcluster, 2:w1494:dbl[], 3:w1497:refnum<file>)  [unwired: 1 in, 1 out]
        n962 = Array To Cluster(array=w1494) -> (cluster=→"Cal values":T21)
        n963 = Close File(refnum=w1497, error in=w1496) -> ()  [unwired: 2 out]
        n964 = local write "Read Cal"(FALSE ("Read Cal")) -> ()
      }
      event "Stop": Value Change {
        n965 = event-data() -> ("NewVal"=w1508:bool)  [unwired: 1 in, 5 out]
      }
      event "Trap position (V)": Value Change {
        # "Need to rotate so X and Y don't get mixed up."
        n966 = event-data() -> ()  [unwired: 1 in, 6 out]
        n967 = local read "Mirror task"() -> (w1509:refnum<k21>)
        n968 = Cluster To Array(cluster="Trap position (V)") -> (array=w1512:dbl[])
        n969 = Rotate 1D Array(1:w1512, 2:1 ("n")) -> (0:w1510:dbl[])
        n970 = call-poly <vilib>:"DAQmx Write.vi"("task/channels in"=w1509, "data"=w1510) -> ("task out"=w1515:refnum<k21>, "error out"=w1514:errorcluster)  [unwired: 11 in, 1 out]
        n971 = call <vilib>:"DAQmx Stop Task.vi"("task/channels in"=w1515, "error in"=w1514) -> ("error out"=w1513:errorcluster)  [unwired: 12 in, 1 out]
        n972 = call <vilib>:"Simple Error Handler.vi"("error in (no error)"=w1513) -> ()  [unwired: 4 in, 5 out]
      }
      event "Trap delta (nm)": Value Change {
        n973 = event-data() -> ()  [unwired: 1 in, 6 out]
        n974 = local read "Pulling direction"() -> (w1517:bool)
        n975 = local read "Conv Y (nm/V)"() -> (w1518:dbl)
        n976 = local read "Conv X (nm/V)"() -> (w1519:dbl)
        n977 = Select(t=w1518, s=w1517, f=w1519) -> (s? t:f=w1520:dbl)
        n978 = local read "Fixed Y"() -> (w1526:dbl)
        n979 = Divide(x="Trap delta (nm)", y=w1520) -> (x/y=w1521:dbl)
        n980 = local read "Fixed X"() -> (w1525:dbl)
        n981 = Select(t=w1526, s=w1517, f=w1525) -> (s? t:f=w1524:dbl)
        n982 = Add(x=w1521, y=w1524) -> (x+y=w1522:dbl)
        n983 = case shown="False" w1517 {
          tunnel: w1522 -> [w1527 w1528]
          frame False {
            n984 = property on="X" class="DigNum (strict)"("Val(Sgnl)"=w1527) -> ()  [unwired: 2 in, 2 out]
          }
          frame True {
            n985 = property on="Y" class="DigNum (strict)"("Val(Sgnl)"=w1528) -> ()  [unwired: 2 in, 2 out]
          }
        }
      }
      event "Fish": Value Change {
        n986 = event-data() -> ()  [unwired: 1 in, 6 out]
        n987 = local read "Fish"() -> (w1529:bool)
        n988 = case shown="True" w1529 {
          frame False {
          }
          frame True {
            w1538 = 0.0 ("minimum value")
            w1539 = 10.0 ("maximum value")
            # "Grab offset in pulling\ndirection and add to \ndelta values"
            n989 = call-poly <vilib>:"DAQmx Create Virtual Channel.vi"("maximum value"=w1539, "minimum value"=w1538, "physical channels"=tag "Dev1/ao0") -> ("task out"=w1543:refnum<k21>, "error out"=w1542:errorcluster)  [unwired: 11 in]
            n990 = call-poly <vilib>:"DAQmx Create Virtual Channel.vi"("task in"=w1543, "maximum value"=w1539, "minimum value"=w1538, "physical channels"=tag "Dev1/ao1", "error in"=w1542) -> ("task out"=w1537:refnum<k21>, "error out"=w1536:errorcluster)  [unwired: 9 in]
            n991 = node-c288(i64 1 ("Period")) -> (w1545:T11)  [unwired: 3 in]
            n992 = timed-loop {
              timing: w1545 -> [_]
              timing-out: [_] -> w1544
              tunnel: w1537 -> [w1613]
              tunnel: w1536 -> [w1612]
              tunnel: [w1611] -> w1532
              tunnel: [w1610] -> w1531
              tunnel: [w1570] -> w1534
              tunnel: [w1571] -> w1530
              i -> [w1596]
              stop <- w1571 stop-if-true
              # "x direction"
              # "y direction"
              # "Send offset in direction\nof not-pulling to DAQ"
              n993 = node-c288() -> ()  [unwired: 1 in, 1 out]
              n994 = local read "Pulling direction"() -> (w1575:bool)
              n995 = local read "Conv Y (nm/V)"() -> (w1577:dbl)
              n996 = local read "Conv X (nm/V)"() -> (w1576:dbl)
              n997 = local read "Fixed X"() -> (w1584:dbl)
              n998 = local read "Fixed Y"() -> (w1583:dbl)
              n999 = Select(t=w1583, s=w1575, f=w1584) -> (s? t:f=w1585:dbl)
              n1000 = Select(t=w1584, s=w1575, f=w1583) -> (s? t:f=w1582:dbl)
              n1001 = Select(t=w1577, s=w1575, f=w1576) -> (s? t:f=w1572:dbl)
              n1002 = Divide(x="Max fish\ndelta (nm)", y=w1572) -> (x/y=w1574:dbl)
              n1003 = Divide(x="Min fish\ndelta (nm)", y=w1572) -> (x/y=w1573:dbl)
              n1004 = Add(x=w1585, y=w1574) -> (x+y=w1587:dbl)
              n1005 = Subtract(x=w1574, y=w1573) -> (x-y=w1589:dbl)
              n1006 = Divide(x=w1589, y="Fish Speed (ms)") -> (x/y=w1590:dbl)
              n1007 = flat-sequence {
                tunnel: w1575 -> [w1633]
                tunnel: w1582 -> [w1632]
                tunnel: w1613 -> [w1631]
                tunnel: w1612 -> [w1630]
                tunnel: w1590 -> [w1629]
                tunnel: w1587 -> [w1628]
                tunnel: "Fish Speed (ms)" -> [w1623]
                tunnel: [w1627] -> w1609
                tunnel: [w1626] -> w1608
                tunnel: [w1625] -> w1607
                tunnel: [w1624] -> w1606
                tunnel: [w1617] -> w1595
                tunnel: [w1616] -> w1581
                tunnel: [w1615] -> w1578
                tunnel: [w1614] -> w1568
                tunnel: [w1686] -> w1605
                tunnel: w1609 -> [w1686]
                tunnel: [w1685] -> w1604
                tunnel: w1608 -> [w1685]
                tunnel: [w1684] -> w1603
                tunnel: w1607 -> [w1684]
                tunnel: [w1683] -> w1602
                tunnel: w1606 -> [w1683]
                tunnel: w1595 -> [w1682]
                tunnel: [w1682] -> w1594
                tunnel: w1581 -> [w1681]
                tunnel: [w1680] -> w1579
                tunnel: w1578 -> [w1680]
                tunnel: [w1679] -> w1569
                tunnel: w1568 -> [w1679]
                tunnel: w1605 -> [w1698]
                tunnel: w1604 -> [w1697]
                tunnel: w1603 -> [w1696]
                tunnel: w1602 -> [w1695]
                tunnel: w1592 -> [w1694]
                tunnel: [w1693] -> w1611
                tunnel: [w1692] -> w1610
                tunnel: w1594 -> [w1691]
                tunnel: [w1690] -> w1580
                tunnel: w1579 -> [w1689]
                tunnel: [w1688] -> w1567
                tunnel: w1569 -> [w1688]
                frame #0 {
                  n1008 = local read "Mean force (pN)"() -> (w1622:dbl)
                  n1009 = local read "Cutoff force (pN)"() -> (w1621:dbl)
                  n1010 = Less Or Equal?(x=w1622, y=w1621) -> (x <= y?=w1619:bool)
                  n1011 = And(x="Fish", y=w1619) -> (x .and. y?=w1620:bool)
                  n1012 = case shown="True" w1620 {
                    selector: w1620 -> [w1636 _]
                    tunnel: w1633 -> [w1639 w1656]
                    tunnel: w1632 -> [_ w1655]
                    tunnel: w1631 -> [w1641 w1654]
                    tunnel: w1630 -> [w1640 w1653]
                    tunnel: w1629 -> [w1638 w1652]
                    tunnel: w1628 -> [w1637 w1651]
                    tunnel: [w1641 w1650] -> w1627
                    tunnel: [w1640 w1649] -> w1626
                    tunnel: [w1639 w1648] -> w1625
                    tunnel: [w1637 w1647] -> w1615
                    tunnel: [w1638 w1646] -> w1624
                    tunnel: w1623 -> [_ w1645]
                    tunnel: [w1636 w1644] -> w1617
                    tunnel: [FALSE w1643] -> w1616
                    tunnel: [FALSE w1642] -> w1614
                    frame False {
                    }
                    frame True {
                      n1013 = while {
                        tunnel: w1656 -> [w1668]
                        tunnel: w1655 -> [w1667]
                        tunnel: w1654 -> [w1675]
                        tunnel: w1653 -> [w1674]
                        tunnel: w1652 -> [w1666]
                        tunnel: w1651 -> [w1672]
                        tunnel: [w1670] -> w1650
                        tunnel: [w1669] -> w1649
                        tunnel: [w1668] -> w1648
                        tunnel: [w1667] -> w1647
                        tunnel: [w1666] -> w1646
                        tunnel: w1645 -> [w1665]
                        tunnel: [w1658] -> w1644
                        tunnel: [w1658] -> w1643
                        tunnel: [w1657] -> w1642
                        i -> [w1664]
                        stop <- w1661 stop-if-true
                        # "top: x"
                        # "x direction"
                        # "y direction"
                        n1014 = Multiply(x=w1666, y=w1664) -> (x*y=w1673:dbl)
                        n1015 = local read "Cutoff force (pN)"() -> (w1659:dbl)
                        n1016 = local read "Mean force (pN)"() -> (w1660:dbl)
                        n1017 = Subtract(x=w1672, y=w1673) -> (x-y=w1671:dbl)
                        n1018 = Build Array(w1667, w1671) -> (w1678:dbl[])
                        n1019 = Build Array(w1671, w1667) -> (w1677:dbl[])
                        n1020 = Greater Or Equal?(x=w1664, y=w1665) -> (x >= y?=w1658:bool)
                        n1021 = Select(t=w1678, s=w1668, f=w1677) -> (s? t:f=w1676:dbl[])
                        n1022 = Greater?(x=w1660, y=w1659) -> (0:w1657:bool)
                        n1023 = local read "Fish"() -> (w1662:bool)
                        n1024 = Not(x=w1662) -> (.not. x?=w1663:bool)
                        n1025 = call-poly <vilib>:"DAQmx Write.vi"("task/channels in"=w1675, "data"=w1676, "error in"=w1674) -> ("task out"=w1670:refnum<k21>, "error out"=w1669:errorcluster)  [unwired: 10 in, 1 out]
                        n1026 = Compound Arithmetic op=OR(w1658, w1663, w1657) -> (w1661:bool)
                      }
                    }
                  }
                }
                frame #1 {
                  n1027 = case shown="True" w1681 {
                    frame False {
                    }
                    frame True {
                      n1028 = Wait (ms)(milliseconds to wait="Wait (ms)") -> ()  [unwired: 1 out]
                    }
                  }
                }
                frame #2 {
                  n1029 = case shown="True" w1691 {
                    tunnel: w1698 -> [w1701 w1710]
                    tunnel: w1697 -> [w1700 w1709]
                    tunnel: w1696 -> [_ w1708]
                    tunnel: w1695 -> [_ w1707]
                    tunnel: w1694 -> [_ w1706]
                    tunnel: [w1701 w1705] -> w1693
                    tunnel: [w1700 w1704] -> w1692
                    tunnel: [FALSE w1703] -> w1690
                    tunnel: w1689 -> [_ w1702]
                    frame False {
                    }
                    frame True {
                      n1030 = while {
                        tunnel: w1710 -> [w1742]
                        tunnel: w1709 -> [w1741]
                        tunnel: w1708 -> [w1713]
                        tunnel: w1707 -> [w1739]
                        tunnel: w1706 -> [w1738]
                        tunnel: [w1736] -> w1705
                        tunnel: [w1735] -> w1704
                        tunnel: [w1720] -> w1703
                        tunnel: w1702 -> [w1711]
                        i -> [w1727]
                        stop <- w1732 stop-if-true
                        # "y direction"
                        # "If tether formed,\nimmediately change\nto new delta."
                        n1031 = local read "Conv Y (nm/V)"() -> (w1714:dbl)
                        n1032 = local read "Conv X (nm/V)"() -> (w1712:dbl)
                        n1033 = local read "Fixed Y"() -> (w1721:dbl)
                        n1034 = local read "Fixed X"() -> (w1726:dbl)
                        n1035 = Select(t=w1714, s=w1713, f=w1712) -> (s? t:f=w1715:dbl)
                        n1036 = local read "Cutoff force (pN)"() -> (w1728:dbl)
                        n1037 = Divide(x="Delta after tether", y=w1715) -> (x/y=w1716:dbl)
                        n1038 = Multiply(x=w1739, y=w1727) -> (x*y=w1740:dbl)
                        n1039 = local read "Mean force (pN)"() -> (w1729:dbl)
                        n1040 = Add(x=w1738, y=w1740) -> (x+y=w1723:dbl)
                        n1041 = Select(t=w1721, s=w1713, f=w1726) -> (s? t:f=w1725:dbl)
                        n1042 = Greater?(x=w1729, y=w1728) -> (0:w1720:bool)
                        n1043 = Add(x=w1725, y=w1716) -> (x+y=w1724:dbl)
                        n1044 = Select(t=w1724, s=w1720, f=w1723) -> (s? t:f=w1722:dbl)
                        n1045 = local read "Fish Speed (ms)"() -> (w1734:i32)
                        n1046 = Build Array(w1711, w1722) -> (w1737:dbl[])
                        n1047 = Build Array(w1722, w1711) -> (w1718:dbl[])
                        n1048 = Select(t=w1737, s=w1713, f=w1718) -> (s? t:f=w1717:dbl[])
                        n1049 = case shown="True" w1720 {
                          tunnel: w1716 -> [_ _]
                          tunnel: w1717 -> [_ w1744]
                          frame False {
                          }
                          frame True {
                            n1050 = Array To Cluster(array=w1744) -> (cluster=w1743:cluster{"[0]":dbl, "[1]":dbl})
                            n1051 = property on="Trap position (V)" class="Clust (strict)"("Val(Sgnl)"=w1743) -> ()  [unwired: 2 in, 2 out]
                          }
                        }
                        n1052 = local read "Fish"() -> (w1731:bool)
                        n1053 = Greater Or Equal?(x=w1727, y=w1734) -> (x >= y?=w1733:bool)
                        n1054 = Not(x=w1731) -> (.not. x?=w1730:bool)
                        n1055 = call-poly <vilib>:"DAQmx Write.vi"("task/channels in"=w1742, "data"=w1717, "error in"=w1741) -> ("task out"=w1736:refnum<k21>, "error out"=w1735:errorcluster)  [unwired: 10 in, 1 out]
                        n1056 = Compound Arithmetic op=OR(w1733, w1730, w1720) -> (w1732:bool)
                      }
                    }
                  }
                }
              }
              n1057 = Add(x=w1585, y=w1573) -> (x+y=w1592:dbl)
              n1058 = Decrement(x="# attempts") -> (x-1=w1600:dbl)
              n1059 = Greater Or Equal?(x=w1596, y=w1600) -> (x >= y?=w1599:bool)
              n1060 = local read "Mean force (pN)"() -> (w1598:dbl)
              n1061 = Greater?(x=w1598, y="Cutoff force (pN)") -> (0:w1593:bool)
              n1062 = Compound Arithmetic op=OR(w1567, w1580, w1593, w1599) -> (w1571:bool)
              n1063 = Or(x=w1580, y=w1567) -> (x .or. y?=w1570:bool)
              "Tether" <- w1570
              n1064 = case shown="True" w1570 {
                frame False {
                }
                frame True {
                  n1065 = call <vilib>:"Beep.vi"() -> ()  [unwired: 12 in]
                }
              }
              n1066 = node-c288() -> ()  [unwired: 1 in, 1 out]
              "Attempt #" <- w1596
            }
            n1067 = node-c288(w1544) -> ()  [unwired: 1 out]
            n1068 = flat-sequence {
              tunnel: w1534 -> [w1553]
              tunnel: [w1553] -> w1533
              tunnel: w1532 -> [w1550]
              tunnel: w1531 -> [w1549]
              tunnel: w1530 -> [w1546]
              tunnel: w1533 -> [w1555]
              frame #0 {
                w1552 = T19 1 items=["no dialog", "OK message", "continue or stop message", "OK message + warnings", "continue/stop + warnings"] ("type of dialog (OK msg:1)")
                n1069 = call <vilib>:"DAQmx Clear Task.vi"("task in"=w1550, "error in"=w1549) -> ("error out"=w1551:errorcluster)  [unwired: 13 in]
                n1070 = Not(x=w1546) -> (.not. x?=w1547:bool)
                n1071 = local write "Fish"(w1547) -> ()
                n1072 = Wait (ms)(milliseconds to wait=u32 300) -> ()  [unwired: 1 out]
                n1073 = call <vilib>:"Simple Error Handler.vi"("type of dialog (OK msg:1)"=w1552, "error in (no error)"=w1551) -> ()  [unwired: 3 in, 5 out]
              }
              frame #1 {
                n1074 = And(x=w1555, y="Raster after\n tether?") -> (x .and. y?=w1556:bool)
                n1075 = case shown="True" w1556 {
                  selector: w1556 -> [_ w1557]
                  frame False {
                  }
                  frame True {
                    n1076 = stacked-sequence {
                      tunnel: w1557 -> [_ _ _ _ w1566]
                      frame #0 {
                        n1077 = local read "Raster set"() -> (w1561:i32)
                        n1078 = property on="Inject Sample" class="Bool (strict)"("Val(Sgnl)"=FALSE ("Value (Signaling)")) -> ()  [unwired: 2 in, 2 out]
                        n1079 = Replace Array Subset(array=i32[] [0], new element=w1561, index=0) -> (w1558:i32[])
                        n1080 = property on="Scan Parameters" class="Arr (strict)"("Index Values"=w1558) -> ()  [unwired: 2 in, 2 out]
                      }
                      frame #1 {
                        n1081 = Wait (ms)(milliseconds to wait=u32 500) -> ()  [unwired: 1 out]
                      }
                      frame #2 {
                        n1082 = property on="Load param" class="Bool (strict)"("Val(Sgnl)"=TRUE ("Value (Signaling)")) -> ()  [unwired: 2 in, 2 out]
                      }
                      frame #3 {
                        n1083 = Wait (ms)(milliseconds to wait=u32 500) -> ()  [unwired: 1 out]
                      }
                      frame #4 {
                        n1084 = property on="Raster scan" class="Bool (strict)"("Val(Sgnl)"=w1566) -> ()  [unwired: 2 in, 2 out]
                      }
                    }
                  }
                }
              }
            }
          }
        }
      }
      event "Load param": Value Change {
        n1085 = event-data() -> ()  [unwired: 1 in, 6 out]
        n1086 = property on="Scan Parameters" class="Arr (strict)"() -> ("Index Values"=w1760:u32[])  [unwired: 2 in, 2 out]
        n1087 = Index Array(array=w1760, index=0) -> (element=w1757:u32)
        n1088 = Index Array(array="Scan Parameters", index=w1757) -> (element=w1756:T22)
        n1089 = Unbundle(w1756) -> ("Scan range 1"=w1754:dbl, "Step size 1"=w1753:dbl, "Scan speed 1"=w1751:i32, "# scans 2"=w1752:i32)  [unwired: 1 out]
        n1090 = property on="Scan speed 1" class="DigNum (strict)"("Val(Sgnl)"=w1751) -> ()  [unwired: 2 in, 2 out]
        n1091 = property on="# scans" class="DigNum (strict)"("Val(Sgnl)"=w1752) -> ()  [unwired: 2 in, 2 out]
        n1092 = property on="Scan range (nm)" class="DigNum (strict)"("Val(Sgnl)"=w1754) -> ()  [unwired: 2 in, 2 out]
        n1093 = property on="Step size 1" class="DigNum (strict)"("Val(Sgnl)"=w1753) -> ()  [unwired: 2 in, 2 out]
        n1094 = local write "Load param"(FALSE ("Load param")) -> ()
      }
      event "# scans", "Scan range (nm)", "Step size (nm)", "Scan speed (nm/s)": Value Change {
        n1095 = event-data() -> ()  [unwired: 1 in, 6 out]
        n1096 = local read "Pulling direction"() -> (w1791:bool)
        n1097 = Reciprocal(x="Scan speed (nm/s)") -> (1/x=w1783:dbl)
        n1098 = local read "Conv Y (nm/V)"() -> (w1789:dbl)
        n1099 = local read "Conv X (nm/V)"() -> (w1790:dbl)
        n1100 = Multiply(x="Step size (nm)", y=w1783) -> (x*y=w1781:dbl)
        n1101 = Divide(x="Scan range (nm)", y="Step size (nm)") -> (x/y=w1788:dbl)
        n1102 = Absolute Value(x=w1788) -> (abs(x)=w1787:dbl)
        n1103 = Multiply(x=w1781, y=1000.0) -> (x*y=w1768:dbl)
        n1104 = Select(t=w1789, s=w1791, f=w1790) -> (s? t:f=w1779:dbl)
        n1105 = Multiply(x="# scans", y=2) -> (x*y=w1767:i32)
        n1106 = To Unsigned Quad Integer(1:w1787) -> (0:w1777:u64)
        "Scan steps (mirror)" <- w1777
        n1107 = Divide(x="Scan range (nm)", y=w1779) -> (x/y=→"Scan range (V)":dbl)
        n1108 = Multiply(x=w1777, y=w1768) -> (x*y=w1776:dbl)
        n1109 = Divide(x="Step size (nm)", y=w1779) -> (x/y=→"Scan increment (V)":dbl)
        n1110 = Round Toward +Infinity(x=w1768) -> (ceil(x): smallest int >= x=w1765:dbl)
        "Time per step (ms)" <- w1765
        n1111 = local read "Data update period (s/set)"() -> (w1771:dbl)
        n1112 = Multiply(x=w1767, y=w1776) -> (x*y=w1774:dbl)
        n1113 = Divide(x=w1774, y=1000.0) -> (x/y=w1772:dbl)
        "Total raster time (s)" <- w1772
        n1114 = local read "Data update period (s/set)"() -> (w1763:dbl)
        n1115 = Divide(x=w1772, y=w1771) -> (x/y=w1770:dbl)
        n1116 = Round Toward -Infinity(1:w1770) -> (0:→"N sets to be saved":dbl)
        n1117 = Multiply(x=w1763, y=1000.0) -> (x*y=w1761:dbl)
        n1118 = Less?(x=w1765, y=w1761) -> (x < y?=w1764:bool)
        n1119 = case shown="True" w1764 {
          selector: w1764 -> [_ w1792]
          frame False {
          }
          frame True {
            n1120 = call "Display Message to User"("Enable"=w1792) -> ()  [unwired: 9 in, 2 out]
          }
        }
      }
      event "Pulling direction": Value Change {
        n1121 = event-data() -> ()  [unwired: 1 in, 6 out]
        n1122 = local read "Pulling direction"() -> (w1798:bool)
        n1123 = local read "Conv Y (nm/V)"() -> (w1800:dbl)
        n1124 = local read "Conv X (nm/V)"() -> (w1799:dbl)
        n1125 = local read "Scan range (nm)"() -> (w1797:dbl)
        n1126 = Select(t=w1800, s=w1798, f=w1799) -> (s? t:f=w1794:dbl)
        n1127 = local read "Step size (nm)"() -> (w1795:dbl)
        n1128 = case shown="False" w1798 {
          frame False {
            n1129 = local read "Fixed Y"() -> (w1803:dbl)
            n1130 = local read "Trap delta (nm)"() -> (w1808:dbl)
            n1131 = local read "Conv X (nm/V)"() -> (w1807:dbl)
            n1132 = local read "Fixed X"() -> (w1805:dbl)
            n1133 = Divide(x=w1808, y=w1807) -> (x/y=w1806:dbl)
            n1134 = Add(x=w1806, y=w1805) -> (x+y=w1804:dbl)
            n1135 = Build Array(w1804, w1803) -> (w1802:dbl[])
            n1136 = Array To Cluster(array=w1802) -> (cluster=w1801:cluster{"[0]":dbl, "[1]":dbl})
            n1137 = property on="Trap position (V)" class="Clust (strict)"("Val(Sgnl)"=w1801) -> ()  [unwired: 2 in, 2 out]
          }
          frame True {
            n1138 = local read "Trap delta (nm)"() -> (w1816:dbl)
            n1139 = local read "Conv Y (nm/V)"() -> (w1815:dbl)
            n1140 = local read "Fixed X"() -> (w1811:dbl)
            n1141 = local read "Fixed Y"() -> (w1813:dbl)
            n1142 = Divide(x=w1816, y=w1815) -> (x/y=w1814:dbl)
            n1143 = Add(x=w1814, y=w1813) -> (x+y=w1812:dbl)
            n1144 = Build Array(w1811, w1812) -> (w1810:dbl[])
            n1145 = Array To Cluster(array=w1810) -> (cluster=w1809:cluster{"[0]":dbl, "[1]":dbl})
            n1146 = property on="Trap position (V)" class="Clust (strict)"("Val(Sgnl)"=w1809) -> ()  [unwired: 2 in, 2 out]
          }
        }
        n1147 = Divide(x=w1797, y=w1794) -> (x/y=w1796:dbl)
        n1148 = Divide(x=w1795, y=w1794) -> (x/y=w1793:dbl)
        n1149 = local write "Scan range (V)"(w1796) -> ()
        n1150 = local write "Scan increment (V)"(w1793) -> ()
      }
      event "Averaging Number": Value Change {
        n1151 = event-data() -> ()  [unwired: 1 in, 6 out]
        n1152 = local read "# Samples/channel (in)"() -> (w1820:i32)
        n1153 = local read "Averaging Number"() -> (w1818:i32)
        n1154 = Quotient & Remainder(x=w1820, y=w1818) -> (floor(x/y)=w1819:i32)  [unwired: 1 out]
        n1155 = Multiply(x=w1819, y=w1818) -> (x*y=w1817:i32)
        n1156 = local write "# Samples/channel (in)"(w1817) -> ()
      }
    }
    n1157 = node-c288() -> ()  [unwired: 1 in, 1 out]
  }
  n1158 = call <vilib>:"Simple Error Handler.vi"("error in (no error)"=w95) -> ()  [unwired: 4 in, 5 out]
  n1159 = disable-structure shown="Enabled" {
    frame Disabled {
      n1160 = node-c288(2 ("Processor")) -> (w1826:T11)  [unwired: 3 in]
      n1161 = timed-loop "Pump Control" {
        timing: w1826 -> [_]
        timing-out: [_] -> w1825
        tunnel: refnum<visa-resource-name> "COM6" ("VISA resource name") -> [w1828]
        stop <- w1827 stop-if-true
        n1162 = node-c288() -> ()  [unwired: 1 in, 1 out]
        n1163 = event shown="[4] \"Inject Pump 1\": Value Change" {
          selector: _ -> [_ _ _ _ _ _ _ _ _]
          dyn-events: _ -> [_ _ _ _ _ _ _ _ _]
          timeout: _ -> [_ _ _ _ _ _ _ _ _]
          tunnel: w1828 -> [w1836 w1932 _ w2008 w2136 w2279 w2324 w2382 w2441]
          tunnel: [_ _ w2007 _ _ _ _ _ _] -> w1827
          event "Flush Pump 1": Value Change {
            w1837 = "\r"
            n1164 = event-data() -> ()  [unwired: 1 in, 5 out]
            n1165 = call-poly "VISA Configure Serial Port"("VISA resource name"=w1836) -> ("VISA resource name out"=w1850:refnum<visa-resource-name>, "error out"=w1851:errorcluster)  [unwired: 13 in]
            n1166 = local read "Write Wait"() -> (w1829:i32)
            n1167 = Concatenate Strings("enter pump1", w1837) -> (w1838:string)
            n1168 = flat-sequence {
              tunnel: w1851 -> [w1870]
              tunnel: w1850 -> [w1872]
              tunnel: [w1871] -> w1867
              tunnel: [w1869] -> w1866
              tunnel: w1838 -> [w1868]
              tunnel: w1867 -> [w1875]
              tunnel: [w1875] -> w1865
              tunnel: w1866 -> [w1874]
              tunnel: [w1874] -> w1864
              tunnel: w1829 -> [w1873]
              tunnel: [w1880] -> w1863
              tunnel: w1843 -> [w1879]
              tunnel: [w1876] -> w1862
              tunnel: w1865 -> [w1878]
              tunnel: w1864 -> [w1877]
              tunnel: w1863 -> [w1883]
              tunnel: [w1883] -> w1861
              tunnel: [w1882] -> w1860
              tunnel: w1862 -> [w1882]
              tunnel: w1829 -> [w1881]
              tunnel: w1861 -> [w1888]
              tunnel: [w1887] -> w1859
              tunnel: w1846 -> [w1886]
              tunnel: w1860 -> [w1885]
              tunnel: [w1884] -> w1858
              tunnel: w1859 -> [w1891]
              tunnel: [w1891] -> w1857
              tunnel: [w1890] -> w1856
              tunnel: w1858 -> [w1890]
              tunnel: w1829 -> [w1889]
              tunnel: w1857 -> [w1896]
              tunnel: [w1895] -> w1855
              tunnel: w1849 -> [w1894]
              tunnel: w1856 -> [w1893]
              tunnel: [w1892] -> w1854
              tunnel: [w1899] -> w1853
              tunnel: w1855 -> [w1899]
              tunnel: [w1898] -> w1852
              tunnel: w1854 -> [w1898]
              tunnel: w1829 -> [w1897]
              tunnel: w1853 -> [w1904]
              tunnel: w1852 -> [w1901]
              tunnel: [w1903] -> w1832
              tunnel: [w1902] -> w1830
              tunnel: [w1909] -> w1833
              tunnel: w1832 -> [w1909]
              tunnel: [w1908] -> w1831
              tunnel: w1830 -> [w1908]
              tunnel: w1829 -> [w1907]
              tunnel: w1833 -> [w1911]
              tunnel: w1831 -> [w1910]
              frame #0 {
                n1169 = VISA Write(VISA resource name=w1872, write buffer=w1868, error in (no error)=w1870) -> (VISA resource name out=w1871:refnum<visa-resource-name>, error out=w1869:errorcluster)  [unwired: 1 out]
              }
              frame #1 {
                n1170 = Wait (ms)(milliseconds to wait=w1873) -> ()  [unwired: 1 out]
              }
              frame #2 {
                n1171 = VISA Write(VISA resource name=w1878, write buffer=w1879, error in (no error)=w1877) -> (VISA resource name out=w1880:refnum<visa-resource-name>, error out=w1876:errorcluster)  [unwired: 1 out]
              }
              frame #3 {
                n1172 = Wait (ms)(milliseconds to wait=w1881) -> ()  [unwired: 1 out]
              }
              frame #4 {
                n1173 = VISA Write(VISA resource name=w1888, write buffer=w1886, error in (no error)=w1885) -> (VISA resource name out=w1887:refnum<visa-resource-name>, error out=w1884:errorcluster)  [unwired: 1 out]
              }
              frame #5 {
                n1174 = Wait (ms)(milliseconds to wait=w1889) -> ()  [unwired: 1 out]
              }
              frame #6 {
                n1175 = VISA Write(VISA resource name=w1896, write buffer=w1894, error in (no error)=w1893) -> (VISA resource name out=w1895:refnum<visa-resource-name>, error out=w1892:errorcluster)  [unwired: 1 out]
              }
              frame #7 {
                n1176 = Wait (ms)(milliseconds to wait=w1897) -> ()  [unwired: 1 out]
              }
              frame #8 {
                n1177 = Concatenate Strings("start ", "\r") -> (w1900:string)
                n1178 = VISA Write(VISA resource name=w1904, write buffer=w1900, error in (no error)=w1901) -> (VISA resource name out=w1903:refnum<visa-resource-name>, error out=w1902:errorcluster)  [unwired: 1 out]
              }
              frame #9 {
                n1179 = Wait (ms)(milliseconds to wait=w1907) -> ()  [unwired: 1 out]
              }
              frame #10 {
                n1180 = local write "Flush Pump 1"(FALSE ("Flush Pump 1")) -> ()
                n1181 = Concatenate Strings("enter main ", "\r") -> (w1915:string)
                n1182 = VISA Write(VISA resource name=w1911, write buffer=w1915, error in (no error)=w1910) -> (VISA resource name out=w1914:refnum<visa-resource-name>, error out=w1913:errorcluster)  [unwired: 1 out]
                n1183 = VISA Close(VISA resource name=w1914, error in (no error)=w1913) -> ()  [unwired: 1 out]
              }
            }
            n1184 = Concatenate Strings("set units 4 ", w1837) -> (w1843:string)
            n1185 = Multiply(x="Flush\nRate (ul/min)", y=60) -> (x*y=w1841:dbl)
            n1186 = Number To Decimal String(number=w1841) -> (decimal integer string=w1844:string)  [unwired: 1 in]
            n1187 = Concatenate Strings("set rate ", w1844, w1837) -> (w1846:string)
            n1188 = Number To Decimal String(number="Flush\nVolume (ul)") -> (decimal integer string=w1848:string)  [unwired: 1 in]
            n1189 = Concatenate Strings("set volume ", w1848, w1837) -> (w1849:string)
          }
          event "Flush Pump 2": Value Change {
            w1923 = "\r"
            n1190 = event-data() -> ()  [unwired: 1 in, 5 out]
            n1191 = call-poly "VISA Configure Serial Port"("VISA resource name"=w1932) -> ("VISA resource name out"=w1943:refnum<visa-resource-name>, "error out"=w1944:errorcluster)  [unwired: 13 in]
            n1192 = local read "Write Wait"() -> (w1918:i32)
            n1193 = Concatenate Strings("enter pump2", w1923) -> (w1924:string)
            n1194 = flat-sequence {
              tunnel: w1944 -> [w1959]
              tunnel: w1943 -> [w1961]
              tunnel: [w1960] -> w1929
              tunnel: [w1958] -> w1927
              tunnel: w1924 -> [w1957]
              tunnel: w1929 -> [w1964]
              tunnel: [w1964] -> w1928
              tunnel: w1927 -> [w1963]
              tunnel: [w1963] -> w1926
              tunnel: w1918 -> [w1962]
              tunnel: [w1969] -> w1956
              tunnel: w1936 -> [w1968]
              tunnel: [w1965] -> w1955
              tunnel: w1928 -> [w1967]
              tunnel: w1926 -> [w1966]
              tunnel: w1956 -> [w1972]
              tunnel: [w1972] -> w1954
              tunnel: [w1971] -> w1953
              tunnel: w1955 -> [w1971]
              tunnel: w1918 -> [w1970]
              tunnel: w1954 -> [w1977]
              tunnel: [w1976] -> w1952
              tunnel: w1939 -> [w1975]
              tunnel: w1953 -> [w1974]
              tunnel: [w1973] -> w1951
              tunnel: w1952 -> [w1980]
              tunnel: [w1980] -> w1950
              tunnel: [w1979] -> w1949
              tunnel: w1951 -> [w1979]
              tunnel: w1918 -> [w1978]
              tunnel: w1950 -> [w1985]
              tunnel: [w1984] -> w1948
              tunnel: w1942 -> [w1983]
              tunnel: w1949 -> [w1982]
              tunnel: [w1981] -> w1947
              tunnel: [w1988] -> w1946
              tunnel: w1948 -> [w1988]
              tunnel: [w1987] -> w1945
              tunnel: w1947 -> [w1987]
              tunnel: w1918 -> [w1986]
              tunnel: w1946 -> [w1995]
              tunnel: w1945 -> [w1994]
              tunnel: [w1990] -> w1922
              tunnel: [w1989] -> w1920
              tunnel: w1922 -> [w1998]
              tunnel: [w1998] -> w1921
              tunnel: w1920 -> [w1997]
              tunnel: [w1997] -> w1919
              tunnel: w1918 -> [w1996]
              tunnel: w1921 -> [w2002]
              tunnel: w1919 -> [w2001]
              frame #0 {
                n1195 = VISA Write(VISA resource name=w1961, write buffer=w1957, error in (no error)=w1959) -> (VISA resource name out=w1960:refnum<visa-resource-name>, error out=w1958:errorcluster)  [unwired: 1 out]
              }
              frame #1 {
                n1196 = Wait (ms)(milliseconds to wait=w1962) -> ()  [unwired: 1 out]
              }
              frame #2 {
                n1197 = VISA Write(VISA resource name=w1967, write buffer=w1968, error in (no error)=w1966) -> (VISA resource name out=w1969:refnum<visa-resource-name>, error out=w1965:errorcluster)  [unwired: 1 out]
              }
              frame #3 {
                n1198 = Wait (ms)(milliseconds to wait=w1970) -> ()  [unwired: 1 out]
              }
              frame #4 {
                n1199 = VISA Write(VISA resource name=w1977, write buffer=w1975, error in (no error)=w1974) -> (VISA resource name out=w1976:refnum<visa-resource-name>, error out=w1973:errorcluster)  [unwired: 1 out]
              }
              frame #5 {
                n1200 = Wait (ms)(milliseconds to wait=w1978) -> ()  [unwired: 1 out]
              }
              frame #6 {
                n1201 = VISA Write(VISA resource name=w1985, write buffer=w1983, error in (no error)=w1982) -> (VISA resource name out=w1984:refnum<visa-resource-name>, error out=w1981:errorcluster)  [unwired: 1 out]
              }
              frame #7 {
                n1202 = Wait (ms)(milliseconds to wait=w1986) -> ()  [unwired: 1 out]
              }
              frame #8 {
                n1203 = Concatenate Strings("start ", "\r") -> (w1993:string)
                n1204 = VISA Write(VISA resource name=w1995, write buffer=w1993, error in (no error)=w1994) -> (VISA resource name out=w1990:refnum<visa-resource-name>, error out=w1989:errorcluster)  [unwired: 1 out]
              }
              frame #9 {
                n1205 = Wait (ms)(milliseconds to wait=w1996) -> ()  [unwired: 1 out]
              }
              frame #10 {
                n1206 = local write "Flush Pump 2"(FALSE ("Flush Pump 1")) -> ()
                n1207 = Concatenate Strings("enter main ", "\r") -> (w2003:string)
                n1208 = VISA Write(VISA resource name=w2002, write buffer=w2003, error in (no error)=w2001) -> (VISA resource name out=w2000:refnum<visa-resource-name>, error out=w1999:errorcluster)  [unwired: 1 out]
                n1209 = VISA Close(VISA resource name=w2000, error in (no error)=w1999) -> ()  [unwired: 1 out]
              }
            }
            n1210 = Concatenate Strings("set units 4 ", w1923) -> (w1936:string)
            n1211 = Multiply(x="Flush \nRate (ul/min)  2", y=60) -> (x*y=w1934:dbl)
            n1212 = Number To Decimal String(number=w1934) -> (decimal integer string=w1937:string)  [unwired: 1 in]
            n1213 = Concatenate Strings("set rate ", w1937, w1923) -> (w1939:string)
            n1214 = Number To Decimal String(number="Flush\nVolume (ul)  2") -> (decimal integer string=w1941:string)  [unwired: 1 in]
            n1215 = Concatenate Strings("set volume ", w1941, w1923) -> (w1942:string)
          }
          event "Stop": Value Change {
            n1216 = event-data() -> ()  [unwired: 1 in, 5 out]
            n1217 = local read "Stop"() -> (w2007:bool)
          }
          event "Inject Pump 2": Value Change {
            n1218 = event-data() -> ()  [unwired: 1 in, 5 out]
            n1219 = case shown="True" "Inject Pump 2" {
              tunnel: w2008 -> [w2011 w2053]
              frame False {
                n1220 = local read "Write Wait"() -> (w2010:i32)
                n1221 = call-poly "VISA Configure Serial Port"("VISA resource name"=w2011) -> ("VISA resource name out"=w2015:refnum<visa-resource-name>, "error out"=w2016:errorcluster)  [unwired: 13 in]
                n1222 = Concatenate Strings("enter pump2", "\r") -> (w2013:string)
                n1223 = flat-sequence {
                  tunnel: w2016 -> [w2027]
                  tunnel: w2015 -> [w2029]
                  tunnel: [w2028] -> w2024
                  tunnel: [w2026] -> w2023
                  tunnel: w2013 -> [w2025]
                  tunnel: w2024 -> [w2032]
                  tunnel: w2023 -> [w2031]
                  tunnel: [w2032] -> w2022
                  tunnel: [w2031] -> w2021
                  tunnel: w2010 -> [w2030]
                  tunnel: [w2036] -> w2020
                  tunnel: [w2035] -> w2019
                  tunnel: w2022 -> [w2034]
                  tunnel: w2021 -> [w2033]
                  tunnel: w2020 -> [w2042]
                  tunnel: [w2042] -> w2018
                  tunnel: w2019 -> [w2041]
                  tunnel: [w2041] -> w2017
                  tunnel: w2010 -> [w2040]
                  tunnel: w2018 -> [w2046]
                  tunnel: w2017 -> [w2045]
                  frame #0 {
                    n1224 = VISA Write(VISA resource name=w2029, write buffer=w2025, error in (no error)=w2027) -> (VISA resource name out=w2028:refnum<visa-resource-name>, error out=w2026:errorcluster)  [unwired: 1 out]
                  }
                  frame #1 {
                    n1225 = Wait (ms)(milliseconds to wait=w2030) -> ()  [unwired: 1 out]
                  }
                  frame #2 {
                    n1226 = Concatenate Strings("stop ", "\r") -> (w2039:string)
                    n1227 = VISA Write(VISA resource name=w2034, write buffer=w2039, error in (no error)=w2033) -> (VISA resource name out=w2036:refnum<visa-resource-name>, error out=w2035:errorcluster)  [unwired: 1 out]
                  }
                  frame #3 {
                    n1228 = Wait (ms)(milliseconds to wait=w2040) -> ()  [unwired: 1 out]
                  }
                  frame #4 {
                    n1229 = Concatenate Strings("enter main ", "\r") -> (w2047:string)
                    n1230 = VISA Write(VISA resource name=w2046, write buffer=w2047, error in (no error)=w2045) -> (VISA resource name out=w2044:refnum<visa-resource-name>, error out=w2043:errorcluster)  [unwired: 1 out]
                    n1231 = VISA Close(VISA resource name=w2044, error in (no error)=w2043) -> ()  [unwired: 1 out]
                  }
                }
              }
              frame True {
                w2066 = "\r"
                n1232 = call-poly "VISA Configure Serial Port"("VISA resource name"=w2053) -> ("VISA resource name out"=w2055:refnum<visa-resource-name>, "error out"=w2054:errorcluster)  [unwired: 13 in]
                n1233 = local read "Write Wait"() -> (w2050:i32)
                n1234 = Concatenate Strings("enter pump2", w2066) -> (w2065:string)
                n1235 = flat-sequence {
                  tunnel: w2054 -> [w2089]
                  tunnel: w2055 -> [w2091]
                  tunnel: [w2090] -> w2086
                  tunnel: [w2088] -> w2085
                  tunnel: w2065 -> [w2087]
                  tunnel: w2086 -> [w2094]
                  tunnel: [w2094] -> w2084
                  tunnel: w2085 -> [w2093]
                  tunnel: [w2093] -> w2083
                  tunnel: w2050 -> [w2092]
                  tunnel: [w2099] -> w2082
                  tunnel: w2062 -> [w2098]
                  tunnel: [w2095] -> w2081
                  tunnel: w2084 -> [w2097]
                  tunnel: w2083 -> [w2096]
                  tunnel: w2082 -> [w2102]
                  tunnel: [w2102] -> w2080
                  tunnel: [w2101] -> w2079
                  tunnel: w2081 -> [w2101]
                  tunnel: w2050 -> [w2100]
                  tunnel: w2080 -> [w2107]
                  tunnel: [w2106] -> w2078
                  tunnel: w2059 -> [w2105]
                  tunnel: w2079 -> [w2104]
                  tunnel: [w2103] -> w2077
                  tunnel: w2078 -> [w2110]
                  tunnel: [w2110] -> w2076
                  tunnel: [w2109] -> w2075
                  tunnel: w2077 -> [w2109]
                  tunnel: w2050 -> [w2108]
                  tunnel: w2076 -> [w2115]
                  tunnel: [w2114] -> w2074
                  tunnel: w2056 -> [w2113]
                  tunnel: w2075 -> [w2112]
                  tunnel: [w2111] -> w2073
                  tunnel: [w2118] -> w2072
                  tunnel: w2074 -> [w2118]
                  tunnel: [w2117] -> w2071
                  tunnel: w2073 -> [w2117]
                  tunnel: w2050 -> [w2116]
                  tunnel: w2072 -> [w2125]
                  tunnel: w2071 -> [w2124]
                  tunnel: [w2120] -> w2070
                  tunnel: [w2119] -> w2069
                  tunnel: w2070 -> [w2128]
                  tunnel: [w2128] -> w2068
                  tunnel: w2069 -> [w2127]
                  tunnel: [w2127] -> w2067
                  tunnel: w2050 -> [w2126]
                  tunnel: w2068 -> [w2132]
                  tunnel: w2067 -> [w2131]
                  frame #0 {
                    n1236 = VISA Write(VISA resource name=w2091, write buffer=w2087, error in (no error)=w2089) -> (VISA resource name out=w2090:refnum<visa-resource-name>, error out=w2088:errorcluster)  [unwired: 1 out]
                  }
                  frame #1 {
                    n1237 = Wait (ms)(milliseconds to wait=w2092) -> ()  [unwired: 1 out]
                  }
                  frame #2 {
                    n1238 = VISA Write(VISA resource name=w2097, write buffer=w2098, error in (no error)=w2096) -> (VISA resource name out=w2099:refnum<visa-resource-name>, error out=w2095:errorcluster)  [unwired: 1 out]
                  }
                  frame #3 {
                    n1239 = Wait (ms)(milliseconds to wait=w2100) -> ()  [unwired: 1 out]
                  }
                  frame #4 {
                    n1240 = VISA Write(VISA resource name=w2107, write buffer=w2105, error in (no error)=w2104) -> (VISA resource name out=w2106:refnum<visa-resource-name>, error out=w2103:errorcluster)  [unwired: 1 out]
                  }
                  frame #5 {
                    n1241 = Wait (ms)(milliseconds to wait=w2108) -> ()  [unwired: 1 out]
                  }
                  frame #6 {
                    n1242 = VISA Write(VISA resource name=w2115, write buffer=w2113, error in (no error)=w2112) -> (VISA resource name out=w2114:refnum<visa-resource-name>, error out=w2111:errorcluster)  [unwired: 1 out]
                  }
                  frame #7 {
                    n1243 = Wait (ms)(milliseconds to wait=w2116) -> ()  [unwired: 1 out]
                  }
                  frame #8 {
                    n1244 = Concatenate Strings("start ", "\r") -> (w2123:string)
                    n1245 = VISA Write(VISA resource name=w2125, write buffer=w2123, error in (no error)=w2124) -> (VISA resource name out=w2120:refnum<visa-resource-name>, error out=w2119:errorcluster)  [unwired: 1 out]
                  }
                  frame #9 {
                    n1246 = Wait (ms)(milliseconds to wait=w2126) -> ()  [unwired: 1 out]
                  }
                  frame #10 {
                    n1247 = Concatenate Strings("enter main ", "\r") -> (w2133:string)
                    n1248 = VISA Write(VISA resource name=w2132, write buffer=w2133, error in (no error)=w2131) -> (VISA resource name out=w2130:refnum<visa-resource-name>, error out=w2129:errorcluster)  [unwired: 1 out]
                    n1249 = VISA Close(VISA resource name=w2130, error in (no error)=w2129) -> ()  [unwired: 1 out]
                  }
                }
                n1250 = local read "Normal \nRate (ul/hr)  2"() -> (w2051:dbl)
                n1251 = Concatenate Strings("set units 4 ", w2066) -> (w2062:string)
                n1252 = local read "Normal \nVolume (ul) 2"() -> (w2052:dbl)
                n1253 = Number To Decimal String(number=w2051) -> (decimal integer string=w2061:string)  [unwired: 1 in]
                n1254 = Concatenate Strings("set rate ", w2061, w2066) -> (w2059:string)
                n1255 = Number To Decimal String(number=w2052) -> (decimal integer string=w2057:string)  [unwired: 1 in]
                n1256 = Concatenate Strings("set volume ", w2057, w2066) -> (w2056:string)
              }
            }
          }
          event "Inject Pump 1": Value Change {
            n1257 = event-data() -> ()  [unwired: 1 in, 5 out]
            n1258 = case shown="True" "Inject Pump 1" {
              tunnel: w2136 -> [w2139 w2181]
              frame False {
                n1259 = local read "Write Wait"() -> (w2138:i32)
                n1260 = call-poly "VISA Configure Serial Port"("VISA resource name"=w2139) -> ("VISA resource name out"=w2143:refnum<visa-resource-name>, "error out"=w2144:errorcluster)  [unwired: 13 in]
                n1261 = Concatenate Strings("enter pump1", "\r") -> (w2141:string)
                n1262 = flat-sequence {
                  tunnel: w2144 -> [w2155]
                  tunnel: w2143 -> [w2157]
                  tunnel: [w2156] -> w2152
                  tunnel: [w2154] -> w2151
                  tunnel: w2141 -> [w2153]
                  tunnel: w2152 -> [w2160]
                  tunnel: w2151 -> [w2159]
                  tunnel: [w2160] -> w2150
                  tunnel: [w2159] -> w2149
                  tunnel: w2138 -> [w2158]
                  tunnel: [w2164] -> w2148
                  tunnel: [w2163] -> w2147
                  tunnel: w2150 -> [w2162]
                  tunnel: w2149 -> [w2161]
                  tunnel: w2148 -> [w2170]
                  tunnel: [w2170] -> w2146
                  tunnel: w2147 -> [w2169]
                  tunnel: [w2169] -> w2145
                  tunnel: w2138 -> [w2168]
                  tunnel: w2146 -> [w2174]
                  tunnel: w2145 -> [w2173]
                  frame #0 {
                    n1263 = VISA Write(VISA resource name=w2157, write buffer=w2153, error in (no error)=w2155) -> (VISA resource name out=w2156:refnum<visa-resource-name>, error out=w2154:errorcluster)  [unwired: 1 out]
                  }
                  frame #1 {
                    n1264 = Wait (ms)(milliseconds to wait=w2158) -> ()  [unwired: 1 out]
                  }
                  frame #2 {
                    n1265 = Concatenate Strings("stop ", "\r") -> (w2167:string)
                    n1266 = VISA Write(VISA resource name=w2162, write buffer=w2167, error in (no error)=w2161) -> (VISA resource name out=w2164:refnum<visa-resource-name>, error out=w2163:errorcluster)  [unwired: 1 out]
                  }
                  frame #3 {
                    n1267 = Wait (ms)(milliseconds to wait=w2168) -> ()  [unwired: 1 out]
                  }
                  frame #4 {
                    n1268 = Concatenate Strings("enter main ", "\r") -> (w2175:string)
                    n1269 = VISA Write(VISA resource name=w2174, write buffer=w2175, error in (no error)=w2173) -> (VISA resource name out=w2172:refnum<visa-resource-name>, error out=w2171:errorcluster)  [unwired: 1 out]
                    n1270 = VISA Close(VISA resource name=w2172, error in (no error)=w2171) -> ()  [unwired: 1 out]
                  }
                }
              }
              frame True {
                w2194 = "\r"
                n1271 = call-poly "VISA Configure Serial Port"("VISA resource name"=w2181) -> ("VISA resource name out"=w2183:refnum<visa-resource-name>, "error out"=w2182:errorcluster)  [unwired: 13 in]
                n1272 = local read "Write Wait"() -> (w2178:i32)
                n1273 = flat-sequence {
                  tunnel: w2182 -> [w2217]
                  tunnel: w2183 -> [w2219]
                  tunnel: [w2218] -> w2214
                  tunnel: [w2216] -> w2213
                  tunnel: w2193 -> [w2215]
                  tunnel: w2214 -> [w2222]
                  tunnel: [w2222] -> w2212
                  tunnel: w2213 -> [w2221]
                  tunnel: [w2221] -> w2211
                  tunnel: w2178 -> [w2220]
                  tunnel: [w2227] -> w2210
                  tunnel: w2190 -> [w2226]
                  tunnel: [w2223] -> w2209
                  tunnel: w2212 -> [w2225]
                  tunnel: w2211 -> [w2224]
                  tunnel: w2210 -> [w2230]
                  tunnel: [w2230] -> w2208
                  tunnel: [w2229] -> w2207
                  tunnel: w2209 -> [w2229]
                  tunnel: w2178 -> [w2228]
                  tunnel: w2208 -> [w2235]
                  tunnel: [w2234] -> w2206
                  tunnel: w2187 -> [w2233]
                  tunnel: w2207 -> [w2232]
                  tunnel: [w2231] -> w2205
                  tunnel: w2206 -> [w2238]
                  tunnel: [w2238] -> w2204
                  tunnel: [w2237] -> w2203
                  tunnel: w2205 -> [w2237]
                  tunnel: w2178 -> [w2236]
                  tunnel: w2204 -> [w2243]
                  tunnel: [w2242] -> w2202
                  tunnel: w2184 -> [w2241]
                  tunnel: w2203 -> [w2240]
                  tunnel: [w2239] -> w2201
                  tunnel: [w2246] -> w2200
                  tunnel: w2202 -> [w2246]
                  tunnel: [w2245] -> w2199
                  tunnel: w2201 -> [w2245]
                  tunnel: w2178 -> [w2244]
                  tunnel: w2200 -> [w2253]
                  tunnel: w2199 -> [w2252]
                  tunnel: [w2248] -> w2198
                  tunnel: [w2247] -> w2197
                  tunnel: w2198 -> [w2256]
                  tunnel: [w2256] -> w2196
                  tunnel: w2197 -> [w2255]
                  tunnel: [w2255] -> w2195
                  tunnel: w2178 -> [w2254]
                  tunnel: w2196 -> [w2260]
                  tunnel: w2195 -> [w2259]
                  frame #0 {
                    n1274 = VISA Write(VISA resource name=w2219, write buffer=w2215, error in (no error)=w2217) -> (VISA resource name out=w2218:refnum<visa-resource-name>, error out=w2216:errorcluster)  [unwired: 1 out]
                  }
                  frame #1 {
                    n1275 = Wait (ms)(milliseconds to wait=w2220) -> ()  [unwired: 1 out]
                  }
                  frame #2 {
                    n1276 = VISA Write(VISA resource name=w2225, write buffer=w2226, error in (no error)=w2224) -> (VISA resource name out=w2227:refnum<visa-resource-name>, error out=w2223:errorcluster)  [unwired: 1 out]
                  }
                  frame #3 {
                    n1277 = Wait (ms)(milliseconds to wait=w2228) -> ()  [unwired: 1 out]
                  }
                  frame #4 {
                    n1278 = VISA Write(VISA resource name=w2235, write buffer=w2233, error in (no error)=w2232) -> (VISA resource name out=w2234:refnum<visa-resource-name>, error out=w2231:errorcluster)  [unwired: 1 out]
                  }
                  frame #5 {
                    n1279 = Wait (ms)(milliseconds to wait=w2236) -> ()  [unwired: 1 out]
                  }
                  frame #6 {
                    n1280 = VISA Write(VISA resource name=w2243, write buffer=w2241, error in (no error)=w2240) -> (VISA resource name out=w2242:refnum<visa-resource-name>, error out=w2239:errorcluster)  [unwired: 1 out]
                  }
                  frame #7 {
                    n1281 = Wait (ms)(milliseconds to wait=w2244) -> ()  [unwired: 1 out]
                  }
                  frame #8 {
                    n1282 = Concatenate Strings("start ", "\r") -> (w2251:string)
                    n1283 = VISA Write(VISA resource name=w2253, write buffer=w2251, error in (no error)=w2252) -> (VISA resource name out=w2248:refnum<visa-resource-name>, error out=w2247:errorcluster)  [unwired: 1 out]
                  }
                  frame #9 {
                    n1284 = Wait (ms)(milliseconds to wait=w2254) -> ()  [unwired: 1 out]
                  }
                  frame #10 {
                    n1285 = Concatenate Strings("enter main ", "\r") -> (w2261:string)
                    n1286 = VISA Write(VISA resource name=w2260, write buffer=w2261, error in (no error)=w2259) -> (VISA resource name out=w2258:refnum<visa-resource-name>, error out=w2257:errorcluster)  [unwired: 1 out]
                    n1287 = VISA Close(VISA resource name=w2258, error in (no error)=w2257) -> ()  [unwired: 1 out]
                  }
                }
                n1288 = Concatenate Strings("enter pump1", w2194) -> (w2193:string)
                n1289 = local read "Normal \nRate (ul/hr)"() -> (w2179:dbl)
                n1290 = Concatenate Strings("set units 4 ", w2194) -> (w2190:string)
                n1291 = local read "Normal \nVolume (ul)"() -> (w2180:dbl)
                n1292 = Number To Decimal String(number=w2179) -> (decimal integer string=w2189:string)  [unwired: 1 in]
                n1293 = Concatenate Strings("set rate ", w2189, w2194) -> (w2187:string)
                n1294 = Number To Decimal String(number=w2180) -> (decimal integer string=w2185:string)  [unwired: 1 in]
                n1295 = Concatenate Strings("set volume ", w2185, w2194) -> (w2184:string)
              }
            }
          }
          event "Normal \nVolume (ul)": Value Change {
            n1296 = event-data() -> ()  [unwired: 1 in, 5 out]
            n1297 = call-poly "VISA Configure Serial Port"("VISA resource name"=w2279) -> ("VISA resource name out"=w2281:refnum<visa-resource-name>, "error out"=w2280:errorcluster)  [unwired: 13 in]
            n1298 = local read "Write Wait"() -> (w2264:i32)
            n1299 = Concatenate Strings("enter pump1", "\r") -> (w2283:string)
            n1300 = flat-sequence {
              tunnel: w2280 -> [w2293]
              tunnel: w2281 -> [w2295]
              tunnel: [w2294] -> w2273
              tunnel: [w2292] -> w2272
              tunnel: w2283 -> [w2291]
              tunnel: w2273 -> [w2298]
              tunnel: [w2298] -> w2271
              tunnel: w2272 -> [w2297]
              tunnel: [w2297] -> w2269
              tunnel: w2264 -> [w2296]
              tunnel: w2271 -> [w2302]
              tunnel: [w2303] -> w2270
              tunnel: w2269 -> [w2301]
              tunnel: [w2300] -> w2268
              tunnel: w2265 -> [w2299]
              tunnel: w2270 -> [w2306]
              tunnel: w2268 -> [w2305]
              tunnel: [w2306] -> w2290
              tunnel: [w2305] -> w2289
              tunnel: w2264 -> [w2304]
              tunnel: [w2311] -> w2288
              tunnel: [w2310] -> w2287
              tunnel: w2290 -> [w2309]
              tunnel: w2289 -> [w2308]
              tunnel: w2274 -> [w2307]
              tunnel: w2288 -> [w2314]
              tunnel: [w2314] -> w2286
              tunnel: w2287 -> [w2313]
              tunnel: [w2313] -> w2285
              tunnel: w2264 -> [w2312]
              tunnel: w2286 -> [w2318]
              tunnel: w2285 -> [w2317]
              frame #0 {
                n1301 = VISA Write(VISA resource name=w2295, write buffer=w2291, error in (no error)=w2293) -> (VISA resource name out=w2294:refnum<visa-resource-name>, error out=w2292:errorcluster)  [unwired: 1 out]
              }
              frame #1 {
                n1302 = Wait (ms)(milliseconds to wait=w2296) -> ()  [unwired: 1 out]
              }
              frame #2 {
                n1303 = VISA Write(VISA resource name=w2302, write buffer=w2299, error in (no error)=w2301) -> (VISA resource name out=w2303:refnum<visa-resource-name>, error out=w2300:errorcluster)  [unwired: 1 out]
              }
              frame #3 {
                n1304 = Wait (ms)(milliseconds to wait=w2304) -> ()  [unwired: 1 out]
              }
              frame #4 {
                n1305 = VISA Write(VISA resource name=w2309, write buffer=w2307, error in (no error)=w2308) -> (VISA resource name out=w2311:refnum<visa-resource-name>, error out=w2310:errorcluster)  [unwired: 1 out]
              }
              frame #5 {
                n1306 = Wait (ms)(milliseconds to wait=w2312) -> ()  [unwired: 1 out]
              }
              frame #6 {
                n1307 = Concatenate Strings("enter main ", "\r") -> (w2319:string)
                n1308 = VISA Write(VISA resource name=w2318, write buffer=w2319, error in (no error)=w2317) -> (VISA resource name out=w2316:refnum<visa-resource-name>, error out=w2315:errorcluster)  [unwired: 1 out]
                n1309 = VISA Close(VISA resource name=w2316, error in (no error)=w2315) -> ()  [unwired: 1 out]
              }
            }
            n1310 = Concatenate Strings("set units 4", "\r") -> (w2265:string)
            n1311 = Number To Decimal String(number="Normal \nVolume (ul)") -> (decimal integer string=w2276:string)  [unwired: 1 in]
            n1312 = Concatenate Strings("set volume", w2276, "\r") -> (w2274:string)
          }
          event "Normal \nRate (ul/hr)": Value Change {
            n1313 = event-data() -> ()  [unwired: 1 in, 5 out]
            n1314 = call-poly "VISA Configure Serial Port"("VISA resource name"=w2324) -> ("VISA resource name out"=w2332:refnum<visa-resource-name>, "error out"=w2331:errorcluster)  [unwired: 13 in]
            n1315 = local read "Write Wait"() -> (w2322:i32)
            n1316 = Concatenate Strings("enter pump1", "\r") -> (w2334:string)
            n1317 = flat-sequence {
              tunnel: w2331 -> [w2351]
              tunnel: w2332 -> [w2353]
              tunnel: [w2352] -> w2347
              tunnel: [w2350] -> w2346
              tunnel: w2334 -> [w2349]
              tunnel: w2347 -> [w2356]
              tunnel: [w2356] -> w2345
              tunnel: w2346 -> [w2355]
              tunnel: [w2355] -> w2344
              tunnel: w2322 -> [w2354]
              tunnel: w2345 -> [w2360]
              tunnel: [w2361] -> w2343
              tunnel: w2344 -> [w2359]
              tunnel: [w2358] -> w2342
              tunnel: w2325 -> [w2357]
              tunnel: w2343 -> [w2364]
              tunnel: w2342 -> [w2363]
              tunnel: [w2364] -> w2341
              tunnel: [w2363] -> w2340
              tunnel: w2322 -> [w2362]
              tunnel: [w2369] -> w2339
              tunnel: [w2368] -> w2338
              tunnel: w2341 -> [w2367]
              tunnel: w2340 -> [w2366]
              tunnel: w2328 -> [w2365]
              tunnel: w2339 -> [w2372]
              tunnel: [w2372] -> w2337
              tunnel: w2338 -> [w2371]
              tunnel: [w2371] -> w2336
              tunnel: w2322 -> [w2370]
              tunnel: w2337 -> [w2376]
              tunnel: w2336 -> [w2375]
              frame #0 {
                n1318 = VISA Write(VISA resource name=w2353, write buffer=w2349, error in (no error)=w2351) -> (VISA resource name out=w2352:refnum<visa-resource-name>, error out=w2350:errorcluster)  [unwired: 1 out]
              }
              frame #1 {
                n1319 = Wait (ms)(milliseconds to wait=w2354) -> ()  [unwired: 1 out]
              }
              frame #2 {
                n1320 = VISA Write(VISA resource name=w2360, write buffer=w2357, error in (no error)=w2359) -> (VISA resource name out=w2361:refnum<visa-resource-name>, error out=w2358:errorcluster)  [unwired: 1 out]
              }
              frame #3 {
                n1321 = Wait (ms)(milliseconds to wait=w2362) -> ()  [unwired: 1 out]
              }
              frame #4 {
                n1322 = VISA Write(VISA resource name=w2367, write buffer=w2365, error in (no error)=w2366) -> (VISA resource name out=w2369:refnum<visa-resource-name>, error out=w2368:errorcluster)  [unwired: 1 out]
              }
              frame #5 {
                n1323 = Wait (ms)(milliseconds to wait=w2370) -> ()  [unwired: 1 out]
              }
              frame #6 {
                n1324 = Concatenate Strings("enter main ", "\r") -> (w2377:string)
                n1325 = VISA Write(VISA resource name=w2376, write buffer=w2377, error in (no error)=w2375) -> (VISA resource name out=w2374:refnum<visa-resource-name>, error out=w2373:errorcluster)  [unwired: 1 out]
                n1326 = VISA Close(VISA resource name=w2374, error in (no error)=w2373) -> ()  [unwired: 1 out]
              }
            }
            n1327 = Concatenate Strings("set units 4", "\r") -> (w2325:string)
            n1328 = Number To Decimal String(number="Normal \nRate (ul/hr)") -> (decimal integer string=w2323:string)  [unwired: 1 in]
            n1329 = Concatenate Strings("set rate", w2323, "\r") -> (w2328:string)
          }
          event "Normal \nRate (ul/hr)  2": Value Change {
            n1330 = event-data() -> ()  [unwired: 1 in, 5 out]
            n1331 = call-poly "VISA Configure Serial Port"("VISA resource name"=w2382) -> ("VISA resource name out"=w2390:refnum<visa-resource-name>, "error out"=w2389:errorcluster)  [unwired: 13 in]
            n1332 = local read "Write Wait"() -> (w2380:i32)
            n1333 = Concatenate Strings("enter pump2", "\r") -> (w2392:string)
            n1334 = flat-sequence {
              tunnel: w2389 -> [w2409]
              tunnel: w2390 -> [w2411]
              tunnel: [w2410] -> w2405
              tunnel: [w2408] -> w2404
              tunnel: w2392 -> [w2407]
              tunnel: w2405 -> [w2414]
              tunnel: [w2414] -> w2403
              tunnel: w2404 -> [w2413]
              tunnel: [w2413] -> w2402
              tunnel: w2380 -> [w2412]
              tunnel: w2403 -> [w2418]
              tunnel: [w2419] -> w2401
              tunnel: w2402 -> [w2417]
              tunnel: [w2416] -> w2400
              tunnel: w2383 -> [w2415]
              tunnel: w2401 -> [w2422]
              tunnel: w2400 -> [w2421]
              tunnel: [w2422] -> w2399
              tunnel: [w2421] -> w2398
              tunnel: w2380 -> [w2420]
              tunnel: [w2427] -> w2397
              tunnel: [w2426] -> w2396
              tunnel: w2399 -> [w2425]
              tunnel: w2398 -> [w2424]
              tunnel: w2386 -> [w2423]
              tunnel: w2397 -> [w2430]
              tunnel: [w2430] -> w2395
              tunnel: w2396 -> [w2429]
              tunnel: [w2429] -> w2394
              tunnel: w2380 -> [w2428]
              tunnel: w2395 -> [w2434]
              tunnel: w2394 -> [w2433]
              frame #0 {
                n1335 = VISA Write(VISA resource name=w2411, write buffer=w2407, error in (no error)=w2409) -> (VISA resource name out=w2410:refnum<visa-resource-name>, error out=w2408:errorcluster)  [unwired: 1 out]
              }
              frame #1 {
                n1336 = Wait (ms)(milliseconds to wait=w2412) -> ()  [unwired: 1 out]
              }
              frame #2 {
                n1337 = VISA Write(VISA resource name=w2418, write buffer=w2415, error in (no error)=w2417) -> (VISA resource name out=w2419:refnum<visa-resource-name>, error out=w2416:errorcluster)  [unwired: 1 out]
              }
              frame #3 {
                n1338 = Wait (ms)(milliseconds to wait=w2420) -> ()  [unwired: 1 out]
              }
              frame #4 {
                n1339 = VISA Write(VISA resource name=w2425, write buffer=w2423, error in (no error)=w2424) -> (VISA resource name out=w2427:refnum<visa-resource-name>, error out=w2426:errorcluster)  [unwired: 1 out]
              }
              frame #5 {
                n1340 = Wait (ms)(milliseconds to wait=w2428) -> ()  [unwired: 1 out]
              }
              frame #6 {
                n1341 = Concatenate Strings("enter main ", "\r") -> (w2435:string)
                n1342 = VISA Write(VISA resource name=w2434, write buffer=w2435, error in (no error)=w2433) -> (VISA resource name out=w2432:refnum<visa-resource-name>, error out=w2431:errorcluster)  [unwired: 1 out]
                n1343 = VISA Close(VISA resource name=w2432, error in (no error)=w2431) -> ()  [unwired: 1 out]
              }
            }
            n1344 = Concatenate Strings("set units 4", "\r") -> (w2383:string)
            n1345 = Number To Decimal String(number="Normal \nRate (ul/hr)  2") -> (decimal integer string=w2381:string)  [unwired: 1 in]
            n1346 = Concatenate Strings("set rate", w2381, "\r") -> (w2386:string)
          }
          event "Normal \nVolume (ul) 2": Value Change {
            n1347 = event-data() -> ()  [unwired: 1 in, 5 out]
            n1348 = call-poly "VISA Configure Serial Port"("VISA resource name"=w2441) -> ("VISA resource name out"=w2445:refnum<visa-resource-name>, "error out"=w2446:errorcluster)  [unwired: 13 in]
            n1349 = local read "Write Wait"() -> (w2438:i32)
            n1350 = Concatenate Strings("enter pump2", "\r") -> (w2443:string)
            n1351 = flat-sequence {
              tunnel: w2446 -> [w2467]
              tunnel: w2445 -> [w2469]
              tunnel: [w2468] -> w2464
              tunnel: [w2466] -> w2463
              tunnel: w2443 -> [w2465]
              tunnel: w2464 -> [w2472]
              tunnel: [w2472] -> w2462
              tunnel: w2463 -> [w2471]
              tunnel: [w2471] -> w2461
              tunnel: w2438 -> [w2470]
              tunnel: w2462 -> [w2476]
              tunnel: [w2477] -> w2460
              tunnel: w2461 -> [w2475]
              tunnel: [w2474] -> w2459
              tunnel: w2452 -> [w2473]
              tunnel: w2460 -> [w2480]
              tunnel: w2459 -> [w2479]
              tunnel: [w2480] -> w2458
              tunnel: [w2479] -> w2457
              tunnel: w2438 -> [w2478]
              tunnel: [w2485] -> w2456
              tunnel: [w2484] -> w2455
              tunnel: w2458 -> [w2483]
              tunnel: w2457 -> [w2482]
              tunnel: w2449 -> [w2481]
              tunnel: w2456 -> [w2488]
              tunnel: [w2488] -> w2454
              tunnel: w2455 -> [w2487]
              tunnel: [w2487] -> w2453
              tunnel: w2438 -> [w2486]
              tunnel: w2454 -> [w2492]
              tunnel: w2453 -> [w2491]
              frame #0 {
                n1352 = VISA Write(VISA resource name=w2469, write buffer=w2465, error in (no error)=w2467) -> (VISA resource name out=w2468:refnum<visa-resource-name>, error out=w2466:errorcluster)  [unwired: 1 out]
              }
              frame #1 {
                n1353 = Wait (ms)(milliseconds to wait=w2470) -> ()  [unwired: 1 out]
              }
              frame #2 {
                n1354 = VISA Write(VISA resource name=w2476, write buffer=w2473, error in (no error)=w2475) -> (VISA resource name out=w2477:refnum<visa-resource-name>, error out=w2474:errorcluster)  [unwired: 1 out]
              }
              frame #3 {
                n1355 = Wait (ms)(milliseconds to wait=w2478) -> ()  [unwired: 1 out]
              }
              frame #4 {
                n1356 = VISA Write(VISA resource name=w2483, write buffer=w2481, error in (no error)=w2482) -> (VISA resource name out=w2485:refnum<visa-resource-name>, error out=w2484:errorcluster)  [unwired: 1 out]
              }
              frame #5 {
                n1357 = Wait (ms)(milliseconds to wait=w2486) -> ()  [unwired: 1 out]
              }
              frame #6 {
                n1358 = Concatenate Strings("enter main ", "\r") -> (w2493:string)
                n1359 = VISA Write(VISA resource name=w2492, write buffer=w2493, error in (no error)=w2491) -> (VISA resource name out=w2490:refnum<visa-resource-name>, error out=w2489:errorcluster)  [unwired: 1 out]
                n1360 = VISA Close(VISA resource name=w2490, error in (no error)=w2489) -> ()  [unwired: 1 out]
              }
            }
            n1361 = Concatenate Strings("set units 4", "\r") -> (w2452:string)
            n1362 = Number To Decimal String(number="Normal \nVolume (ul) 2") -> (decimal integer string=w2439:string)  [unwired: 1 in]
            n1363 = Concatenate Strings("set volume", w2439, "\r") -> (w2449:string)
          }
        }
        n1364 = node-c288() -> ()  [unwired: 1 in, 1 out]
      }
      n1365 = node-c288(w1825) -> ()  [unwired: 1 out]
    }
    frame Enabled {
      n1366 = node-c288(2 ("Processor")) -> (w2505:T11)  [unwired: 3 in]
      n1367 = timed-loop "Pump Control" {
        timing: w2505 -> [_]
        timing-out: [_] -> w2504
        tunnel: refnum<visa-resource-name> "COM4" ("VISA resource name") -> [w2507]
        stop <- w2506 stop-if-true
        n1368 = node-c288() -> ()  [unwired: 1 in, 1 out]
        n1369 = event shown="[2] \"Inject Sample\": Value Change" {
          selector: _ -> [_ _ _ _ _]
          dyn-events: _ -> [_ _ _ _ _]
          timeout: _ -> [_ _ _ _ _]
          tunnel: w2507 -> [w2513 _ w2587 w2614 w2619]
          tunnel: [_ w2585 _ _ _] -> w2506
          event "Flush Sample": Value Change {
            n1370 = event-data() -> ()  [unwired: 1 in, 5 out]
            n1371 = local read "Write Wait"() -> (w2527:i32)
            n1372 = flat-sequence {
              tunnel: [w2551] -> w2547
              tunnel: [w2550] -> w2546
              tunnel: "CLD" -> [w2549]
              tunnel: w2513 -> [w2548]
              tunnel: w2547 -> [w2554]
              tunnel: [w2554] -> w2545
              tunnel: w2546 -> [w2553]
              tunnel: [w2553] -> w2544
              tunnel: w2527 -> [w2552]
              tunnel: [w2559] -> w2543
              tunnel: [w2556] -> w2542
              tunnel: w2545 -> [w2558]
              tunnel: w2544 -> [w2557]
              tunnel: "MODVOL" -> [w2555]
              tunnel: w2543 -> [w2562]
              tunnel: [w2562] -> w2541
              tunnel: [w2561] -> w2540
              tunnel: w2542 -> [w2561]
              tunnel: w2527 -> [w2560]
              tunnel: w2541 -> [w2567]
              tunnel: [w2566] -> w2539
              tunnel: w2529 -> [w2565]
              tunnel: w2540 -> [w2564]
              tunnel: [w2563] -> w2538
              tunnel: w2539 -> [w2570]
              tunnel: [w2570] -> w2537
              tunnel: [w2569] -> w2536
              tunnel: w2538 -> [w2569]
              tunnel: w2527 -> [w2568]
              tunnel: w2537 -> [w2575]
              tunnel: [w2574] -> w2535
              tunnel: w2531 -> [w2573]
              tunnel: w2536 -> [w2572]
              tunnel: [w2571] -> w2534
              tunnel: [w2578] -> w2532
              tunnel: w2535 -> [w2578]
              tunnel: [w2577] -> w2533
              tunnel: w2534 -> [w2577]
              tunnel: w2527 -> [w2576]
              tunnel: w2533 -> [w2583]
              tunnel: w2532 -> [w2584]
              tunnel: [w2582] -> w2522
              tunnel: "RUN " -> [w2581]
              frame #0 {
                n1373 = call "Write to pump 2.vi"("String to write"=w2549, "VISA resource name"=w2548) -> ("error out"=w2550:errorcluster, "VISA resource name out"=w2551:refnum<visa-resource-name>)  [unwired: 8 in]
              }
              frame #1 {
                n1374 = Wait (ms)(milliseconds to wait=w2552) -> ()  [unwired: 1 out]
              }
              frame #2 {
                n1375 = call "Write to pump 2.vi"("error in (no error)"=w2557, "String to write"=w2555, "VISA resource name"=w2558) -> ("error out"=w2556:errorcluster, "VISA resource name out"=w2559:refnum<visa-resource-name>)  [unwired: 7 in]
              }
              frame #3 {
                n1376 = Wait (ms)(milliseconds to wait=w2560) -> ()  [unwired: 1 out]
              }
              frame #4 {
                n1377 = call "Write to pump 2.vi"("error in (no error)"=w2564, "String to write"=w2565, "VISA resource name"=w2567) -> ("error out"=w2563:errorcluster, "VISA resource name out"=w2566:refnum<visa-resource-name>)  [unwired: 7 in]
              }
              frame #5 {
                n1378 = Wait (ms)(milliseconds to wait=w2568) -> ()  [unwired: 1 out]
              }
              frame #6 {
                n1379 = call "Write to pump 2.vi"("error in (no error)"=w2572, "String to write"=w2573, "VISA resource name"=w2575) -> ("error out"=w2571:errorcluster, "VISA resource name out"=w2574:refnum<visa-resource-name>)  [unwired: 7 in]
              }
              frame #7 {
                n1380 = Wait (ms)(milliseconds to wait=w2576) -> ()  [unwired: 1 out]
              }
              frame #8 {
                w2580 = TRUE ("Inject Pump 3")
                n1381 = Tick Count (ms)() -> (millisecond timer value=→"Flush Sample Start Time":u32)
                n1382 = call "Write to pump 2.vi"("error in (no error)"=w2583, "String to write"=w2581, "VISA resource name"=w2584) -> ("error out"=w2582:errorcluster)  [unwired: 7 in, 1 out]
                n1383 = local write "Inject Sample"(w2580) -> ()
                "Flushing Sample" <- w2580
              }
            }
            n1384 = Number To Fractional String(number="Flush \nRate (ul/min)  3") -> (F-format string=w2515:string)  [unwired: 3 in]
            n1385 = String Subset(string=w2515, length (rest)=6 ("length (rest)")) -> (substring=w2514:string)  [unwired: 1 in]
            n1386 = Concatenate Strings("RAT", w2514, "UM") -> (w2529:string)
            n1387 = Divide(x="Flush\nVolume (ul)  3", y=1000.0) -> (x/y=w2520:dbl)
            n1388 = Number To Fractional String(number=w2520) -> (F-format string=w2519:string)  [unwired: 3 in]
            n1389 = Divide(x="Flush\nVolume (ul)  3", y="Flush \nRate (ul/min)  3") -> (x/y=w2510:dbl)
            n1390 = Multiply(x=w2510, y=60.0) -> (x*y=→"Sample flush time (s)":dbl)
            n1391 = String Subset(string=w2519, length (rest)=6 ("length (rest)")) -> (substring=w2518:string)  [unwired: 1 in]
            n1392 = Concatenate Strings("TGT", w2518) -> (w2531:string)
            "error out" <- w2522
          }
          event "Stop": Value Change {
            n1393 = event-data() -> ()  [unwired: 1 in, 5 out]
            n1394 = local read "Stop"() -> (w2585:bool)
          }
          event "Inject Sample": Value Change {
            n1395 = event-data() -> ()  [unwired: 1 in, 5 out]
            n1396 = case shown="True" "Inject Sample" {
              tunnel: w2587 -> [w2589 w2590]
              frame False {
                n1397 = call "Write to pump 2.vi"("String to write"="STP", "VISA resource name"=w2589) -> ()  [unwired: 8 in, 2 out]
              }
              frame True {
                n1398 = local read "Normal \nRate (ul/hr)  3"() -> (w2591:dbl)
                n1399 = Number To Fractional String(number=w2591) -> (F-format string=w2594:string)  [unwired: 3 in]
                n1400 = String Subset(string=w2594, length (rest)=6 ("length (rest)")) -> (substring=w2592:string)  [unwired: 1 in]
                n1401 = flat-sequence {
                  tunnel: "RUN " -> [w2606]
                  tunnel: [w2608] -> _
                  tunnel: [w2607] -> _
                  tunnel: w2590 -> [w2605]
                  frame #0 {
                    n1402 = call "Write to pump 2.vi"("String to write"=w2606, "VISA resource name"=w2605) -> ("error out"=w2607:errorcluster, "VISA resource name out"=w2608:refnum<visa-resource-name>)  [unwired: 8 in]
                  }
                }
                n1403 = Concatenate Strings("RAT", w2592, "UH" ("string")) -> ()  [unwired: 1 out]
                n1404 = local read "Normal \nVolume (ul) 3"() -> (w2600:dbl)
                n1405 = Divide(x=w2600, y=1000.0) -> (x/y=w2595:dbl)
                n1406 = Number To Fractional String(number=w2595) -> (F-format string=w2598:string)  [unwired: 3 in]
                n1407 = String Subset(string=w2598, length (rest)=6 ("length (rest)")) -> (substring=w2596:string)  [unwired: 1 in]
                n1408 = Concatenate Strings("TGT", w2596) -> ()  [unwired: 1 out]
              }
            }
          }
          event "Normal \nRate (ul/hr)  3": Value Change {
            n1409 = event-data() -> ()  [unwired: 1 in, 5 out]
            n1410 = Number To Fractional String(number="Normal \nRate (ul/hr)  3") -> (F-format string=w2612:string)  [unwired: 3 in]
            n1411 = String Subset(string=w2612, length (rest)=6 ("length (rest)")) -> (substring=w2610:string)  [unwired: 1 in]
            n1412 = Concatenate Strings("RAT", w2610, "UH") -> (w2613:string)
            n1413 = call "Write to pump 2.vi"("String to write"=w2613, "VISA resource name"=w2614) -> ()  [unwired: 8 in, 2 out]
          }
          event "Clear Volume": Value Change {
            n1414 = event-data() -> ()  [unwired: 1 in, 5 out]
            n1415 = Divide(x="Normal \nVolume (ul) 3", y=1000.0) -> (x/y=w2632:dbl)
            n1416 = Number To Fractional String(number=w2632) -> (F-format string=w2635:string)  [unwired: 3 in]
            n1417 = String Subset(string=w2635, length (rest)=6 ("length (rest)")) -> (substring=w2633:string)  [unwired: 1 in]
            n1418 = flat-sequence {
              tunnel: [w2642] -> w2630
              tunnel: [w2641] -> w2629
              tunnel: w2619 -> [w2640]
              tunnel: w2618 -> [w2639]
              tunnel: [w2644] -> w2627
              tunnel: [w2643] -> w2628
              tunnel: w2624 -> [w2645]
              tunnel: w2630 -> [w2644]
              tunnel: w2629 -> [w2643]
              tunnel: w2628 -> [w2649]
              tunnel: w2627 -> [w2650]
              tunnel: [w2648] -> _
              tunnel: [w2647] -> _
              tunnel: w2617 -> [w2646]
              frame #0 {
                n1419 = call "Write to pump 2.vi"("String to write"=w2639, "VISA resource name"=w2640) -> ("error out"=w2641:errorcluster, "VISA resource name out"=w2642:refnum<visa-resource-name>)  [unwired: 8 in]
              }
              frame #1 {
                n1420 = Wait (ms)(milliseconds to wait=w2645) -> ()  [unwired: 1 out]
              }
              frame #2 {
                n1421 = call "Write to pump 2.vi"("error in (no error)"=w2649, "String to write"=w2646, "VISA resource name"=w2650) -> ("error out"=w2647:errorcluster, "VISA resource name out"=w2648:refnum<visa-resource-name>)  [unwired: 7 in]
              }
            }
            n1422 = local read "Write Wait"() -> (w2624:i32)
            n1423 = Concatenate Strings("TGT", w2633) -> (w2618:string)
            n1424 = local read "Normal \nRate (ul/hr)  3"() -> (w2620:dbl)
            n1425 = local write "Clear Volume"(FALSE ("Clear Volume")) -> ()
            n1426 = Number To Fractional String(number=w2620) -> (F-format string=w2623:string)  [unwired: 3 in]
            n1427 = String Subset(string=w2623, length (rest)=6 ("length (rest)")) -> (substring=w2621:string)  [unwired: 1 in]
            n1428 = Concatenate Strings("RAT", w2621, "UH" ("string")) -> (w2617:string)
          }
        }
        n1429 = node-c288() -> ()  [unwired: 1 in, 1 out]
      }
      n1430 = node-c288(w2504) -> ()  [unwired: 1 out]
    }
  }
  n1431 = node-c288() -> (w80:T11)  [unwired: 4 in]
  n1432 = timed-loop {
    timing: w80 -> [_]
    timing-out: [_] -> w79
    stop <- w2657 stop-if-true
    n1433 = node-c288() -> ()  [unwired: 1 in, 1 out]
    n1434 = event shown="[1] \"Stop\": Value Change" {
      selector: _ -> [_ _]
      dyn-events: _ -> [_ _]
      timeout: _ -> [_ _]
      tunnel: [_ "Stop"] -> w2657
      event Timeout {
        n1435 = event-data() -> ()  [unwired: 1 in, 2 out]
      }
      event "Stop": Value Change {
        n1436 = event-data() -> ()  [unwired: 1 in, 4 out]
        n1437 = property on="Cancel dwell" class="Bool (strict)"("Val(Sgnl)"=TRUE ("Value (Signaling)")) -> ()  [unwired: 2 in, 2 out]
        n1438 = local write "Force Feedback"(FALSE ("Force Feedback")) -> ()
      }
    }
    n1439 = node-c288() -> ()  [unwired: 1 in, 1 out]
  }
  n1440 = case shown="True" w69 {
    tunnel: w74 -> [_ w2665]
    tunnel: w73 -> [_ w2664]
    tunnel: w72 -> [_ w2663]
    frame False {
    }
    frame True {
      w2667 = T19 3 items=["no dialog", "OK message", "continue or stop message", "OK message + warnings", "continue/stop + warnings"] ("type of dialog (OK msg:1)")
      w2666 = T19 3 items=["no dialog", "OK message", "continue or stop message", "OK message + warnings", "continue/stop + warnings"] ("type of dialog (OK msg:1)")
      n1441 = call <vilib>:"DAQmx Clear Task.vi"("task in"=w2665, "error in"=w2663) -> ("error out"=w2668:errorcluster)  [unwired: 13 in]
      n1442 = call <vilib>:"DAQmx Clear Task.vi"("task in"=w2664) -> ("error out"=w2669:errorcluster)  [unwired: 14 in]
      n1443 = call <vilib>:"Simple Error Handler.vi"("type of dialog (OK msg:1)"=w2667, "error in (no error)"=w2668) -> ()  [unwired: 3 in, 5 out]
      n1444 = call <vilib>:"Simple Error Handler.vi"("type of dialog (OK msg:1)"=w2666, "error in (no error)"=w2669) -> ()  [unwired: 3 in, 5 out]
    }
  }
  n1445 = case shown="\"Force Feedback\", Default" "?" {
    frame "Force Feedback", Default {
    }
    frame "Raster scan" {
    }
  }
  n1446 = node-c288(w79) -> ()  [unwired: 1 out]
  n1447 = node-c288(w82) -> ()  [unwired: 1 out]
  n1448 = local write "Pause Mouse/Mirror Connection"(FALSE ("Pause Mouse/Mirror Connection")) -> ()
  n1449 = local write "Stop"(FALSE ("Stop all")) -> ()
  "CoordinatesMousePressed" <- T5 {"Horizontal"=0, "Vertical"=0} ("Coords when pressed")
  "Deflection" <- T5 {"Horizontal"=0, "Vertical"=0} ("Coords when pressed")
